vi "minimal_test_startup.vi"   [LabVIEW 2013, in "main.lvlib"]
uses:
  main.lvlib
  Controls/Enum Variables.ctl
  Controls/Enum Save Action Events.ctl
  Controls/Enum Paper Action Events.ctl
  Controls/Enum Process Data.ctl
  Controls/Enum DICOM.ctl
  Controls/Enum User Events.ctl
  New Design/Controls/Reference AE Control.ctl
  Controls/SaveDataCluster.ctl
  Controls/Combobox Filename.ctl
  <vilib>/Utility/error.llb/DialogTypeEnum.ctl
  Components/TypeDef - SHIFTER.ctl
  New Design/Menu/Top Menu.vi
  New Design/Profile/Profile.vi
  New Design/Configuration/Configuration.vi
  New Design/Acquisition/Acquisition.vi
  New Design/Data/Data.vi
  New Design/Journal/Journal.vi
  <userlib>/_MGI/Error Handling/MGI Suppress Error Code/MGI Suppress Error Code (Scalar).vi
  Acquisition/RefData(SubVI).vi
  Globals/DataPathGlobalVariable.vi
  <userlib>/_OpenG.lib/file/file.llb/File Exists - Scalar__ogtk.vi
  Globals/DataAcqRecordPathGlobal.vi
  <vilib>/Utility/file.llb/Write To Spreadsheet File (string).vi
  <userlib>/_OpenG.lib/error/error.llb/Filter Error Codes (Array)__ogtk.vi
  <vilib>/Utility/file.llb/Read From Spreadsheet File (DBL).vi
  <vilib>/Utility/file.llb/Write To Spreadsheet File (DBL).vi
  <vilib>/Utility/file.llb/Read From Spreadsheet File (string).vi
  <userlib>/_OpenG.lib/file/file.llb/Valid Path - Traditional__ogtk.vi
  <vilib>/regexp/Match Regular Expression.xnode
  Components/Dependencies.llb/TLB_Dependencies.lvlib
  Settings/Options/Options.vi
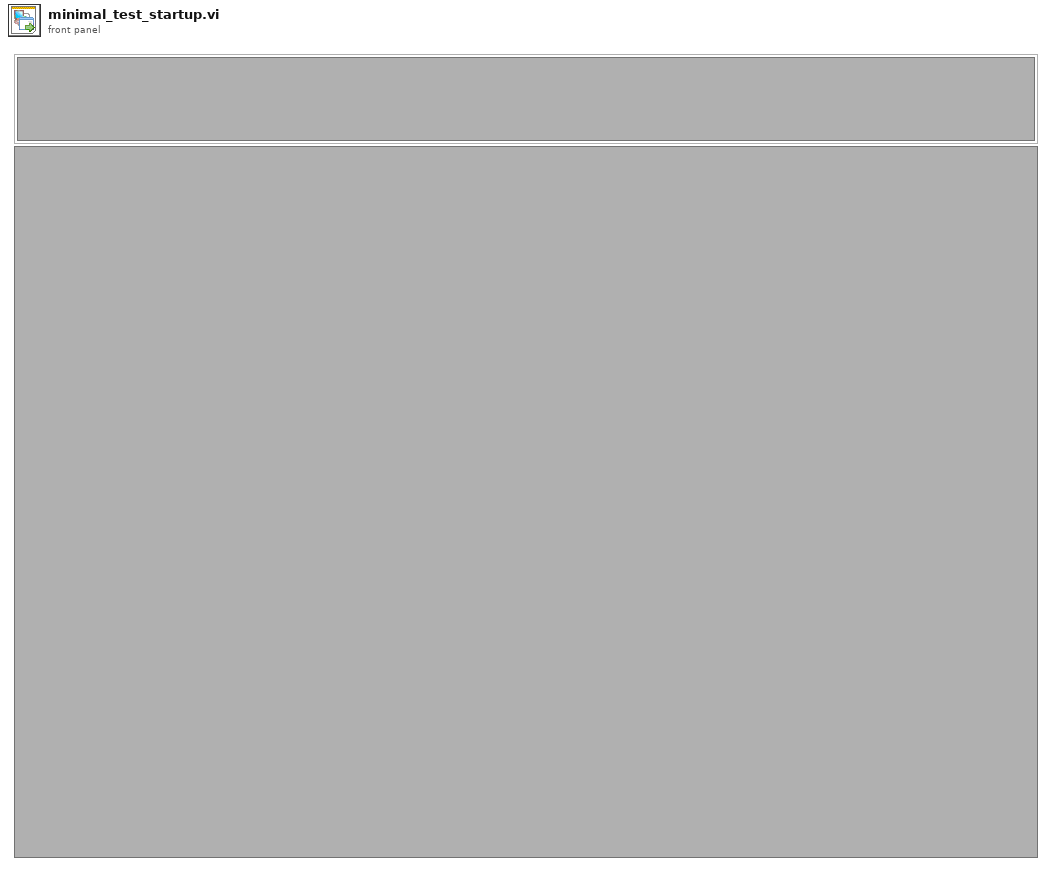
[diagram p1: front panel]
types:
  T1 = enum16{"Clear SR", "Set Display", "Set Shifter", "Initialize Events", "Init Q"}
  T2 = enum32{"Invalid", "Standard", "Closed", "Hidden", "Minimized", "Maximized"}
  T3 = typedef "main.lvlib/TypeDef - SHIFTER.ctl" = cluster{"Exit Event":T4, "Terminate Error":errorcluster, "User Parameter Controls":refnum<vi>[], "User Parameters":cluster{"Name":string, "CPR Number":string, "Measuring Type ":string, "Measuring Technique":string, "Measuring Limb":string, "Operator":string, "Doctor":string, "Comment":string, "AdditionalInfo":string, "RightArm":string[][], "LeftArm":string[][], "PalpationRight":string, "PalpationLeft":string, "Puls":dbl, "Temp One":dbl, "Temp Two":dbl, "ActivityBox":bool}, "System Parameters":cluster{"Paper Running?":bool, "GraphSelection":bool, "Date":string, "Active Page":string}, "Data Acquisition":cluster{"Acquisition":bool, "DAQmx Task":refnum<k21>, "DAQmx Error":errorcluster, "Record number":dbl, "RecordPath":path, "AcqDataRef":refnum<vi>, "Duration":timestamp, "Queue":refnum<queue>, "Control?":bool, "RelativeRecordPath":path}, "Reference signal":cluster{"DAQmx  Task ":refnum<k21>, "Monitor":bool, "Events":dbl, "Time":timestamp, "NullEvents":dbl, "RefDataRef":refnum<vi>, "Queue":refnum<queue>}, "Data Process":cluster{"SubpanelRef":refnum<vi>, "ActiveItemTag":string, "Queue":refnum<queue>}, "System Parameter Controls":refnum<vi>[], "Database":cluster{"PatientdataRef":refnum<file>, "PatientdataPath":path, "Blue Pressure":dbl, "Red Pressure":dbl, "ActiveItemTag":string, "Height Adjustment":dbl, "BluePositionArray":dbl[][], "RedPositionArray":dbl[][], "JournalPath":path}, "MWL":cluster{"PatientID":string, "Name":string, "DICOM Info":path, "DICOM Variables":string[], "Worklist":string[][]}, "Control":cluster{"Queue":refnum<queue>, "SignalCluster":cluster{"Pump":bool, "Finger":bool, "Ankle":bool, "Fast Def":bool, "Slow Def":bool, "Init Cal":bool, "Table Pres":bool, "Table":bool}}, "PageMenu":cluster{"VI Reference":refnum<vi>, "Queue":refnum<queue>}, "Profile":cluster{"VI Reference":refnum<vi>, "Queue":refnum<queue>}, "Configuration":cluster{"VI Reference":refnum<vi>, "Queue":refnum<queue>}, "Acquisition":cluster{"VI Reference":refnum<vi>, "Queue":refnum<queue>}, "Data":cluster{"VI Reference":refnum<vi>, "Queue":refnum<queue>}, "Journal":cluster{"VI Reference":refnum<vi>, "Queue":refnum<queue>}, "cRef":T5, "Bluetooth":cluster{"Queue":refnum<queue>, "VI Reference":refnum<vi>}}
  T4 = typedef "main.lvlib/TLB_Dependencies.lvlib/Exit Event Ref.ctl" = refnum<user-event>
  T5 = typedef "main.lvlib/Reference Cluster.ctl" = cluster{"Menu":cluster{"References":cluster{"Stop Acq":refnum<vi>, "MenuExit":refnum<vi>, "MenuStartADC":refnum<vi>, "PersonalInfoString":refnum<vi>, "Profile":refnum<vi>, "Configuration":refnum<vi>, "Acquisition":refnum<vi>, "Data":refnum<vi>, "Journal":refnum<vi>}}, "Profile":cluster{"References":cluster{"Search Patient ID":refnum<vi>, "Name":refnum<vi>, "CommentStr":refnum<vi>, "Listbox Patient ID":refnum<vi>, "ListboxDoctor":refnum<vi>, "ListboxOperator":refnum<vi>, "HospitalName":refnum<vi>, "HospitalDepartment":refnum<vi>, "HospitalAddress":refnum<vi>, "EditHospInfo":refnum<vi>, "Add Patient ID Btn":refnum<vi>, "Query Worklist":refnum<vi>}}, "Configuration":cluster{"References":cluster{"ListboxMeasurementArea":refnum<vi>, "ListboxMeasurementTechnique":refnum<vi>, "ListboxMeasurementMeth":refnum<vi>, "ListboxRightSegmentNr":refnum<vi>, "ListboxLeftSegmentNr":refnum<vi>, "HeightAdjustmentInt":refnum<vi>, "PalpationRight":refnum<vi>, "PalpationLeft":refnum<vi>, "ActivityBox":refnum<vi>}, "New method":cluster{"AddNewMeasurementBtn":refnum<vi>, "Left Time Table":refnum<vi>, "Right Time Table":refnum<vi>}, "Old method":cluster{"LeftArmPressureTable":refnum<vi>, "RightArmPressureTable":refnum<vi>, "SaveArmPressureBtn":refnum<vi>, "Puls":refnum<vi>, "TempTwo":refnum<vi>, "TempOne":refnum<vi>}, "Method":string}, "Acquisition":cluster{"References":cluster{"SegmentAcqString":refnum<vi>, "RingActGraph":refnum<vi>}}, "Data":cluster{"References":cluster{"cmString":refnum<vi>, "AdjustedHeight":refnum<vi>, "Menu":refnum<vi>, "Tangent On/Off":refnum<vi>, "FilterControl":refnum<vi>}}, "Journal":cluster{"References":cluster{"ReportSelection":refnum<vi>, "Data":refnum<vi>, "GenerateReport":refnum<vi>, "Menu":refnum<vi>, "Send To PACS":refnum<vi>}}}
  T6 = typedef "main.lvlib/TLB_Dependencies.lvlib/amc_Message Queue.ctl" = refnum<queue>
  T7 = typedef "main.lvlib/Enum Variables.ctl" = enum16{"SetAcqFilter", "GetAcqFilter", "Set Filter", "Get Filter", "Set Height", "Get Height", "Set Blue Pressure", "Get Blue Pressure", "Set Red Pressure", "Get Red Pressure", "Init", "Reset Pressure", "Set Red Cursors", "Get Red Cursors", "Set Blue Cursors", "Get Blue Cursors", "Set Language", "Get Language", "Set Active Graphs", "Get ActiveGraphs", "Set Method", "Get Method", "Set Encryption", "Get Encryption", "Set ExcelVersion", "Get ExcelVersion", "Set DICOM Avail", "Get DICOM Avail", "Set DICOM Encode", "Get DICOM Encode", "Set JournalExport", "Get JournalExport", "Set Sequence", "Get Sequence", "Set DAQ Connected", "Get DAQ Connected", "Set Current Graph", "Get Current Graph", "Set General Settings", "Get Hyphenation", "Set Arm Calc Method", "Get Arm Calc Method", "Set Dicom Tags", "Get Dicom Tags", "Set BT Serial", "Get BT Serial", "Set BT Accepted Serials", "Get BT Accepted Serials", "Get BT License", "Set BT License"}
  T8 = typedef "main.lvlib/Enum Save Action Events.ctl" = enum16{"LoadReportPath", "SaveReportPath", "Load Graph Path", "Save Graph Path", "LoadDataPath", "SaveDataPath", "Load Template Path", "Save Template Path", "Load PressureFactor", "Save PressureFactor", "Init", "Load Listbox", "Save Listbox", "LoadHospInfo", "SaveHospInfo", "Load DICOM Activation", "Save DICOM Activation", "LoadDICOMInfoWL", "SaveDICOMInfoWL", "LoadDICOMInfoPACS", "SaveDICOMInfoPACS", "Load ArmCalcMethod", "Save ArmCalcMethod", "LoadItemTags", "SaveItemTags", "LoadDICOMEncoding", "SaveDICOMEncoding", "LoadJournalType", "SaveJournalType", "LoadAcqFilterType", "SaveAcqFilterType", "Load Sequence", "Save Sequence", "Load Acquisition Mode", "Save Acquisition Mode", "Load General Settings", "Save General Settings", "Load Language", "Save Language", "Load Dicom Tags", "Save Dicom Tags", "Load BT Serial", "Save BT Serial", "Load BT License", "Save BT License"}
  T9 = typedef "LVPoint32TypeDef.ctl" = cluster{"Horizontal":i32, "Vertical":i32}
  T10 = typedef "LVRowAndColumnTypeDef.ctl" = cluster{"Row":i32, "Column":i32}
  T11 = typedef "eventvkey.ctl" = enum16{"ASCII", "Enter", "Return", "Shift", "Ctrl", "Alt", "Cmd", "Opt", "Caps", "NumLock", "Clear", "Break", "Up", "Down", "Left", "Right", "Insert", "Delete", "Home", "End", "PageUp", "PageDown", "Escape", "Help", "Pause", "ScrollLock", "F1", "F2", "F3", "F4", "F5", "F6", "F7", "F8", "F9", "F10", "F11", "F12", "F13", "F14", "F15", "F16", "F17", "F18", "F19", "F20", "F21", "F22", "F23", "F24", "Play", "VolumeUp", "VolumeDown", "Mute", "Two Byte Char"}
  T12 = typedef "main.lvlib/Enum Paper Action Events.ctl" = enum16{"Paper State", "Init"}
  T13 = typedef "main.lvlib/Enum Process Data.ctl" = enum16{"Init", "Set Cursor Mode", "Set Data Path", "Get All"}
  T14 = typedef "main.lvlib/Enum DICOM.ctl" = enum16{"Set DICOM itemTags", "Set Dicom Encoding", "Set DICOM Attributes"}
  T15 = typedef "main.lvlib/Reference AE Control.ctl" = enum16{"Initialize", "Set Menu", "Set Profile", "Set Configuration", "Set Configuration_old", "Set Configuration_new", "Set Configuration Method", "Set Acquisition", "Set Data", "Set Journal", "Get"}
  T16 = typedef "main.lvlib/Enum User Events.ctl" = enum16{"User Event", "Init"}
  T17 = typedef "main.lvlib/SaveDataCluster.ctl" = cluster{"HospInfo":cluster{"Name":string, "Address":string, "Department":string}, "Pressure":cluster{"Pressure":dbl}, "DataPath":cluster{"DataPath":path}, "ReportPath":cluster{"Path":path, "Name":string}, "DICOM Info WL":cluster{"port":i32, "AEtitle":string, "host":string, "remoteAE":string}, "DICOM Info PACS":cluster{"port":i32, "AEtitle":string, "host":string, "remoteAE":string}, "ArmCalcMethod":dbl, "itemTags":string[], "DicomEncoding":u16, "JournalType":u16, "General Settings":cluster{"Hyphenation":bool, "Language":u16, "CellStr1":string, "CellStr2":string}, "Dicom Tags":string[][], "BT Serial":cluster{"Serial Number":string, "Side":string, "Ignore?":bool}[], "BT License":cluster{"License":string, "Accepted Serials":string[]}}
  T18 = typedef "main.lvlib/Combobox Filename.ctl" = string
  T19 = enum16{"leave excel open after last close", "close only if opened by LabVIEW", "close excel after last close"}
  T20 = cluster{"sys":dbl, "dia":dbl, "puls":dbl, "date":string, "time":string, "code":string, "serial":string, "temp":dbl, "activity":string}
  T21 = cluster{"name":string, "department":string, "address":string}
  T22 = cluster{"id":string, "name":string, "operator":string, "doctor":string, "comment":string}
  T23 = typedef "DialogTypeEnum.ctl" = enum16{"no dialog", "OK message", "continue or stop message", "auto error handling dialog", "OK message + warnings", "continue/stop + warnings"}
  T24 = cluster{"port":i32, "AEtitle":string, "host":string, "remoteAE":string}
  T25 = cluster{"Search Patient ID":refnum<vi>, "Name":refnum<vi>, "CommentStr":refnum<vi>, "Listbox Patient ID":refnum<vi>, "ListboxDoctor":refnum<vi>, "ListboxOperator":refnum<vi>, "HospitalName":refnum<vi>, "HospitalDepartment":refnum<vi>, "HospitalAddress":refnum<vi>, "EditHospInfo":refnum<vi>, "Add Patient ID Btn":refnum<vi>, "Query Worklist":refnum<vi>}
  T26 = cluster{"Name":refnum<vi>, "ListboxOperator":refnum<vi>, "ListboxDoctor":refnum<vi>, "CommentStr":refnum<vi>, "Name":string, "Operator":string, "Doctor":string, "Comment":string}
  T27 = cluster{"Hospital Name 2":string, "Hospital Address 2":string, "Department 2":string}
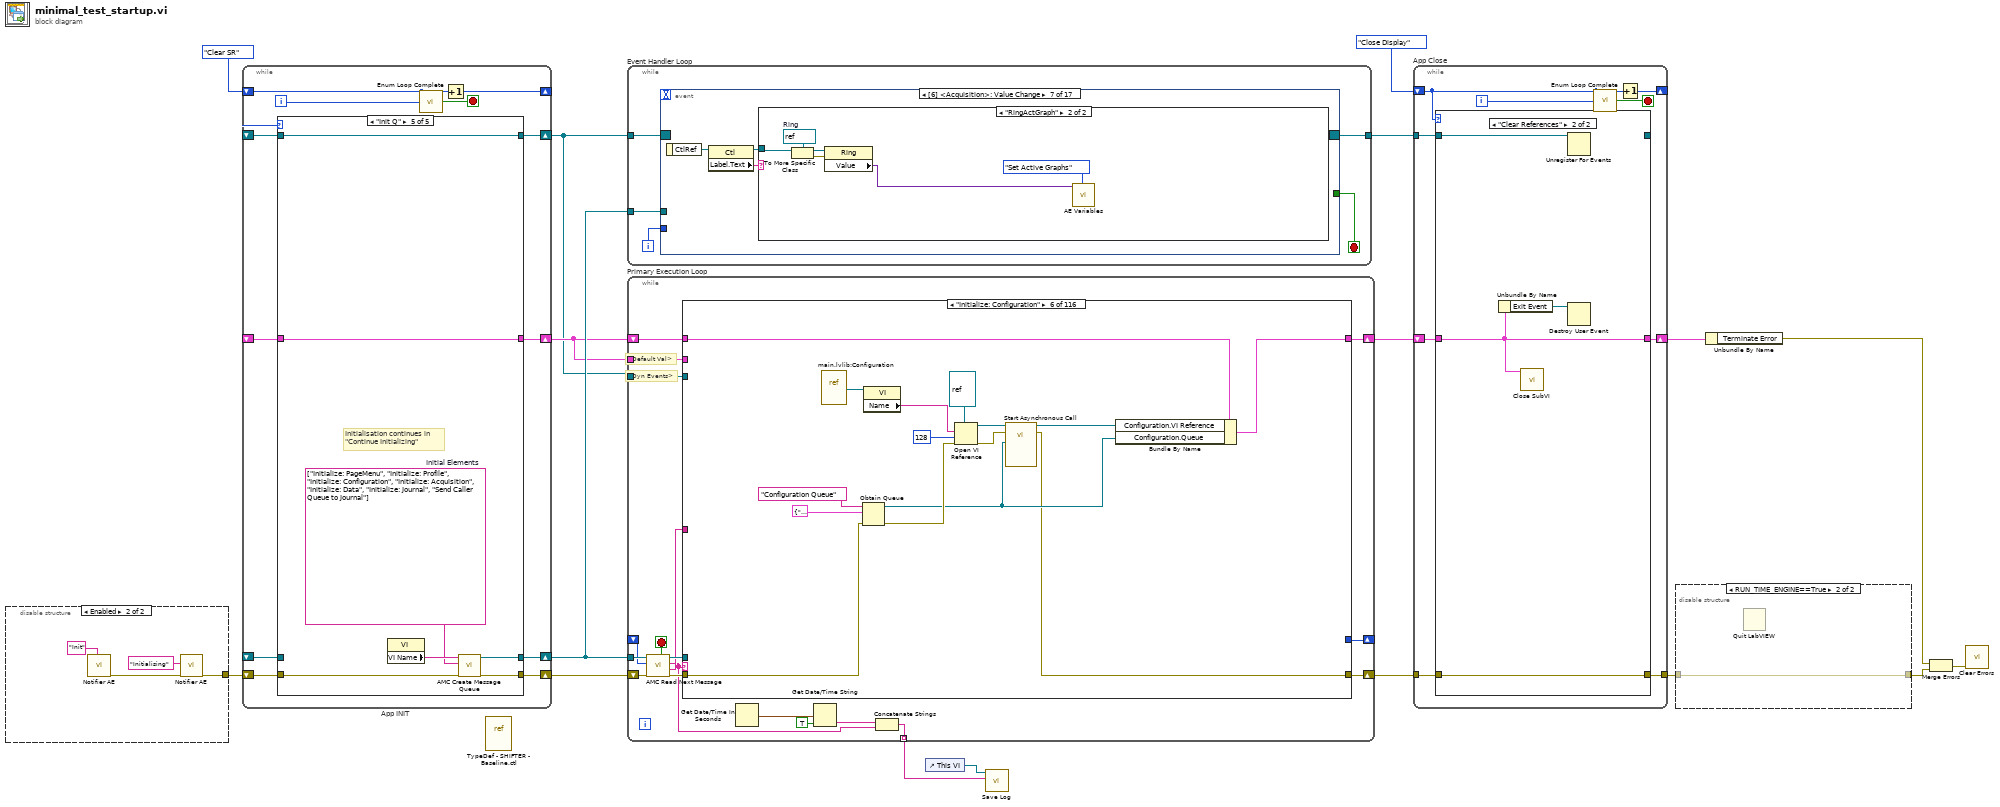
[diagram p0: block diagram]
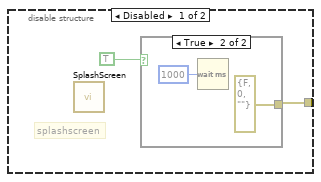
[diagram p2: hidden frame]
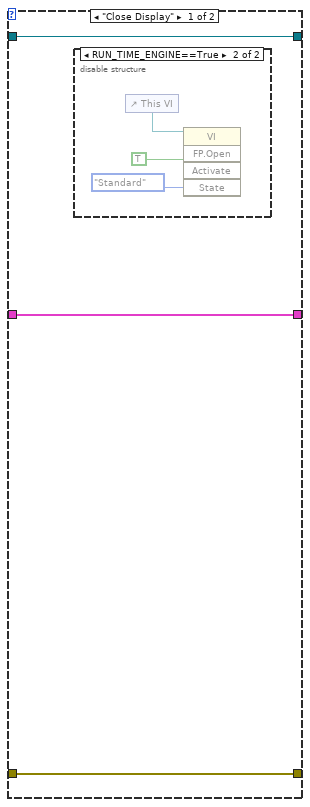
[diagram p5: hidden frame]
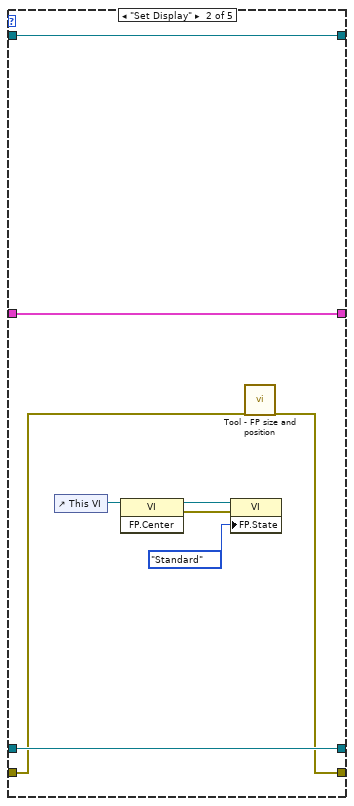
[diagram p8: hidden frame]
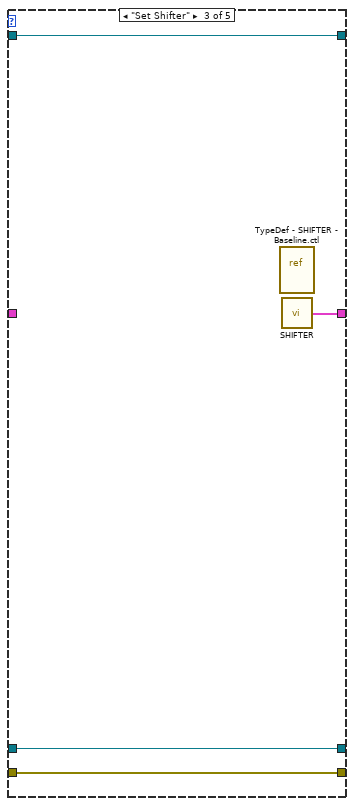
[diagram p9: hidden frame]
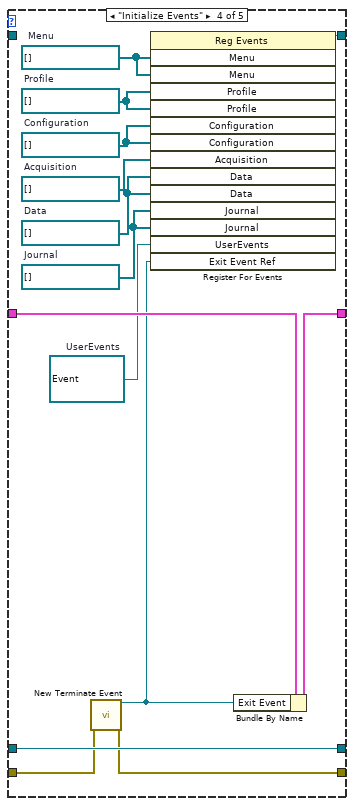
[diagram p10: hidden frame]
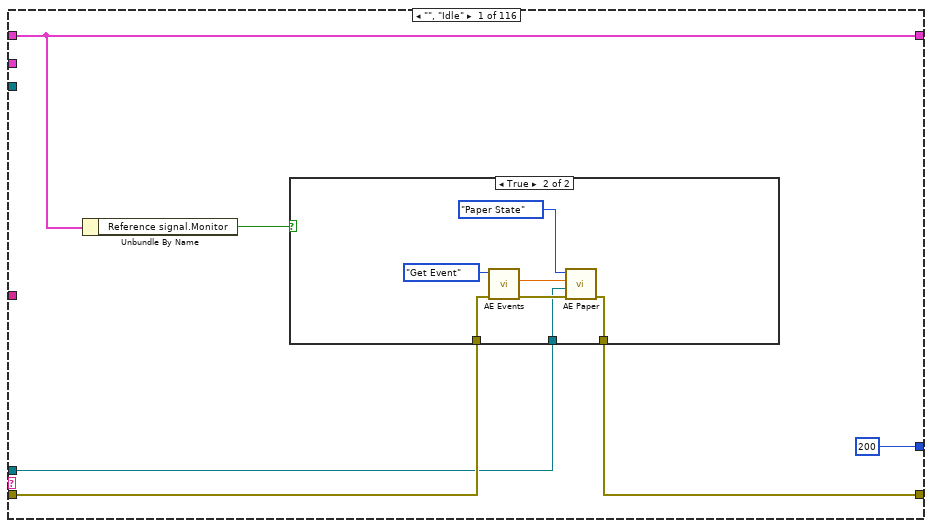
[diagram p11: hidden frame]
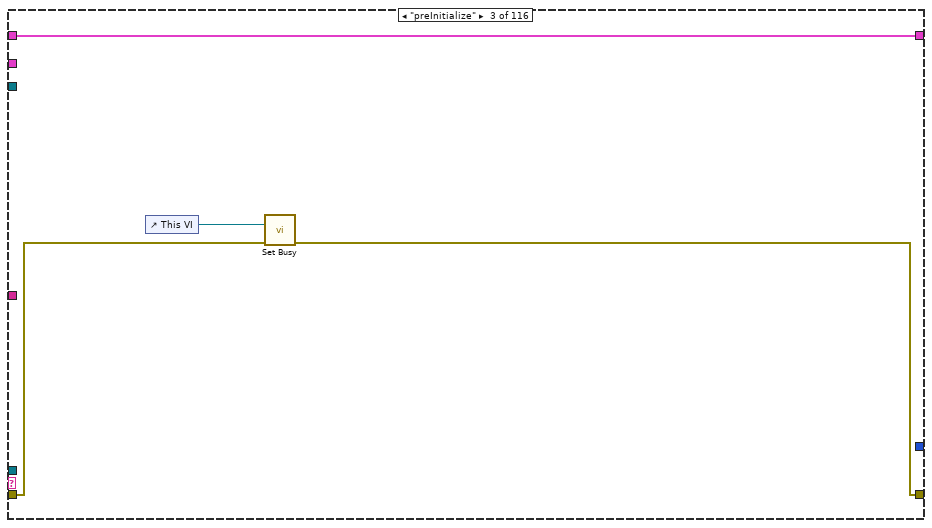
[diagram p14: hidden frame]
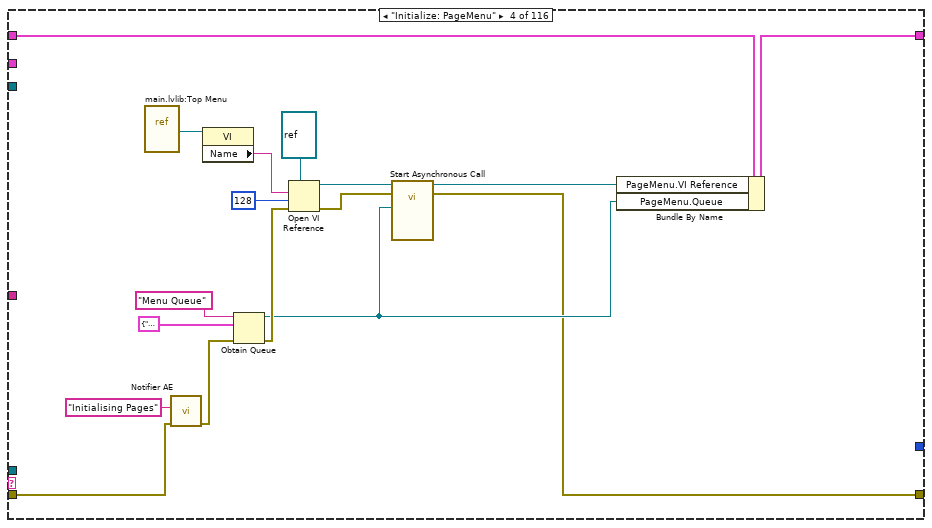
[diagram p15: hidden frame]
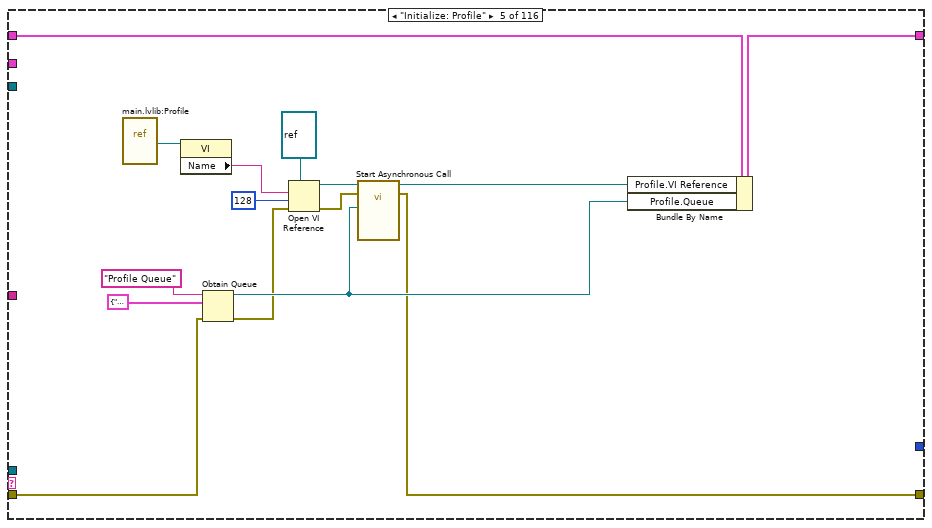
[diagram p16: hidden frame]
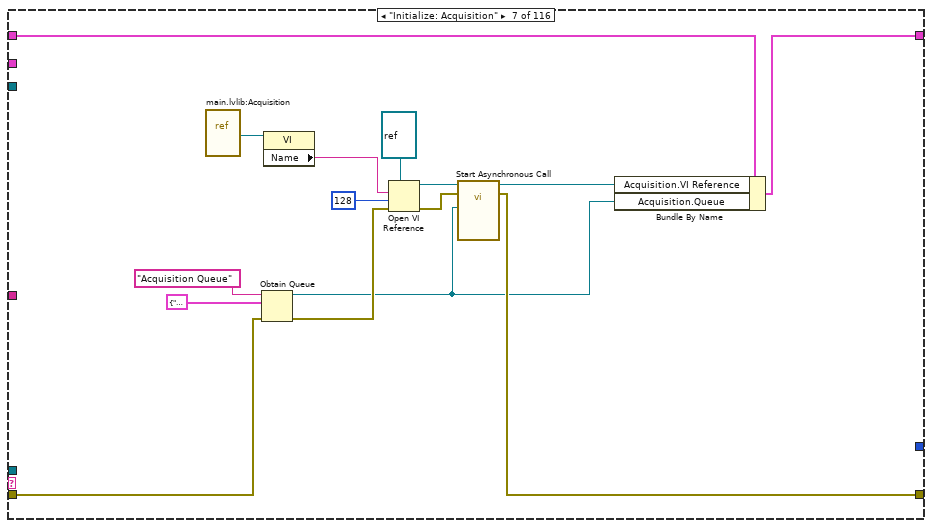
[diagram p17: hidden frame]
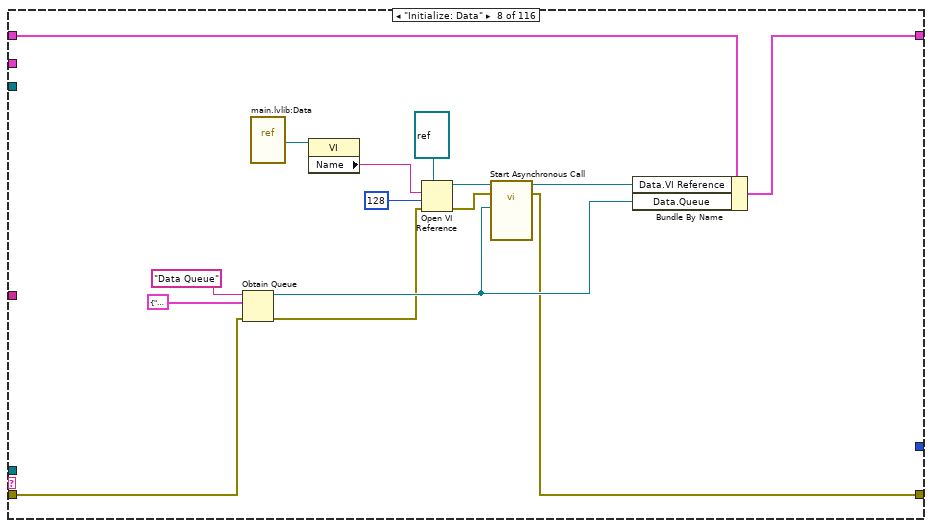
[diagram p18: hidden frame]
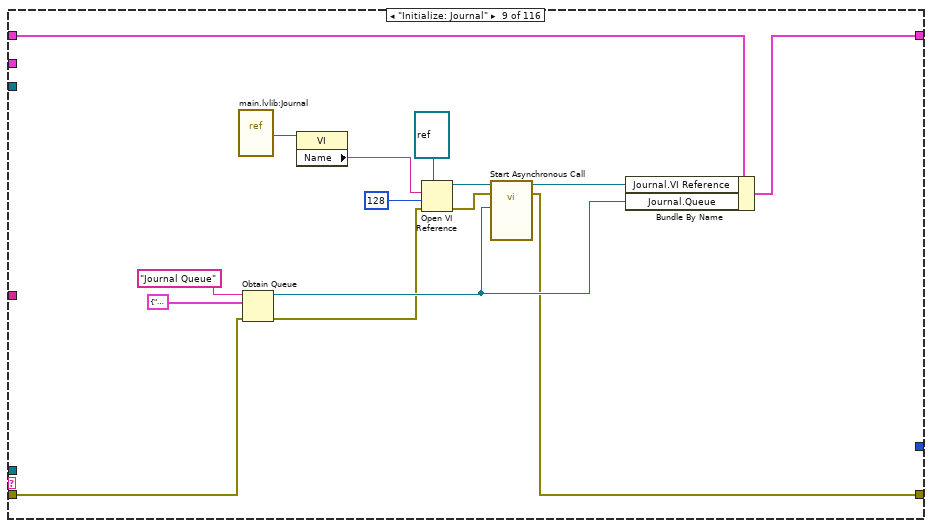
[diagram p19: hidden frame]
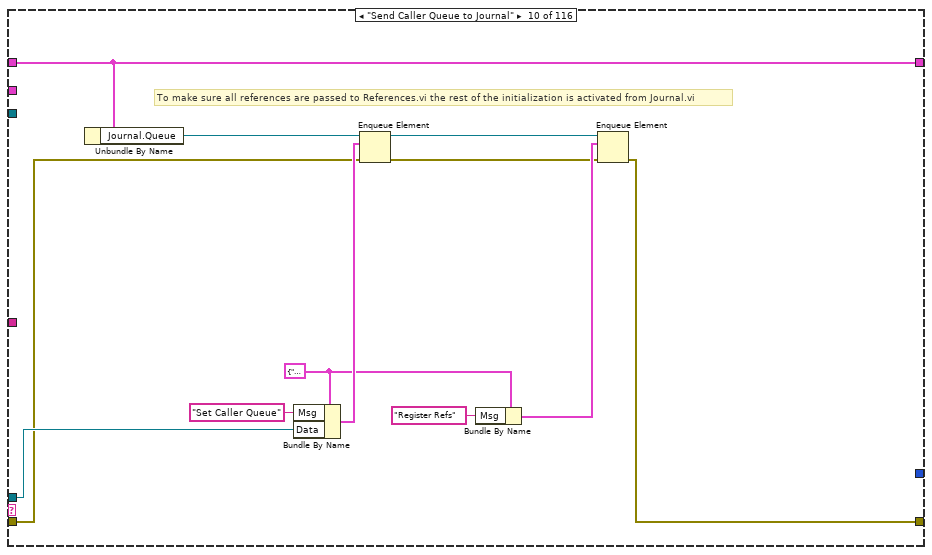
[diagram p20: hidden frame]
diagram:
  n1 = disable-structure shown="Enabled" {
    disable-tunnel: [w18 w23] -> w3
    frame Disabled {
      # "splashscreen"
      n2 = call "SplashScreen.vi"() -> ()  [unwired: 11 in, 1 out]
      n3 = case shown="True" TRUE {
        tunnel: [_ errorcluster {"status"=FALSE, "code"=0, "source"=""} ("error out")] -> w18
        frame False {
        }
        frame True {
          n4 = Wait (ms)(milliseconds to wait=u32 1000) -> ()  [unwired: 1 out]
        }
      }
    }
    frame Enabled {
      n5 = call "Notifier AE.vi"("Cmd"="Init") -> ("error out"=w24:errorcluster)  [unwired: 10 in]
      n6 = call "Notifier AE.vi"("error in (no error)"=w24, "String"="Initialising") -> ("error out"=w23:errorcluster)  [unwired: 9 in]
    }
  }
  n7 = while "App INIT" {
    shift-right: [w31] -> _
    shift-left: T1."Clear SR" -> [w26]
    shift-right: [w37] -> w7
    shift-left: _ -> [w30]
    shift-right: [w34] -> w12
    shift-left: w3 -> [w29]
    shift-right: [w36] -> w5
    shift-left: _ -> [w28]
    shift-right: [w35] -> w6
    shift-left: _ -> [w27]
    i -> [w32]
    stop <- w33 stop-if-true
    n8 = case shown="\"Init Q\"" w26 {
      tunnel: [_ w44 w49 w64 w68] -> w37
      tunnel: [_ w43 w48 w59 w66] -> w34
      tunnel: [_ w46 w50 w62 w70] -> w35
      tunnel: [_ w45 w47 w61 w71] -> w36
      tunnel: w30 -> [_ w44 w49 w64 _]
      tunnel: w29 -> [_ w42 w48 w60 w67]
      tunnel: w28 -> [_ w45 w47 _ w71]
      tunnel: w27 -> [_ w46 _ w63 w70]
      frame "Clear SR" {
      }
      frame "Set Display" {
        n9 = control-ref of="This VI"() -> (w40:refnum<vi>)
        n10 = invoke class="VI" method="FP.Center"(reference=w40) -> (reference out=w39:refnum<vi>, error out=w38:errorcluster)  [unwired: 2 in, 1 out]
        n11 = property class="VI"(reference=w39, error in=w38, "FP.State"=T2."Standard" ("Front Panel Window:State")) -> ()  [unwired: 2 out]
        n12 = call "Tool - FP size and position.vi"("error in (no error)"=w42) -> ("error out"=w43:errorcluster)  [unwired: 7 in, 11 out]
      }
      frame "Set Shifter" {
        n13 = vi-ref "TypeDef - SHIFTER - Baseline.ctl"() -> ()  [unwired: 1 out]
        n14 = call "SHIFTER.vi"() -> ("SHIFTER DATA"=w50:T3)  [unwired: 15 out]
      }
      frame "Initialize Events" {
        w53 = refnum<vi>[] []  # Journal
        w54 = refnum<vi>[] []  # Data
        w55 = refnum<vi>[] []  # Acquisition
        w56 = refnum<vi>[] []  # Configuration
        w52 = refnum<user-event> refnum  # UserEvents
        w57 = refnum<vi>[] []  # Profile
        w58 = refnum<vi>[] []  # Menu
        n15 = call "New Terminate Event.vi"("error in (no error)"=w60) -> ("Exit Event Ref"=w51:T4, "error out"=w59:errorcluster)  [unwired: 13 in]
        n16 = register-events(w58, w58, w57, w57, w56, w56, w55, w54, w54, w53, w53, w52, w51) -> (reference out=w61:refnum<event-registration>)  [unwired: 2 in, 1 out]
        n17 = Bundle By Name(cluster=w63, "Exit Event"=w51) -> (w62:T3)
      }
      frame "Init Q" {
        w65 = string[] ["Initialize: PageMenu", "Initialize: Profile", "Initialize: Configuration", "Initialize: Acquisition", "Initialize: Data", "Initialize: Journal", "Send Caller Queue to Journal"]  # Initial Elements
        # "Initialisation continues in \n\"Continue Initializing\""
        n18 = property class="VI"() -> ("VI Name"=w69:string)  [unwired: 2 in, 2 out]
        n19 = call "AMC Create Message Queue.vi"("error in (no error)"=w67, "Initial Message Names"=w65, "Message Queue Name"=w69) -> ("error out"=w66:errorcluster, "Message Queue out"=w68:T6)  [unwired: 7 in]
      }
    }
    n20 = call "Enum Loop Complete.vi"("Current State Enum"=w26, "Itteration"=w32) -> ("Loop Complete?"=w33:bool)  [unwired: 13 out]
    n21 = Increment(x=w26) -> (x+1=w31:T1)
  }
  n22 = vi-ref "TypeDef - SHIFTER - Baseline.ctl"() -> ()  [unwired: 1 out]
  n23 = while "Event Handler Loop" {
    tunnel: w5 -> [w75]
    tunnel: w7 -> [w74]
    tunnel: [w73] -> w15
    i -> [w72]
    stop <- w76 stop-if-true
    n24 = event shown="[6] <Acquisition>: Value Change" {
      selector: w75 -> [_ _ _ _ _ _ _ _ _ _ _ _ _ _ _ _ _]
      dyn-events: [_ _ _ _ _ _ _ _ _ _ _ _ _ _ _ _ _] -> w73
      timeout: _ -> [_ _ _ _ _ _ _ _ _ _ _ _ _ _ _ _ _]
      tunnel: [_ _ _ _ _ _ _ _ _ _ _ _ TRUE ("NewVal") TRUE ("NewVal") _ w290 _] -> w76
      tunnel: w74 -> [w80 _ w106 w124 w155 _ _ w179 w191 w207 w219 w236 w267 w268 w272 w291 _]
      tunnel: w72 -> [_ _ _ _ _ _ _ _ _ _ _ _ _ _ _ _ _]
      event Value Change {
        n25 = event-data() -> ("CtlRef"=w82:refnum<vi>)  [unwired: 1 out]
        n26 = property class="Ctl"(reference=w82) -> (reference out=w77:refnum<vi>, "Label.Text"=w81:string)  [unwired: 1 in, 1 out]
        n27 = call "AMC Send Local Message.vi"("Message Name"="Cache User Parameters", "Message Queue in"=w80) -> ("Message Queue out"=w79:T6)  [unwired: 8 in, 1 out]
        n28 = case shown="\"Acquisition\"" w81 {
          tunnel: w79 -> [_ w84 w85 w87 w89 w91 w97 w102 w105]
          tunnel: w77 -> [_ _ _ _ _ _ w96 _ _]
          frame "", Default {
          }
          frame "Profile" {
            n29 = call "AMC Send Local Messages.vi"("Message Names"=string[] ["Subpanel: Load Profile"], "Message Queue in"=w84) -> ()  [unwired: 8 in, 2 out]
          }
          frame "Configuration" {
            n30 = call "AMC Send Local Messages.vi"("Message Names"=string[] ["Subpanel: Load Configuration"], "Message Queue in"=w85) -> ()  [unwired: 8 in, 2 out]
          }
          frame "Acquisition" {
            n31 = call "AMC Send Local Messages.vi"("Message Names"=string[] ["Update Display", "Subpanel: Load Acquisition", "Send Segment to Acquisition"], "Message Queue in"=w87) -> ()  [unwired: 8 in, 2 out]
          }
          frame "Data" {
            n32 = call "AMC Send Local Messages.vi"("Message Names"=string[] ["Subpanel: Load Data"], "Message Queue in"=w89) -> ()  [unwired: 8 in, 2 out]
          }
          frame "Journal" {
            n33 = call "AMC Send Local Messages.vi"("Message Names"=string[] ["Subpanel: Load Journal"], "Message Queue in"=w91) -> ()  [unwired: 8 in, 2 out]
          }
          frame "MenuStartADC" {
            n34 = property class="Ctl"(reference=w96) -> ("Value"=w95:variant)  [unwired: 1 in, 2 out]
            n35 = Variant To Data(type=TRUE, Variant=w95) -> (data=w93:bool)  [unwired: 1 in, 1 out]
            n36 = case shown="True" w93 {
              tunnel: w97 -> [w98 w100]
              frame False {
                n37 = call "AMC Send Local Messages.vi"("Message Names"=string[] ["Stop Reference", "Update Display", "", "", ""], "Message Queue in"=w98) -> ()  [unwired: 8 in, 2 out]
              }
              frame True {
                n38 = call "AMC Send Local Messages.vi"("Message Names"=string[] ["Query DAQ Availability", "SavePatientDataOnDate"], "Message Queue in"=w100) -> ()  [unwired: 8 in, 2 out]
              }
            }
          }
          frame "Stop Acq" {
            n39 = call "AMC Send Local Messages.vi"("Message Names"=string[] ["Stop Reference", "Update Display", "", "", ""], "Message Queue in"=w102) -> ()  [unwired: 8 in, 2 out]
          }
          frame "MenuExit" {
            n40 = call "AMC Send Local Message.vi"("Message Name"="Exit", "Message Queue in"=w105) -> ()  [unwired: 8 in, 2 out]
          }
        }
      }
      event Shortcut Menu Selection (User) {
        n41 = event-data() -> ()  [unwired: 6 out]
      }
      event Value Change {
        n42 = event-data() -> ("CtlRef"=w108:refnum<vi>)  [unwired: 1 out]
        n43 = property class="Ctl"(reference=w108) -> ("Label.Text"=w107:string)  [unwired: 1 in, 2 out]
        n44 = case shown="\"Listbox Patient ID\"" w107 {
          tunnel: w106 -> [_ w109 w111 w114 w115 w117 w119]
          frame "", Default {
          }
          frame "Search Patient ID" {
            n45 = call "AMC Send Local Message.vi"("Message Name"="FindCprNumber", "Message Queue in"=w109) -> ()  [unwired: 8 in, 2 out]
          }
          frame "CommentStr", "ListboxDoctor", "ListboxOperator", "Name" {
            n46 = call "AMC Send Local Messages.vi"("Message Names"=string[] ["Cache User Parameters", "SavePatientData", "Update Display", "DCM: Update Variables"], "Message Queue in"=w111) -> ()  [unwired: 8 in, 2 out]
          }
          frame "Listbox Patient ID" {
            n47 = call "AMC Send Local Messages.vi"("Message Names"=string[] ["ResetToDefault", "LoadNameCpr", "Cache User Parameters", "SelectCpr", "DCM: Load DICOM Info", "DCM: Update Variables", "Load Armpressure"], "Message Queue in"=w114) -> ()  [unwired: 8 in, 2 out]
          }
          frame "EditHospInfo" {
            n48 = call "AMC Send Local Message.vi"("Message Name"="EditHospInfo", "Message Queue in"=w115) -> ()  [unwired: 8 in, 2 out]
          }
          frame "Add Patient ID Btn" {
            n49 = call "AMC Send Local Messages.vi"("Message Names"=string[] ["AddCpr", ""], "Message Queue in"=w117) -> ()  [unwired: 8 in, 2 out]
          }
          frame "Query Worklist" {
            n50 = call "AMC Send Local Messages.vi"("Message Names"=string[] ["MWL: QueryWorklist", "MWL: PatientID", "ResetToDefault", "LoadNameCpr", "Cache User Parameters", "MWL: Update Data", "SelectCpr"], "Message Queue in"=w119) -> ()  [unwired: 8 in, 2 out]
          }
        }
      }
      event Shortcut Menu Selection (User) {
        n51 = event-data() -> ("CtlRef"=w123:refnum<vi>, "ItemTag"=w122:string, "Coords"=w121:T9)  [unwired: 3 out]
        n52 = case shown="\"Add New\"" w122 {
          tunnel: w124 -> [_ w129 w145 w152]
          tunnel: w123 -> [_ w128 w144 w151]
          tunnel: w121 -> [_ w125 w141 _]
          frame "False", Default {
          }
          frame "DeleteID" {
            w127 = refnum<vi> refnum  # ListBox
            n53 = To More Specific Class(target class=w127, reference=w128) -> (specific class reference=w126:refnum<vi>)  [unwired: 1 in, 1 out]
            n54 = invoke class="LstBox" method="Point To Row"(reference=w126, "Point"=w125) -> (reference out=w133:refnum<vi>, "Row"=w131:i32)  [unwired: 5 in, 5 out]
            n55 = property class="LstBox"(reference=w133) -> ("Item Names"=w132:string[])  [unwired: 1 in, 2 out]
            n56 = Index Array(array=w132, index=w131) -> (element=w130:string)
            n57 = call "AMC Send Local Message.vi"("Message Value"=w130, "Message Name"="RemoveCpr", "Message Queue in"=w129) -> ()  [unwired: 7 in, 2 out]
          }
          frame "Delete" {
            w143 = refnum<vi> refnum  # ListBox
            n58 = To More Specific Class(target class=w143, reference=w144) -> (specific class reference=w142:refnum<vi>)  [unwired: 1 in, 1 out]
            n59 = invoke class="LstBox" method="Point To Row"(reference=w142, "Point"=w141) -> (reference out=w140:refnum<vi>, "Row"=w139:i32)  [unwired: 5 in, 5 out]
            n60 = property class="LstBox"(reference=w140) -> ("Label.Text"=w137:string)  [unwired: 1 in, 2 out]
            n61 = Number To Decimal String(number=w139) -> (decimal integer string=w135:string)  [unwired: 1 in]
            n62 = Concatenate Strings("Delete: ", w137) -> (w136:string)
            n63 = call "AMC Send Local Message.vi"("Message Value"=w135, "Message Name"=w136, "Message Queue in"=w145) -> ()  [unwired: 7 in, 2 out]
          }
          frame "Add New" {
            w150 = refnum<vi> refnum  # ListBox
            n64 = To More Specific Class(target class=w150, reference=w151) -> (specific class reference=w146:refnum<vi>)  [unwired: 1 in, 1 out]
            n65 = property class="LstBox"(reference=w146) -> ("Label.Text"=w148:string)  [unwired: 1 in, 2 out]
            n66 = Concatenate Strings("Add New: ", w148) -> (w147:string)
            n67 = call "AMC Send Local Message.vi"("Message Name"=w147, "Message Queue in"=w152) -> ()  [unwired: 8 in, 2 out]
          }
        }
      }
      event Value Change {
        n68 = event-data() -> ("CtlRef"=w158:refnum<vi>)  [unwired: 1 out]
        n69 = call "AMC Send Local Message.vi"("Message Name"="Cache User Parameters", "Message Queue in"=w155) -> ("Message Queue out"=w154:T6)  [unwired: 8 in, 1 out]
        n70 = property class="Ctl"(reference=w158) -> (reference out=w156:refnum<vi>, "Label.Text"=w157:string)  [unwired: 1 in, 1 out]
        n71 = case shown="\"SaveArmPressureBtn\"" w157 {
          tunnel: w154 -> [_ _ _ _ _ _ w165 _ _ _ _ _ w166 _ _]
          tunnel: w156 -> [_ _ _ w162 _ _ _ _ _ _ _ _ _ _ _]
          frame "False", Default {
          }
          frame "ListboxMeasurementArea" {
          }
          frame "ListboxMeasurementTechnique" {
          }
          frame "ListboxMeasurementMeth" {
            w161 = refnum<vi> refnum  # ListBox
            n72 = To More Specific Class(target class=w161, reference=w162) -> (specific class reference=w160:refnum<vi>)  [unwired: 1 in, 1 out]
            n73 = property class="LstBox"(reference=w160) -> ("Value"=w159:variant)  [unwired: 1 in, 2 out]
            n74 = call "AE Variables.vi"("VariantIn"=w159, "Action"=Enum_Variables."Set Method") -> ()  [unwired: 10 in, 8 out]
          }
          frame "ListboxRightSegmentNr" {
          }
          frame "ListboxLeftSegmentNr" {
          }
          frame "HeightAdjustmentInt" {
            n75 = call "AMC Send Local Message.vi"("Message Name"="Set Height", "Message Queue in"=w165) -> ()  [unwired: 8 in, 2 out]
          }
          frame "TempOne" {
          }
          frame "TempTwo" {
          }
          frame "Puls" {
          }
          frame "RightArmPressureTable" {
          }
          frame "LeftArmPressureTable" {
          }
          frame "SaveArmPressureBtn" {
            n76 = call "AMC Send Local Messages.vi"("Message Names"=string[] ["SaveArmPressure", "SavePalpationData"], "Message Queue in"=w166) -> ()  [unwired: 8 in, 2 out]
          }
          frame "PalpationRight" {
          }
          frame "PalpationLeft" {
          }
        }
      }
      event Shortcut Menu Selection (User) {
        n77 = event-data() -> ("ItemTag"=w168:string)  [unwired: 5 out]
        n78 = case shown="\"True\"" w168 {
          frame "False", Default {
          }
          frame "True" {
          }
        }
      }
      event Value Change {
        n79 = event-data() -> ("CtlRef"=w171:refnum<vi>)  [unwired: 1 out]
        n80 = property class="Ctl"(reference=w171) -> (reference out=w169:refnum<vi>, "Label.Text"=w170:string)  [unwired: 1 in, 1 out]
        n81 = case shown="\"RingActGraph\"" w170 {
          tunnel: w169 -> [_ w176]
          frame "", Default {
          }
          frame "RingActGraph" {
            w175 = refnum<vi> refnum  # Ring
            n82 = To More Specific Class(target class=w175, reference=w176) -> (specific class reference=w174:refnum<vi>, error out=w173:errorcluster)  [unwired: 1 in]
            n83 = property class="Ring"(reference=w174, error in=w173) -> ("Value"=w172:variant)  [unwired: 2 out]
            n84 = call "AE Variables.vi"("VariantIn"=w172, "Action"=Enum_Variables."Set Active Graphs") -> ()  [unwired: 10 in, 8 out]
          }
        }
      }
      event Value Change {
        n85 = event-data() -> ("CtlRef"=w181:refnum<vi>)  [unwired: 1 out]
        n86 = property class="Ctl"(reference=w181) -> (reference out=w178:refnum<vi>, "Label.Text"=w180:string)  [unwired: 1 in, 1 out]
        n87 = case shown="\"FilterControl\"" w180 {
          tunnel: w179 -> [_ w182 w187 w189]
          tunnel: w178 -> [_ w184 _ _]
          frame "", Default {
          }
          frame "ProcessDataTreeMenu" {
            n88 = call "Tree Menu to String.vi"("Control in"=w184) -> ("delimited string"=w183:string)  [unwired: 10 in]
            n89 = Build Array(w183) -> (w185:string[])
            n90 = call "AMC Send Local Messages.vi"("Message Values"=w185, "Message Names"=string[] ["GetActiveItemTag", "Display Data", "Update Display"], "Message Queue in"=w182) -> ()  [unwired: 7 in, 2 out]
          }
          frame "Tangent On/Off" {
            n91 = call "AMC Send Local Message.vi"("Message Name"="Set Tangent Mode", "Message Queue in"=w187) -> ()  [unwired: 8 in, 2 out]
          }
          frame "FilterControl" {
            n92 = call "AMC Send Local Messages.vi"("Message Names"=string[] ["FilterControl", "Display Data", ""], "Message Queue in"=w189) -> ()  [unwired: 8 in, 2 out]
          }
        }
      }
      event Shortcut Menu Selection (User) {
        n93 = event-data() -> ("CtlRef"=w192:refnum<vi>, "ItemTag"=w193:string)  [unwired: 4 out]
        n94 = case shown="\"ChangeSegment\"" w193 {
          tunnel: w192 -> [_ w196 w200 w204]
          tunnel: w191 -> [_ w194 w198 w202]
          frame "", Default {
          }
          frame "DeleteTreeItem" {
            n95 = call "Tree Menu to String.vi"("Control in"=w196) -> ("delimited string"=w195:string)  [unwired: 10 in]
            n96 = call "AMC Send Local Message.vi"("Message Value"=w195, "Message Name"="DeleteTreeItem", "Message Queue in"=w194) -> ()  [unwired: 7 in, 2 out]
          }
          frame "ChangeSegment" {
            n97 = call "Tree Menu to String.vi"("Control in"=w200) -> ("delimited string"=w199:string)  [unwired: 10 in]
            n98 = call "AMC Send Local Message.vi"("Message Value"=w199, "Message Name"="ChangeSegment", "Message Queue in"=w198) -> ()  [unwired: 7 in, 2 out]
          }
          frame "ExportGraphs" {
            n99 = call "Tree Menu to String.vi"("Control in"=w204) -> ("delimited string"=w203:string)  [unwired: 10 in]
            n100 = call "AMC Send Local Message.vi"("Message Value"=w203, "Message Name"="ExportGraphs", "Message Queue in"=w202) -> ()  [unwired: 7 in, 2 out]
          }
        }
      }
      event Value Change {
        n101 = event-data() -> ("CtlRef"=w209:refnum<vi>)  [unwired: 1 out]
        n102 = property class="Ctl"(reference=w209) -> (reference out=w206:refnum<vi>, "Label.Text"=w208:string)  [unwired: 1 in, 1 out]
        n103 = case shown="\"Data Menu\"" w208 {
          tunnel: w207 -> [_ _ _ w210 w215 w217]
          tunnel: w206 -> [_ _ _ _ w214 _]
          frame "", Default {
          }
          frame "ReportSelection" {
          }
          frame "Data Listbox" {
          }
          frame "GenerateReport" {
            n104 = call "AMC Send Local Message.vi"("Message Name"="GenerateReport", "Message Queue in"=w210) -> ()  [unwired: 8 in, 2 out]
          }
          frame "Data Menu" {
            # "Need to convert to array because\nmultiple messages"
            n105 = call "Tree Menu to String.vi"("Control in"=w214) -> ("delimited string"=w213:string)  [unwired: 10 in]
            n106 = Build Array(w213) -> (w212:string[])
            n107 = call "AMC Send Local Messages.vi"("Message Values"=w212, "Message Names"=string[] ["FillDataTable", "DCM: Create Export Path", "DCM: Load DICOM Info", "DCM: Update Variables"], "Message Queue in"=w215) -> ()  [unwired: 7 in, 2 out]
          }
          frame "Send To PACS" {
            n108 = call "AMC Send Local Messages.vi"("Message Names"=string[] ["DCM: Create Export Path", "DCM: Export Journal"], "Message Queue in"=w217) -> ()  [unwired: 8 in, 2 out]
          }
        }
      }
      event Shortcut Menu Selection (User) {
        n109 = event-data() -> ("CtlRef"=w221:refnum<vi>, "ItemTag"=w222:string, "Coords"=w220:T9)  [unwired: 3 out]
        n110 = case shown="\"DeleteSingleMeasurement\"" w222 {
          tunnel: w221 -> [_ w224 w233]
          tunnel: w220 -> [_ _ w230]
          tunnel: w219 -> [_ w223 w228]
          frame "", Default {
          }
          frame "DeleteTreeItem" {
            n111 = call "Tree Menu to String.vi"("Control in"=w224) -> ("delimited string"=w225:string)  [unwired: 10 in]
            n112 = call "AMC Send Local Message.vi"("Message Value"=w225, "Message Name"="DeleteTreeItem", "Message Queue in"=w223) -> ()  [unwired: 7 in, 2 out]
          }
          frame "DeleteSingleMeasurement" {
            w232 = refnum<vi> refnum  # MulticolumnListbox
            n113 = To More Specific Class(target class=w232, reference=w233) -> (specific class reference=w231:refnum<vi>)  [unwired: 1 in, 1 out]
            n114 = invoke class="MCListbox" method="Point To Row Column"(reference=w231, "Point"=w230) -> ("CellPosition"=w234:T10)  [unwired: 5 in, 6 out]
            n115 = Flatten To String(anything=w234) -> (data string=w227:string)  [unwired: 3 in, 2 out]
            n116 = call "AMC Send Local Message.vi"("Message Value"=w227, "Message Name"="DeleteSingleMeasurement", "Message Queue in"=w228) -> ()  [unwired: 7 in, 2 out]
          }
        }
      }
      event User Event {
        n117 = event-data() -> ("Event"=w235:string)  [unwired: 1 out]
        n118 = case shown="\"BTelement\"" w235 {
          selector: w235 -> [_ _ _ _ _ _ _ _ _ w257 _ _ _]
          tunnel: w236 -> [_ w237 w243 w246 w247 w249 w251 w254 w256 w258 w260 w262 w264]
          frame "", Default {
          }
          frame "DaqError" {
            n119 = One Button Dialog(message="Programmet kan ikke få kontakt til dit USB6008\ndataopsamlingskort. Undersøg venligst om dette er\ntilsluttet korrekt.", button name ("OK")="Luk") -> ()  [unwired: 1 out]
            n120 = call "AMC Send Local Messages.vi"("Message Names"=string[] ["Stop Reference", "Update Display"], "Message Queue in"=w237) -> ()  [unwired: 8 in, 2 out]
          }
          frame "tdmsError" {
            n121 = One Button Dialog(message="Data fejl", button name ("OK")="Luk") -> ()  [unwired: 1 out]
            n122 = call "AMC Send Local Messages.vi"("Message Names"=string[] ["Stop Reference", "Update Display"], "Message Queue in"=w243) -> ()  [unwired: 8 in, 2 out]
          }
          frame "SavePressure" {
            n123 = call "AMC Send Local Messages.vi"("Message Names"=string[] ["GetProcessData", "SaveProcessData"], "Message Queue in"=w246) -> ()  [unwired: 8 in, 2 out]
          }
          frame "TangentMode" {
            n124 = call "AMC Send Local Message.vi"("Message Name"="Set Tangent Mode: True", "Message Queue in"=w247) -> ()  [unwired: 8 in, 2 out]
          }
          frame "StopCalibration" {
            n125 = call "AMC Send Local Messages.vi"("Message Names"=string[] ["Calibrate Pressure: Step 3", "Monitor Reference"], "Message Queue in"=w249) -> ()  [unwired: 8 in, 2 out]
          }
          frame "Set Acquisition Mode" {
            n126 = call "AMC Send Local Messages.vi"("Message Names"=string[] ["Set Acquisition Mode"], "Message Queue in"=w251) -> ()  [unwired: 8 in, 2 out]
          }
          frame "Set DICOM Availability" {
            n127 = call "AMC Send Local Messages.vi"("Message Names"=string[] ["Load Menu", "Initialize: Dicom"], "Message Queue in"=w254) -> ()  [unwired: 8 in, 2 out]
          }
          frame "New Data Path" {
            n128 = call "AMC Send Local Messages.vi"("Message Names"=string[] ["ResetToDefault", "Load Patient Register"], "Message Queue in"=w256) -> ()  [unwired: 8 in, 2 out]
          }
          frame "Regulation Stopped" {
            n129 = call "AMC Send Local Message.vi"("Message Name"=w257, "Message Queue in"=w258) -> ()  [unwired: 8 in, 2 out]
          }
          frame "Set New Hospital Info" {
            n130 = call "AMC Send Local Message.vi"("Message Name"="Load Hospital Info", "Message Queue in"=w260) -> ()  [unwired: 8 in, 2 out]
          }
          frame "Change Language" {
            n131 = call "AMC Send Local Messages.vi"("Message Names"=string[] ["Change Language", "Load Patient Register", "Initialize: Dicom"], "Message Queue in"=w262) -> ()  [unwired: 8 in, 2 out]
          }
          frame "BTelement" {
            n132 = call "AMC Send Local Message.vi"("Message Name"="BT: Dequeue Element", "Message Queue in"=w264) -> ()  [unwired: 8 in, 2 out]
          }
        }
      }
      event User Event {
        n133 = event-data() -> ()  [unwired: 2 out]
        n134 = call "AMC Send Local Messages.vi"("Message Names"=string[] ["BT: Stop", "Exit"], "Message Queue in"=w267) -> ()  [unwired: 8 in, 2 out]
      }
      event Panel Close? {
        w270 = TRUE  # Discard?
        n135 = event-data() -> ()  [unwired: 2 out]
        n136 = call "AMC Send Local Message.vi"("Message Name"="Exit", "Message Queue in"=w268) -> ()  [unwired: 8 in, 2 out]
        n137 = event-data("Discard?"=w270) -> ()  [unwired: 1 in, 1 out]
      }
      event Key Down {
        n138 = event-data() -> ("VKey"=w273:T11, "ScanCode"=w274:i16)  [unwired: 3 out]
        n139 = case shown="57" w274 {
          tunnel: w273 -> [_ _ w279 w284]
          tunnel: w272 -> [_ w276 w278 w283]
          frame 0, Default {
          }
          frame 57 {
            # "Space"
            n140 = call "AMC Send Local Message.vi"("Message Value"="Space", "Message Name"="KeyDown", "Message Queue in"=w276) -> ()  [unwired: 7 in, 2 out]
          }
          frame 77 {
            n141 = case shown="\"Right\"" w279 {
              tunnel: w278 -> [_ w281]
              frame "ASCII", Default {
              }
              frame "Right" {
                # "Rightarrow"
                n142 = call "AMC Send Local Message.vi"("Message Value"="Right", "Message Name"="KeyDown", "Message Queue in"=w281) -> ()  [unwired: 7 in, 2 out]
              }
            }
          }
          frame 75 {
            n143 = case shown="\"Left\"" w284 {
              tunnel: w283 -> [_ w286]
              frame "ASCII", Default {
              }
              frame "Left" {
                # "Leftarrow"
                n144 = call "AMC Send Local Message.vi"("Message Value"="Left", "Message Name"="KeyDown", "Message Queue in"=w286) -> ()  [unwired: 7 in, 2 out]
              }
            }
          }
        }
      }
      event Menu Selection (User) {
        n145 = event-data() -> ("MenuRef"=w288:refnum<k9>, "ItemTag"=w292:string, "ItemPath"=w289:string)  [unwired: 2 out]
        n146 = case shown="\"StartCalibration\"" w292 {
          tunnel: w291 -> [_ w295 _ w297 _ w302 w308 _ _ w311 _ w314 w316 _ _ _ _ _ w326 _ _ _ _]
          tunnel: [_ TRUE _ _ _ _ _ _ _ _ _ _ _ _ _ _ _ _ _ _ _ _ _] -> w290
          tunnel: w289 -> [_ _ _ _ _ _ _ _ _ _ _ _ _ _ _ _ _ _ _ _ _ _ _]
          tunnel: w288 -> [_ _ _ _ _ _ _ _ _ _ _ _ _ _ _ _ _ _ _ _ _ _ _]
          frame Default {
          }
          frame "ExitProgram" {
            n147 = call "AMC Send Local Messages.vi"("Message Names"=string[] ["Close SubVI", "Exit"], "Message Queue in"=w295) -> ()  [unwired: 8 in, 2 out]
          }
          frame "ArmPressureCalculation" {
            n148 = call "ArmPressureCalcMethod.vi"() -> ()  [unwired: 12 in]
          }
          frame "EditDataFolder" {
            n149 = call "SaveDataPath.vi"() -> ("Changed"=w296:bool)  [unwired: 11 in]
            n150 = case shown="True" w296 {
              tunnel: w297 -> [_ w298]
              frame False {
              }
              frame True {
                n151 = call "AMC Send Local Message.vi"("Message Name"="ResetToDefault", "Message Queue in"=w298) -> ()  [unwired: 8 in, 2 out]
              }
            }
          }
          frame "EditJournalFolder" {
            n152 = call "SaveReportPath.vi"() -> ()  [unwired: 12 in]
          }
          frame "StartCalibration" {
            # "Calibration is stopped as userEvent"
            n153 = call "AE Variables.vi"("Action"=Enum_Variables."Get DAQ Connected") -> ("BooleanOut"=w300:bool)  [unwired: 11 in, 7 out]
            n154 = case shown="True" w300 {
              tunnel: w302 -> [_ w305]
              frame False {
                n155 = One Button Dialog(message="Acquisition module must be active") -> ()  [unwired: 1 in, 1 out]
              }
              frame True {
                n156 = call "AMC Send Local Messages.vi"("Message Names"=string[] ["Idle Monitor Reference", "Calibrate Pressure: Step 1", "Calibrate Pressure: Step 2"], "Message Queue in"=w305) -> ()  [unwired: 8 in, 2 out]
                n157 = call "stopCalibrationPopUp.vi"() -> ()  [unwired: 12 in]
              }
            }
          }
          frame "MeasurementTest" {
            n158 = call "AE Variables.vi"("Action"=Enum_Variables."Get DAQ Connected") -> ("BooleanOut"=w306:bool)  [unwired: 11 in, 7 out]
            n159 = case shown="True" w306 {
              tunnel: w308 -> [_ w309]
              frame False {
              }
              frame True {
                n160 = call "AMC Send Local Messages.vi"("Message Names"=string[] ["Stop Monitor Reference", "AcqTest", "Monitor Reference"], "Message Queue in"=w309) -> ()  [unwired: 8 in, 2 out]
              }
            }
          }
          frame "LowpassFilter" {
            n161 = call "acqFilterSelection.vi"() -> ()  [unwired: 12 in]
          }
          frame "Options" {
            n162 = call-by-ref "?"() -> ()  [unwired: 14 in, 2 out]
          }
          frame "FlowCalc" {
            n163 = call "AMC Send Local Message.vi"("Message Name"="Flow: View Signals", "Message Queue in"=w311) -> ()  [unwired: 8 in, 2 out]
          }
          frame "DICOM Server" {
            n164 = call "DICOMServerSettings.vi"() -> ()  [unwired: 12 in]
          }
          frame "EditDicomValues" {
            n165 = call "AMC Send Local Messages.vi"("Message Names"=string[] ["DCM: Edit Values"], "Message Queue in"=w314) -> ()  [unwired: 8 in, 2 out]
          }
          frame "ShowDicomValues" {
            n166 = call "AMC Send Local Messages.vi"("Message Names"=string[] ["DCM: Show Values"], "Message Queue in"=w316) -> ()  [unwired: 8 in, 2 out]
          }
          frame "Journal" {
            w317 = u16 0 items=["Journal", "Graph"]
            n167 = call "AE Variables.vi"("VariantIn"=w317, "Action"=Enum_Variables."Set JournalExport") -> ()  [unwired: 10 in, 8 out]
            n168 = call "AE Save.vi"("Variant In"=w317, "Action"=Enum_Save_Action_Events."SaveJournalType") -> ()  [unwired: 7 in, 2 out]
          }
          frame "Graph" {
            w320 = u16 1 items=["Journal", "Graph"]
            n169 = call "AE Variables.vi"("VariantIn"=w320, "Action"=Enum_Variables."Set JournalExport") -> ()  [unwired: 10 in, 8 out]
            n170 = call "AE Save.vi"("Variant In"=w320, "Action"=Enum_Save_Action_Events."SaveJournalType") -> ()  [unwired: 7 in, 2 out]
          }
          frame "Bitmap" {
            w323 = u16 0 items=["Bitmap", "JPEG"] ("Encoding")
            n171 = call "DICOMFileEncoding.vi"("Encoding"=w323) -> ()  [unwired: 11 in]
          }
          frame "JPEG" {
            w324 = u16 1 items=["Bitmap", "JPEG"] ("Encoding")
            n172 = call "DICOMFileEncoding.vi"("Encoding"=w324) -> ()  [unwired: 11 in]
          }
          frame "ChangePassword" {
            n173 = call "change_password.vi"() -> ()  [unwired: 12 in]
          }
          frame "UpdateProgram" {
            n174 = call "AMC Send Local Message.vi"("Message Name"="Update Program", "Message Queue in"=w326) -> ()  [unwired: 8 in, 2 out]
          }
          frame "ActivateDICOM" {
            n175 = call "Activation.vi"() -> ()  [unwired: 12 in]
          }
          frame "Danish" {
            (unwired) u16 0 ("Value (Signaling)")
          }
          frame "English" {
            (unwired) u16 1 ("Value (Signaling)")
          }
          frame "French" {
            (unwired) u16 2 ("Value (Signaling)")
          }
        }
      }
      event Menu Activation? {
        n176 = event-data() -> ("MenuRef"=w327:refnum<k9>)  [unwired: 1 out]
        n177 = call "AE Variables.vi"("Action"=Enum_Variables."Get DICOM Avail") -> ("BooleanOut"=w328:bool)  [unwired: 11 in, 7 out]
        n178 = case shown="True" w328 {
          tunnel: w327 -> [_ w330]
          frame False {
          }
          frame True {
            n179 = Get Menu Item Info(7:"FileEncoding" ("item tag"), 11:w330) -> (3:w338:refnum<k9>, 5:w339:string[])  [unwired: 1 in, 5 out]
            n180 = call "AE Variables.vi"("Action"=Enum_Variables."Get DICOM Encode") -> ("RingOut"=w337:u16)  [unwired: 11 in, 7 out]
            n181 = for {
              tunnel: w339 -> [w351] mode=indexing
              tunnel: w338 -> [w352]
              tunnel: w337 -> [w350]
              tunnel: [w347] -> w336
              i -> [w349]
              n182 = Equal?(x=w350, y=w349) -> (x = y?=w348:bool)
              n183 = Set Menu Item Info(6:w348, 7:w351, 11:w352) -> (3:w347:refnum<k9>)  [unwired: 4 in, 1 out]
            }
            n184 = Get Menu Item Info(7:"ExportType" ("item tag"), 11:w336) -> (3:w333:refnum<k9>, 5:w334:string[])  [unwired: 1 in, 5 out]
            n185 = call "AE Variables.vi"("Action"=Enum_Variables."Get JournalExport") -> ("RingOut"=w332:u16)  [unwired: 11 in, 7 out]
            n186 = for {
              tunnel: w334 -> [w345] mode=indexing
              tunnel: w333 -> [w346]
              tunnel: w332 -> [w344]
              i -> [w343]
              n187 = Equal?(x=w344, y=w343) -> (x = y?=w342:bool)
              n188 = Set Menu Item Info(6:w342, 7:w345, 11:w346) -> ()  [unwired: 4 in, 2 out]
            }
          }
        }
        n189 = event-data() -> ()  [unwired: 2 in, 1 out]
      }
    }
  }
  n190 = while "Primary Execution Loop" {
    shift-right: [w370] -> w17
    shift-left: w12 -> [w358]
    shift-right: [w367] -> _
    shift-left: _ -> [w361]
    shift-right: [w366] -> w16
    shift-left: w6 -> [w369]
    tunnel: w6 -> [w368]
    tunnel: w7 -> [w364]
    tunnel: w5 -> [w365]
    tunnel: [w354] -> w1 mode=indexing
    stop <- w362 stop-if-true
    # "<Dyn Events>"
    # "<Default Val>"
    n191 = call "AMC Read Next Message.vi"("error in (no error)"=w358, "timeout (1ms)"=w361, "Message Queue in"=w364) -> ("error out"=w360:errorcluster, "Message Value"=w359:string, "Message Name"=w356:string, "Message Queue out"=w363:T6, "Exit Process"=w362:bool)  [unwired: 2 in, 2 out]
    n192 = case shown="\"Initialize: Configuration\"" w356 {
      selector: w356 -> [_ _ _ _ _ _ _ _ _ _ _ _ _ _ _ _ _ _ w600 _ _ _ _ _ _ _ _ _ _ _ _ _ _ _ _ _ _ _ _ _ _ _ _ _ _ _ _ _ _ _ _ _ _ _ _ _ _ _ _ _ _ _ _ _ _ _ _ _ _ _ _ _ _ _ _ _ _ _ _ _ _ _ _ _ _ _ _ _ _ _ _ _ _ _ _ _ _ _ _ _ _ _ _ _ _ _ _ _ _ _ _ _ _ _ _ w2466]
      tunnel: [w373 w386 w387 w395 w410 w423 w440 w453 w468 w484 w495 w506 w512 w529 w553 w562 w571 w596 w612 w616 w620 w639 w659 w665 w676 w678 w679 w686 w692 w698 w704 w710 w713 w719 w721 w722 w743 w753 w764 w769 w799 w836 w866 w875 w1138 w1170 w1187 w1208 w1228 w1236 w1245 w1270 w1288 w1305 w1347 w1358 w1375 w1388 w1391 w1409 w1430 w1458 w1460 w1473 w1475 w1476 w1491 w1526 w1551 w1559 w1568 w1579 w1593 w1603 w1617 w1625 w1634 w1645 w1665 w1705 w1733 w1747 w1755 w1776 w1821 w1831 w1833 w1837 w1843 w1846 w1876 w1883 w1892 w1901 w1905 w2050 w2081 w2102 w2112 w2131 w2149 w2196 w2216 w2250 w2273 w2294 w2317 w2347 w2362 w2379 w2396 w2435 w2442 w2459 w2464 w2470] -> w370
      tunnel: w360 -> [w375 w386 w388 w392 w412 w424 w439 w454 w469 w483 w496 w506 w513 w537 w548 w564 w568 w597 w602 w616 w619 w651 w659 w663 w676 w678 w680 w687 w693 w699 w705 w711 w714 w719 w721 w724 w750 w756 w764 w769 w803 w837 w866 w876 w1139 w1171 w1188 w1208 w1229 w1237 w1247 w1269 w1289 w1304 w1348 w1360 w1363 w1376 w1392 w1410 w1429 w1458 w1461 w1473 w1475 w1484 w1492 w1527 w1552 w1560 w1569 w1581 w1595 w1605 w1618 w1626 w1633 w1645 w1663 w1706 w1732 w1747 w1754 w1777 w1822 w1831 w1833 w1837 w1839 w1848 w1876 w1885 w1894 w1903 w1923 w2053 w2078 w2102 w2104 w2136 w2152 w2196 w2217 w2251 w2272 w2296 w2318 w2347 w2354 w2379 w2398 w2435 w2443 w2457 w2464 w2471]
      tunnel: w363 -> [w371 _ _ _ _ _ _ _ _ w492 w500 w504 _ _ _ _ _ _ _ _ _ _ _ _ _ _ _ _ _ _ _ _ _ _ _ w725 _ _ _ w768 w796 _ _ _ _ _ _ _ _ _ _ _ _ _ _ _ _ _ _ _ _ _ _ _ _ _ w1494 w1529 _ _ _ _ _ _ _ _ w1631 _ _ _ _ _ _ _ w1823 _ _ _ _ _ _ _ _ _ _ _ _ _ _ _ _ _ _ _ _ _ _ w2345 _ _ _ _ w2441 _ _ _]
      tunnel: w369 -> [w372 w385 w390 w405 w418 w426 w448 w463 w478 w494 w502 w505 w521 w533 w552 w567 w570 w599 w608 w615 w618 w657 w658 w674 w675 w677 w682 w685 w690 w696 w702 w708 w717 w718 w720 w728 w752 w762 w763 w766 w797 w838 w863 w889 w1137 w1166 w1189 w1207 w1219 w1239 w1241 w1268 w1292 w1294 w1336 w1353 w1367 w1380 w1390 w1408 w1428 w1457 w1467 w1470 w1474 w1482 w1498 w1532 w1558 w1563 w1567 w1582 w1596 w1606 w1621 w1628 w1632 w1644 w1666 w1704 w1739 w1745 w1762 w1779 w1825 w1830 w1832 w1836 w1842 w1851 w1875 w1882 w1891 w1900 w1922 w2047 w2075 w2101 w2111 w2134 w2164 w2195 w2224 w2254 w2279 w2311 w2333 w2346 w2361 w2378 w2401 w2434 w2438 w2462 w2463 w2472]
      tunnel: w368 -> [_ _ _ _ _ _ _ _ _ _ _ _ _ _ _ _ _ _ _ _ _ _ _ _ _ _ _ _ _ _ _ _ _ _ _ _ _ _ _ _ _ _ _ _ _ _ _ _ _ _ _ _ _ _ _ _ _ _ _ _ _ _ _ _ _ _ _ _ _ _ _ _ _ _ _ _ _ _ _ _ _ _ _ _ _ _ _ _ _ _ _ _ _ _ _ _ _ _ _ _ _ _ _ _ _ _ _ _ _ _ _ _ _ _ _ _]
      tunnel: [w372 w385 w390 w404 w417 w425 w447 w462 w477 w494 w502 w505 w521 w545 w552 w567 w572 w599 w607 w615 w621 w657 w658 w674 w675 w677 w682 w684 w689 w695 w701 w707 w717 w718 w720 w728 w752 w762 w763 w766 w804 w838 w863 w888 w1137 w1172 w1189 w1206 w1219 w1239 w1241 w1268 w1292 w1303 w1335 w1353 w1367 w1380 w1390 w1408 w1428 w1457 w1467 w1469 w1474 w1481 w1498 w1532 w1558 w1563 w1567 w1582 w1596 w1606 w1620 w1630 w1636 w1644 w1666 w1703 w1738 w1752 w1762 w1798 w1825 w1830 w1832 w1835 w1842 w1855 w1875 w1882 w1891 w1900 w1922 w2047 w2075 w2101 w2113 w2133 w2164 w2195 w2224 w2254 w2279 w2311 w2333 w2346 w2360 w2378 w2401 w2434 w2437 w2462 w2463 w2472] -> w366
      tunnel: [200 _ _ _ _ _ _ _ _ _ _ _ _ _ _ _ _ _ _ _ _ _ _ _ _ _ _ _ _ _ _ _ _ _ _ _ _ _ _ _ _ _ _ _ _ _ _ _ _ _ _ _ _ _ _ _ _ _ _ _ _ _ _ _ _ _ _ _ _ _ _ _ _ _ _ _ _ _ _ _ _ _ _ _ _ _ _ _ _ _ _ _ _ _ _ _ _ _ _ _ _ _ _ _ _ _ _ _ _ _ _ _ _ _ _ _] -> w367
      tunnel: w365 -> [_ _ _ _ _ _ _ _ _ _ _ _ _ _ _ _ _ _ w606 _ _ _ _ _ _ _ _ _ _ _ _ _ _ _ _ _ _ _ _ _ _ _ _ _ _ _ _ _ _ _ _ _ _ _ _ _ _ _ _ _ _ _ _ _ _ _ _ _ _ _ _ _ _ _ _ _ _ _ _ _ _ _ _ _ _ _ _ _ _ _ _ _ _ _ _ _ _ _ _ _ _ _ _ _ _ _ _ _ _ _ _ _ _ _ _ _]
      tunnel: w359 -> [_ _ _ _ _ _ _ _ _ _ _ _ _ _ _ _ _ _ _ _ _ _ _ _ _ _ _ _ _ _ _ _ _ _ _ _ _ _ _ w767 _ _ _ _ _ _ _ _ _ _ _ _ _ w1299 _ _ w1365 w1378 _ _ _ _ w1463 _ _ _ _ _ _ _ _ _ _ _ _ _ _ _ _ _ _ _ _ _ _ _ _ w1834 _ _ _ _ _ _ w1917 w2048 w2080 _ w2108 _ w2167 _ _ _ _ _ _ _ _ _ _ _ _ _ _ _]
      frame "", "Idle" {
        n193 = Unbundle By Name(w372) -> ("Reference signal.Monitor"=w374:bool)
        n194 = case shown="True" w374 {
          tunnel: w375 -> [w377 w384]
          tunnel: [w377 w381] -> w373
          tunnel: w371 -> [_ w379]
          frame False {
          }
          frame True {
            n195 = call "AE Events.vi"("error in (no error)"=w384, "Action"=enum16{"Init", "Get Event", "Set Event"}."Get Event") -> ("error out"=w382:errorcluster, "Event Out"=w378:dbl)  [unwired: 8 in]
            n196 = call "AE Paper.vi"("error in (no error)"=w382, "Message Queue in"=w379, "Events"=w378, "Action Events"=Enum_Paper_Action_Events."Paper State") -> ("error out"=w381:errorcluster)  [unwired: 5 in, 1 out]
          }
        }
      }
      frame "/*********Initialize********/" {
      }
      frame "preInitialize" {
        n197 = control-ref of="This VI"() -> (w389:refnum<vi>)
        n198 = call <vilib>:"Set Busy.vi"("error in (no error)"=w388, "VI reference (current VI)"=w389) -> ("error out"=w387:errorcluster)  [unwired: 8 in, 1 out]
      }
      frame "Initialize: PageMenu" {
        n199 = vi-ref "main.lvlib:Top Menu.vi"() -> (w398:refnum<vi>)
        n200 = call "Notifier AE.vi"("error in (no error)"=w392, "String"="Initialising Pages") -> ("error out"=w391:errorcluster)  [unwired: 9 in]
        n201 = property class="VI"(reference=w398) -> ("Name"=w397:string)  [unwired: 1 in, 2 out]
        n202 = Obtain Queue(name (unnamed)="Menu Queue", element data type=cluster{"Msg":string, "Data":variant} {"Msg"="", "Data"=variant}, error in (no error)=w391) -> (queue out=w396:refnum<queue>, error out=w399:errorcluster)  [unwired: 2 in, 1 out]
        n203 = Open VI Reference(type specifier VI Refnum (for type only)=refnum<vi> refnum, vi path=w397, options=128, error in (no error)=w399) -> (vi reference=w403:refnum<vi>, error out=w402:errorcluster)  [unwired: 2 in]
        n204 = call-by-ref "Start Asynchronous Call"(reference=w403, error in=w402, "Menu Queue"=w396) -> (reference out=w394:refnum<vi>, error out=w395:errorcluster)  [unwired: 11 in]
        n205 = Bundle By Name(cluster=w405, "PageMenu.VI Reference"=w394, "PageMenu.Queue"=w396) -> (w404:T3)
      }
      frame "Initialize: Profile" {
        n206 = vi-ref "main.lvlib:Profile.vi"() -> (w409:refnum<vi>)
        n207 = property class="VI"(reference=w409) -> ("Name"=w408:string)  [unwired: 1 in, 2 out]
        n208 = Obtain Queue(name (unnamed)="Profile Queue", element data type=cluster{"Msg":string, "Data":variant} {"Msg"="", "Data"=variant}, error in (no error)=w412) -> (queue out=w413:refnum<queue>, error out=w411:errorcluster)  [unwired: 2 in, 1 out]
        n209 = Open VI Reference(type specifier VI Refnum (for type only)=refnum<vi> refnum, vi path=w408, options=128, error in (no error)=w411) -> (vi reference=w416:refnum<vi>, error out=w414:errorcluster)  [unwired: 2 in]
        n210 = call-by-ref "Start Asynchronous Call"(reference=w416, error in=w414, "Queue In"=w413) -> (reference out=w415:refnum<vi>, error out=w410:errorcluster)  [unwired: 11 in]
        n211 = Bundle By Name(cluster=w418, "Profile.VI Reference"=w415, "Profile.Queue"=w413) -> (w417:T3)
      }
      frame "Initialize: Configuration" {
        n212 = vi-ref "main.lvlib:Configuration.vi"() -> (w430:refnum<vi>)
        n213 = Obtain Queue(name (unnamed)="Configuration Queue", element data type=cluster{"Msg":string, "Data":variant} {"Msg"="", "Data"=variant}, error in (no error)=w424) -> (queue out=w427:refnum<queue>, error out=w428:errorcluster)  [unwired: 2 in, 1 out]
        n214 = property class="VI"(reference=w430) -> ("Name"=w429:string)  [unwired: 1 in, 2 out]
        n215 = Open VI Reference(type specifier VI Refnum (for type only)=refnum<vi> refnum, vi path=w429, options=128, error in (no error)=w428) -> (vi reference=w433:refnum<vi>, error out=w431:errorcluster)  [unwired: 2 in]
        n216 = call-by-ref "Start Asynchronous Call"(reference=w433, error in=w431, "Queue In"=w427) -> (reference out=w432:refnum<vi>, error out=w423:errorcluster)  [unwired: 11 in]
        n217 = Bundle By Name(cluster=w426, "Configuration.VI Reference"=w432, "Configuration.Queue"=w427) -> (w425:T3)
      }
      frame "Initialize: Acquisition" {
        n218 = vi-ref "main.lvlib:Acquisition.vi"() -> (w443:refnum<vi>)
        n219 = Obtain Queue(name (unnamed)="Acquisition Queue", element data type=cluster{"Msg":string, "Data":variant} {"Msg"="", "Data"=variant}, error in (no error)=w439) -> (queue out=w438:refnum<queue>, error out=w441:errorcluster)  [unwired: 2 in, 1 out]
        n220 = property class="VI"(reference=w443) -> ("Name"=w442:string)  [unwired: 1 in, 2 out]
        n221 = Open VI Reference(type specifier VI Refnum (for type only)=refnum<vi> refnum, vi path=w442, options=128, error in (no error)=w441) -> (vi reference=w446:refnum<vi>, error out=w444:errorcluster)  [unwired: 2 in]
        n222 = call-by-ref "Start Asynchronous Call"(reference=w446, error in=w444, "Queue In"=w438) -> (reference out=w445:refnum<vi>, error out=w440:errorcluster)  [unwired: 11 in]
        n223 = Bundle By Name(cluster=w448, "Acquisition.VI Reference"=w445, "Acquisition.Queue"=w438) -> (w447:T3)
      }
      frame "Initialize: Data" {
        n224 = Obtain Queue(name (unnamed)="Data Queue", element data type=cluster{"Msg":string, "Data":variant} {"Msg"="", "Data"=variant}, error in (no error)=w454) -> (queue out=w456:refnum<queue>, error out=w455:errorcluster)  [unwired: 2 in, 1 out]
        n225 = vi-ref "main.lvlib:Data.vi"() -> (w458:refnum<vi>)
        n226 = property class="VI"(reference=w458) -> ("Name"=w457:string)  [unwired: 1 in, 2 out]
        n227 = Open VI Reference(type specifier VI Refnum (for type only)=refnum<vi> refnum, vi path=w457, options=128, error in (no error)=w455) -> (vi reference=w461:refnum<vi>, error out=w459:errorcluster)  [unwired: 2 in]
        n228 = call-by-ref "Start Asynchronous Call"(reference=w461, error in=w459, "Queue In"=w456) -> (reference out=w460:refnum<vi>, error out=w453:errorcluster)  [unwired: 11 in]
        n229 = Bundle By Name(cluster=w463, "Data.VI Reference"=w460, "Data.Queue"=w456) -> (w462:T3)
      }
      frame "Initialize: Journal" {
        n230 = vi-ref "main.lvlib:Journal.vi"() -> (w473:refnum<vi>)
        n231 = Obtain Queue(name (unnamed)="Journal Queue", element data type=cluster{"Msg":string, "Data":variant} {"Msg"="", "Data"=variant}, error in (no error)=w469) -> (queue out=w471:refnum<queue>, error out=w470:errorcluster)  [unwired: 2 in, 1 out]
        n232 = property class="VI"(reference=w473) -> ("Name"=w472:string)  [unwired: 1 in, 2 out]
        n233 = Open VI Reference(type specifier VI Refnum (for type only)=refnum<vi> refnum, vi path=w472, options=128, error in (no error)=w470) -> (vi reference=w476:refnum<vi>, error out=w474:errorcluster)  [unwired: 2 in]
        n234 = call-by-ref "Start Asynchronous Call"(reference=w476, error in=w474, "Queue In"=w471) -> (reference out=w475:refnum<vi>, error out=w468:errorcluster)  [unwired: 11 in]
        n235 = Bundle By Name(cluster=w478, "Journal.VI Reference"=w475, "Journal.Queue"=w471) -> (w477:T3)
      }
      frame "Send Caller Queue to Journal" {
        w489 = cluster{"Msg":string, "Data":variant} {"Msg"="", "Data"=variant} ("element")
        # "To make sure all references are passed to References.vi the rest of the initialization is activated from Journal.vi"
        n236 = Unbundle By Name(w494) -> ("Journal.Queue"=w493:refnum<queue>)
        n237 = Bundle By Name(cluster=w489, "Msg"="Set Caller Queue", "Data"=w492) -> (w491:cluster{"Msg":string, "Data":variant})
        n238 = Enqueue Element(queue=w493, element=w491, error in (no error)=w483) -> (queue out=w487:refnum<queue>, error out=w485:errorcluster)  [unwired: 1 in, 1 out]
        n239 = Bundle By Name(cluster=w489, "Msg"="Register Refs") -> (w486:cluster{"Msg":string, "Data":variant})
        n240 = Enqueue Element(queue=w487, element=w486, error in (no error)=w485) -> (error out=w484:errorcluster)  [unwired: 1 in, 2 out]
      }
      frame "Send Caller Queue to Acquisition" {
        # "To control the acquisition"
        n241 = Unbundle By Name(w502) -> ("Acquisition.Queue"=w501:refnum<queue>)
        n242 = Bundle By Name(cluster=cluster{"Msg":string, "Data":variant} {"Msg"="", "Data"=variant} ("element"), "Msg"="Set Caller Queue", "Data"=w500) -> (w499:cluster{"Msg":string, "Data":variant})
        n243 = Enqueue Element(queue=w501, element=w499, error in (no error)=w496) -> (error out=w495:errorcluster)  [unwired: 1 in, 2 out]
      }
      frame "Continue Initializing" {
        w503 = string[] ["Send Caller Queue to Acquisition", "Register User Parameters", "Initialize", "Change Language", "", "Load Patient Register", "Cache User Parameters", "Load Hospital Info", "Subpanel: Load Menu", "Subpanel: Load Profile", "Reset Graphs", "Set SubVi Color", "Silent DAQ Initialization", "Update Display", "Set Acquisition Mode", "", "Set Height", "ResetToDefault", "End Initializing"]  # Initial Elements
        n244 = call "AMC Send Local Messages.vi"("Message Names"=w503, "Message Queue in"=w504) -> ()  [unwired: 8 in, 2 out]
      }
      frame "Set SubVi Color" {
        w507 = u32 16777226
        n245 = Unbundle By Name(w521) -> ("PageMenu.Queue"=w520:refnum<queue>, "Profile.Queue"=w519:refnum<queue>, "Configuration.Queue"=w518:refnum<queue>, "Acquisition.Queue"=w517:refnum<queue>, "Data.Queue"=w516:refnum<queue>, "Journal.Queue"=w515:refnum<queue>)
        n246 = Bundle By Name(cluster=cluster{"Msg":string, "Data":variant} {"Msg"="", "Data"=variant} ("element"), "Msg"="Set Color", "Data"=w507) -> (w509:cluster{"Msg":string, "Data":variant})
        n247 = control-ref of="This VI"() -> (w508:refnum<vi>)
        n248 = call "Set VI Color.vi"("Pane Color"=w507, "VI in"=w508) -> ()  [unwired: 10 in]
        n249 = Build Array(w520, w519, w518, w517, w516, w515) -> (w514:refnum<queue>[])
        n250 = for {
          tunnel: w514 -> [w525] mode=indexing
          shift-right: [w524] -> w512
          shift-left: w513 -> [w523]
          tunnel: w509 -> [w522]
          n251 = Enqueue Element(queue=w525, element=w522, error in (no error)=w523) -> (error out=w524:errorcluster)  [unwired: 1 in, 2 out]
        }
      }
      frame "Initialize" {
        n252 = Unbundle By Name(w533) -> ("cRef.Profile.References.ListboxDoctor"=w532:refnum<vi>, "cRef.Profile.References.ListboxOperator"=w531:refnum<vi>)
        n253 = call "UpdateGlobals.vi"("error in (no error)"=w537, "Operator Listbox Ref"=w531, "Doctor Listbox Ref"=w532) -> ("error out"=w530:errorcluster)  [unwired: 7 in]
        n254 = call "AE DataProcessControl.vi"("Action"=Enum_Process_Data."Init", "error in (no error)"=w530) -> ("error out"=w538:errorcluster)  [unwired: 7 in, 2 out]
        n255 = call "AE Variables.vi"("VariantIn"=TRUE, "error in (no error)"=w538, "Action"=Enum_Variables."Set Encryption") -> ("error out"=w536:errorcluster)  [unwired: 9 in, 7 out]
        n256 = call "AE Variables.vi"("error in (no error)"=w536, "Action"=Enum_Variables."Set ExcelVersion") -> ("error out"=w534:errorcluster)  [unwired: 10 in, 7 out]
        n257 = call "PassNill.vi"("Error In"=w534) -> ("Error Out"=w526:errorcluster)  [unwired: 10 in]
        n258 = Get Date/Time In Seconds() -> (seconds since 1Jan1904=w543:timestamp)
        n259 = Format Date/Time String(time format string (%c)="%Y-%m-%d", seconds (now)=w543) -> (date/time string=w544:string)  [unwired: 1 in]
        n260 = call-poly <userlib>:"MGI Suppress Error Code.vi"("Error Code"=666, "Error In"=w526) -> ("Error Supressed?"=w527:bool, "Error Out"=w529:errorcluster)  [unwired: 4 in]
        n261 = Bundle By Name(cluster=w533, "System Parameters.Date"=w544) -> (w545:T3)
        n262 = disable-structure shown="Default" {
          disable-tunnel: w527 -> [w546 _]
          frame condition #0 {
            n263 = Quit LabVIEW(quit? (T)=w546) -> ()
          }
          frame condition #1 (active) {
          }
        }
      }
      frame "Initialize: Dicom" {
        n264 = Unbundle By Name(w552) -> ("cRef.Profile.References.Query Worklist"=w551:refnum<vi>, "cRef.Journal.References.Send To PACS"=w550:refnum<vi>)
        n265 = call "CheckLicens.vi"("error in (no error)"=w548) -> ("error out"=w549:errorcluster, "Dicom Active"=w547:bool)  [unwired: 9 in]
        n266 = case shown="False" w547 {
          frame False {
            n267 = Current VI's Menubar() -> (w561:refnum<k9>)
            n268 = Delete Menu Items(7:"DICOM" ("item name"), 9:w561) -> ()  [unwired: 2 in, 2 out]
          }
          frame True {
          }
        }
        n269 = property class="Bool"(reference=w550, "Visible"=w547) -> ()  [unwired: 1 in, 2 out]
        n270 = property class="Bool"(reference=w551, "Visible"=w547) -> ()  [unwired: 1 in, 2 out]
        n271 = case shown="True" w547 {
          tunnel: w549 -> [w554 w557]
          tunnel: [w554 w558] -> w553
          frame False {
          }
          frame True {
            n272 = call "AE Save.vi"("error in (no error)"=w557, "Action"=Enum_Save_Action_Events."Load Dicom Tags") -> ("error out"=w556:errorcluster)  [unwired: 7 in, 1 out]
            n273 = call "AE DICOM.vi"("Action"=Enum_DICOM."Set Dicom Encoding", "Error In"=w556) -> ("Error Out"=w558:errorcluster)  [unwired: 9 in]
          }
        }
      }
      frame "postInitialize" {
        n274 = control-ref of="This VI"() -> (w566:refnum<vi>)
        n275 = call <vilib>:"Unset Busy.vi"("error in (no error)"=w564, "VI reference (current VI)"=w566) -> ("error out"=w563:errorcluster)  [unwired: 9 in]
        n276 = property class="VI"(reference=w566, error in=w563, "FP:Transparency"=u8 0 ("Front Panel Window:Transparency")) -> (error out=w562:errorcluster)  [unwired: 1 out]
      }
      frame "Initialize Reference" {
        n277 = Unbundle By Name(w570) -> ("Data Acquisition.Control?"=w569:bool)
        n278 = case shown="False" w569 {
          tunnel: [w593 w594] -> w572
          tunnel: [w575 w595] -> w571
          tunnel: w568 -> [w574 w595]
          tunnel: w570 -> [w573 w594]
          frame False {
            # "Initialize reference  signal acquisition"
            n279 = vi-ref "main.lvlib:RefData(SubVI).vi"() -> (w584:refnum<vi>)
            n280 = property class="VI"(reference=w584) -> ("Name"=w583:string)  [unwired: 1 in, 2 out]
            n281 = Open VI Reference(type specifier VI Refnum (for type only)=refnum<vi> refnum, vi path=w583, options=128, error in (no error)=w574) -> (vi reference=w580:refnum<vi>, error out=w581:errorcluster)  [unwired: 2 in]
            n282 = call-by-ref "Start Asynchronous Call"(reference=w580, error in=w581) -> (reference out=w577:refnum<vi>, error out=w578:errorcluster)  [unwired: 1 in, 1 out]
            n283 = Obtain Queue(name (unnamed)="RefControl", element data type="", error in (no error)=w578) -> (queue out=w587:refnum<queue>, error out=w586:errorcluster)  [unwired: 2 in, 1 out]
            n284 = Flush Queue(queue=w587, error in (no error)=w586) -> (queue out=w585:refnum<queue>, error out=w576:errorcluster)  [unwired: 1 out]
            n285 = Close Reference(reference=w577, error in (no error)=w576) -> (error out=w575:errorcluster)
            n286 = Bundle By Name(cluster=w573, "Reference signal.Queue"=w585, "Reference signal.Monitor"=TRUE, "System Parameters.Paper Running?"=FALSE ("Paper Running?"), "Reference signal.Events"=0.0) -> (w593:T3)
          }
          frame True {
          }
        }
      }
      frame "End Initializing" {
        n287 = call "Notifier AE.vi"("error in (no error)"=w597, "String"="Ready") -> ("error out"=w596:errorcluster)  [unwired: 9 in]
      }
      frame "Register User Parameters" {
        w613 = ""  # Event
        n288 = call "Notifier AE.vi"("error in (no error)"=w602, "String"=w600) -> ("error out"=w601:errorcluster)  [unwired: 9 in]
        n289 = Create User Event(user event datatype=w613, error in=w601) -> (user event=w605:refnum<user-event>, error out=w611:errorcluster)
        n290 = call "Register User Parameters.vi"("User Events"=w605, "error in (no error)"=w602, "SHIFTER DATA"=w608, "Event Registration Refnum in"=w606) -> ("error out"=w604:errorcluster)  [unwired: 7 in]
        n291 = call "References.vi"("error in"=w604, "Reference AE Control"=Reference_AE_Control."Get") -> ("error out"=w603:errorcluster, "Cluster out"=w609:T5)  [unwired: 8 in]
        n292 = call "AE User Events.vi"("Action"=Enum_User_Events."Init", "user event in"=w605) -> ()  [unwired: 8 in, 2 out]
        n293 = Bundle By Name(cluster=w608, "cRef"=w609) -> (w607:T3)
        n294 = Merge Errors(w603, w611) -> (w612:errorcluster)
      }
      frame "/*********Display Updates********/" {
      }
      frame "Cache User Parameters" {
        n295 = Unbundle By Name(w618) -> ("cRef.Configuration.Method"=w617:string)
        n296 = disable-structure shown="Enabled" {
          disable-tunnel: [w626 w636] -> w621
          disable-tunnel: [w625 w635] -> w620
          disable-tunnel: w619 -> [w624 w637]
          disable-tunnel: w618 -> [w623 w638]
          disable-tunnel: w617 -> [w622 _]
          frame Enabled {
            n297 = case shown="\"new\", Default" w622 {
              tunnel: [w628 w634] -> w626
              tunnel: [w627 w633] -> w625
              tunnel: w624 -> [w629 w632]
              tunnel: w623 -> [w630 w631]
              frame "new", Default {
                n298 = call "Cache User Parameters_new method.vi"("error in (no error)"=w629, "SHIFTER DATA in"=w630) -> ("error out"=w627:errorcluster, "SHIFTER DATA out"=w628:T3)  [unwired: 8 in]
              }
              frame "old" {
                n299 = call "Cache User Parameters.vi"("error in (no error)"=w632, "SHIFTER DATA in"=w631) -> ("error out"=w633:errorcluster, "SHIFTER DATA out"=w634:T3)  [unwired: 8 in]
              }
            }
          }
          frame Disabled {
            n300 = call "Cache User Parameters_minimal_test.vi"("error in (no error)"=w637, "SHIFTER DATA in"=w638) -> ("error out"=w635:errorcluster, "SHIFTER DATA out"=w636:T3)  [unwired: 8 in]
          }
        }
      }
      frame "Update Display" {
        n301 = Unbundle By Name(w657) -> ("cRef.Menu.References.PersonalInfoString"=w643:refnum<vi>, "User Parameters.Name"=w641:string, "User Parameters.CPR Number"=w642:string, "cRef.Data.References.AdjustedHeight"=w648:refnum<vi>, "Database.Height Adjustment"=w647:dbl, "cRef.Acquisition.References.SegmentAcqString"=w656:refnum<vi>, "User Parameters.Measuring Limb"=w655:string, "cRef.Menu.References.MenuStartADC"=w653:refnum<vi>)
        n302 = call "AE Variables.vi"("error in (no error)"=w651, "Action"=Enum_Variables."Get DAQ Connected") -> ("BooleanOut"=w650:bool, "error out"=w649:errorcluster)  [unwired: 10 in, 6 out]
        n303 = property class="Bool (strict)"(reference=w653, error in=w649, "Value"=w650) -> (error out=w654:errorcluster)  [unwired: 1 out]
        n304 = property class="Str"(reference=w656, error in=w654, "Value"=w655) -> (error out=w646:errorcluster)  [unwired: 1 out]
        n305 = property class="DigNum (strict)"(reference=w648, error in=w646, "Val(Sgnl)"=w647) -> (error out=w640:errorcluster)  [unwired: 1 out]
        n306 = Concatenate Strings(w641, "\r", w642) -> (w644:string)
        n307 = property class="Str"(reference=w643, error in=w640, "Value"=w644) -> (error out=w639:errorcluster)  [unwired: 1 out]
      }
      frame "/ ***Language***/" {
      }
      frame "Change Language" {
        n308 = call "AE Variables.vi"("Action"=Enum_Variables."Get Language") -> ("RingOut"=w660:u16)  [unwired: 11 in, 7 out]
        n309 = call "getAllRefs.vi"("error in (no error)"=w663, "Language"=w660, "Change Language"=TRUE) -> ("error out"=w662:errorcluster)  [unwired: 7 in, 1 out]
        n310 = Current VI's Path() -> (path=w670:path)
        n311 = Strip Path(path=w670) -> (stripped path=w669:path)  [unwired: 1 out]
        n312 = Index Array(array=string[] ["DM2000RuntimeMenu.rtm", "DM2000RuntimeMenuEng.rtm", "DM2000RuntimeMenuFrench.rtm"], index=w660) -> (element=w671:string)
        n313 = control-ref of="This VI"() -> (w673:refnum<vi>)
        n314 = Build Path(base path=w669, name or relative path=w671) -> (appended path=w668:path)
        n315 = property class="VI"(reference=w673, error in=w662, "RT Menu Path"=w668) -> (reference out=w666:refnum<vi>, error out=w667:errorcluster)
        n316 = Close Reference(reference=w666, error in (no error)=w667) -> (error out=w665:errorcluster)
      }
      frame "/*********Primary Execution********/" {
      }
      frame "/***Subpanel Control***/" {
      }
      frame "Subpanel: Load Menu" {
        n317 = Unbundle By Name(w682) -> ("PageMenu.VI Reference"=w681:refnum<vi>)
        n318 = invoke on="Top Subpanel" class="SubPanel" method="Insert VI"(error in=w680, "VI Ref"=w681) -> (error out=w679:errorcluster)  [unwired: 2 in, 3 out]
      }
      frame "Subpanel: Load Profile" {
        n319 = Unbundle By Name(w685) -> ("Profile.VI Reference"=w688:refnum<vi>)
        n320 = invoke on="Main Subpanel" class="SubPnl" method="Insert VI"(error in=w687, "VI Ref"=w688) -> (error out=w686:errorcluster)  [unwired: 2 in, 3 out]
        n321 = Bundle By Name(cluster=w685, "System Parameters.Active Page"="Profile") -> (w684:T3)
      }
      frame "Subpanel: Load Configuration" {
        n322 = Unbundle By Name(w690) -> ("Configuration.VI Reference"=w694:refnum<vi>)
        n323 = invoke on="Main Subpanel" class="SubPanel" method="Insert VI"(error in=w693, "VI Ref"=w694) -> (error out=w692:errorcluster)  [unwired: 2 in, 3 out]
        n324 = Bundle By Name(cluster=w690, "System Parameters.Active Page"="Configuration") -> (w689:T3)
      }
      frame "Subpanel: Load Acquisition" {
        n325 = Unbundle By Name(w696) -> ("Acquisition.VI Reference"=w700:refnum<vi>)
        n326 = invoke on="Main Subpanel" class="SubPanel" method="Insert VI"(error in=w699, "VI Ref"=w700) -> (error out=w698:errorcluster)  [unwired: 2 in, 3 out]
        n327 = Bundle By Name(cluster=w696, "System Parameters.Active Page"="Acquisition") -> (w695:T3)
      }
      frame "Subpanel: Load Data" {
        n328 = Unbundle By Name(w702) -> ("Data.VI Reference"=w706:refnum<vi>)
        n329 = invoke on="Main Subpanel" class="SubPanel" method="Insert VI"(error in=w705, "VI Ref"=w706) -> (error out=w704:errorcluster)  [unwired: 2 in, 3 out]
        n330 = Bundle By Name(cluster=w702, "System Parameters.Active Page"="Data") -> (w701:T3)
      }
      frame "Subpanel: Load Journal" {
        n331 = Unbundle By Name(w708) -> ("Journal.VI Reference"=w712:refnum<vi>)
        n332 = invoke on="Main Subpanel" class="SubPanel" method="Insert VI"(error in=w711, "VI Ref"=w712) -> (error out=w710:errorcluster)  [unwired: 2 in, 3 out]
        n333 = Bundle By Name(cluster=w708, "System Parameters.Active Page"="Journal") -> (w707:T3)
      }
      frame "Subpanel: Set Splitters" {
        n334 = Unbundle By Name(w717) -> ("Configuration.Queue"=w716:refnum<queue>)
        n335 = Enqueue Element(queue=w716, element=cluster{"Msg":string, "Data":variant} {"Msg"="Set Splitter", "Data"=variant}, error in (no error)=w714) -> (error out=w713:errorcluster)  [unwired: 1 in, 2 out]
      }
      frame "/*** Bluetooth ***/" {
      }
      frame "/*** Menu ***/" {
      }
      frame "Update Program" {
        n336 = call "Update.vi"("error in (no error)"=w724) -> ("error out"=w723:errorcluster, "Update"=w726:bool, "UpdatePath"=w727:string)  [unwired: 8 in]
        n337 = case shown="True" w726 {
          tunnel: w725 -> [_ w741]
          tunnel: w727 -> [_ w734]
          tunnel: w723 -> [w729 w731]
          tunnel: [w729 w730] -> w722
          frame False {
          }
          frame True {
            w733 = "\""
            n338 = Concatenate Strings("cmd /c", w733, w734, w733, "\r\n") -> (w739:string)
            n339 = Temporary Directory() -> (w736:path)
            n340 = call <vilib>:"System Exec.vi"("run minimized? (F)"=TRUE, "wait until completion? (T)"=FALSE, "error in (no error)"=w731, "working directory"=w736, "command line"=w739) -> ("error out"=w732:errorcluster)  [unwired: 3 in, 3 out]
            n341 = call "AMC Send Local Messages.vi"("error in (no error)"=w732, "Message Names"=string[] ["Close SubVI", "Exit"], "Message Queue in"=w741) -> ("error out"=w730:errorcluster)  [unwired: 7 in, 1 out]
          }
        }
      }
      frame "Load Patient Register" {
        n342 = Unbundle By Name(w752) -> ("cRef.Profile.References.ListboxOperator"=w748:refnum<vi>, "cRef.Profile.References.ListboxDoctor"=w747:refnum<vi>, "cRef.Profile.References.Listbox Patient ID"=w751:refnum<vi>)
        n343 = call "ListboxItemsCpr(SubVI).vi"("error in (no error)"=w750, "LstBox Refnum"=w751) -> ("error out"=w745:errorcluster)  [unwired: 8 in, 1 out]
        n344 = call "AE Save.vi"("error in (no error)"=w745, "LstBox Refnum"=w747, "Action"=Enum_Save_Action_Events."Load Listbox") -> ("error out"=w746:errorcluster)  [unwired: 6 in, 1 out]
        n345 = call "AE Save.vi"("error in (no error)"=w746, "LstBox Refnum"=w748, "Action"=Enum_Save_Action_Events."Load Listbox") -> ("error out"=w743:errorcluster)  [unwired: 6 in, 1 out]
      }
      frame "Load Menu" {
        n346 = control-ref of="This VI"() -> (w759:refnum<vi>)
        n347 = Current VI's Path() -> (path=w761:path)
        n348 = Strip Path(path=w761) -> (stripped path=w757:path)  [unwired: 1 out]
        n349 = Build Path(base path=w757, name or relative path="DM2000RuntimeMenu.rtm") -> (appended path=w758:path)
        n350 = property class="VI"(reference=w759, error in=w756, "RT Menu Path"=w758) -> (reference out=w755:refnum<vi>, error out=w754:errorcluster)
        n351 = Close Reference(reference=w755, error in (no error)=w754) -> (error out=w753:errorcluster)
      }
      frame "/****Profile Page***/" {
      }
      frame "KeyDown" {
        n352 = Unbundle By Name(w766) -> ("System Parameters.Active Page"=w765:string)
        n353 = case shown="\"Left\"" w767 {
          tunnel: w768 -> [_ w771 w780 w789]
          tunnel: w765 -> [_ w770 w781 w788]
          frame "0", Default {
          }
          frame "Right" {
            # "Rightarrow"
            n354 = case shown="\"Configuration\"" w770 {
              tunnel: w771 -> [_ w772 w774 w776 w778]
              frame "Profile", Default {
              }
              frame "Configuration" {
                n355 = call "AMC Send Local Messages.vi"("Message Names"=string[] ["Subpanel: Load Acquisition"], "Message Queue in"=w772) -> ()  [unwired: 8 in, 2 out]
              }
              frame "Acquisition" {
                n356 = call "AMC Send Local Messages.vi"("Message Names"=string[] ["Subpanel: Load Data"], "Message Queue in"=w774) -> ()  [unwired: 8 in, 2 out]
              }
              frame "Data" {
                n357 = call "AMC Send Local Messages.vi"("Message Names"=string[] ["Subpanel: Load Journal"], "Message Queue in"=w776) -> ()  [unwired: 8 in, 2 out]
              }
              frame "Journal" {
                n358 = call "AMC Send Local Messages.vi"("Message Names"=string[] ["Subpanel: Load Profile"], "Message Queue in"=w778) -> ()  [unwired: 8 in, 2 out]
              }
            }
          }
          frame "Left" {
            # "Leftarrow"
            n359 = case shown="\"Journal\"" w781 {
              tunnel: w780 -> [_ _ w782 w784 w786]
              frame "Profile", Default {
              }
              frame "Configuration" {
              }
              frame "Acquisition" {
                n360 = call "AMC Send Local Messages.vi"("Message Names"=string[] ["Subpanel: Load Configuration"], "Message Queue in"=w782) -> ()  [unwired: 8 in, 2 out]
              }
              frame "Data" {
                n361 = call "AMC Send Local Messages.vi"("Message Names"=string[] ["Subpanel: Load Acquisition"], "Message Queue in"=w784) -> ()  [unwired: 8 in, 2 out]
              }
              frame "Journal" {
                n362 = call "AMC Send Local Messages.vi"("Message Names"=string[] ["Subpanel: Load Data"], "Message Queue in"=w786) -> ()  [unwired: 8 in, 2 out]
              }
            }
          }
          frame "Space" {
            # "Space"
            n363 = case shown="\"Configuration\"" w788 {
              tunnel: w789 -> [_ w791 w793 w794 _]
              frame "Profile", Default {
              }
              frame "Configuration" {
                n364 = call "AMC Send Local Messages.vi"("Message Names"=string[] ["Subpanel: Load Acquisition"], "Message Queue in"=w791) -> ()  [unwired: 8 in, 2 out]
              }
              frame "Acquisition" {
                n365 = call "AMC Send Local Message.vi"("Message Name"="Subpanel: Load Data", "Message Queue in"=w793) -> ()  [unwired: 8 in, 2 out]
              }
              frame "Data" {
                n366 = call "AMC Send Local Message.vi"("Message Name"="Subpanel: Load Configuration", "Message Queue in"=w794) -> ()  [unwired: 8 in, 2 out]
              }
              frame "Journal" {
              }
            }
          }
        }
      }
      frame "MWL: QueryWorklist" {
        n367 = call "fo_MWLQuery.vi"("error in (no error)"=w803) -> ("error out"=w800:errorcluster, "Cancel?"=w798:bool, "Worklist"=w802:string[][], "SelectedRow"=w801:string[])  [unwired: 7 in]
        n368 = case shown="False" w798 {
          tunnel: [w823 w832] -> w804
          tunnel: w797 -> [w818 w832]
          tunnel: w802 -> [w814 _]
          tunnel: w801 -> [w805 _]
          tunnel: w800 -> [w810 w831]
          tunnel: [w809 w831] -> w799
          tunnel: w797 -> [w806 _]
          tunnel: w796 -> [_ w830]
          frame False {
            n369 = Unbundle By Name(w806) -> ("System Parameters.Date"=w817:string)
            n370 = call "fo_LocatePatientInfo.vi"("subarray"=w805) -> ("PatientId"=w813:string, "PatientName"=w822:string)  [unwired: 9 in]
            n371 = global read "DataPathGlobalVariable.vi" "DataPath"() -> (w820:path)
            n372 = call "Encrypt.vi"("Input"=w813) -> ("Output"=w819:string)  [unwired: 10 in]
            n373 = Build Path(base path=w820, name or relative path=w819) -> (appended path=w808:path)
            n374 = Empty String/Path?(string/path=w813) -> (empty?=w812:bool)
            n375 = Build Path(base path=w808, name or relative path=w817) -> (appended path=w811:path)
            n376 = case shown="False" w812 {
              tunnel: w811 -> [w827 w828]
              tunnel: w810 -> [w826 w829]
              tunnel: [w825 w829] -> w809
              tunnel: [w824 w828] -> w807
              frame False {
                n377 = call <userlib>:"Create Dir if Non-Existant__ogtk.vi"("error in (no error)"=w826, "Directory Path"=w827) -> ("error out"=w825:errorcluster, "dup Directory Path"=w824:path)  [unwired: 7 in, 1 out]
              }
              frame True {
              }
            }
            n378 = call "DICOMFormatToName.vi"("DICOM Format Name"=w822) -> ("Name"=w821:string)  [unwired: 10 in]
            n379 = Build Path(base path=w807, name or relative path="info.dcm") -> (appended path=w815:path)
            n380 = Bundle By Name(cluster=w818, "MWL.Name"=w821, "MWL.PatientID"=w813, "MWL.DICOM Variables"=w805, "MWL.Worklist"=w814, "MWL.DICOM Info"=w815) -> (w823:T3)
          }
          frame True {
            n381 = call "AMC Flush Message Queue.vi"("Message Queue in"=w830) -> ()  [unwired: 8 in, 2 out]
          }
        }
      }
      frame "MWL: PatientID" {
        # "This will put patientID into the listbox and\nthen select that patientID"
        n382 = Unbundle By Name(w838) -> ("cRef.Profile.References.Listbox Patient ID"=w833:refnum<vi>, "MWL.PatientID"=w835:string)
        n383 = Empty String/Path?(string/path=w835) -> (empty?=w834:bool)
        n384 = case shown="False" w834 {
          tunnel: w837 -> [w849 w859]
          tunnel: [w847 w859] -> w836
          tunnel: w835 -> [w843 _]
          tunnel: w833 -> [w839 _]
          frame False {
            # "Already exist?"
            n385 = property class="LstBox (strict)"(reference=w839) -> (reference out=w840:refnum<vi>, "Item Names"=w844:string[])  [unwired: 1 in, 1 out]
            n386 = Search 1D Array(1D array=w844, element=w843) -> (index of element=w842:i32)  [unwired: 1 in]
            n387 = Greater Or Equal To 0?(x=w842) -> (x >= 0?=w841:bool)
            n388 = case shown="False" w841 {
              tunnel: w843 -> [w855 w857]
              tunnel: w849 -> [w850 w858]
              tunnel: [w854 w858] -> w848
              tunnel: [w853 w856] -> w846
              tunnel: [w852 w857] -> w845
              tunnel: w840 -> [w851 w856]
              frame False {
                n389 = call "InsertPatientIDIntoList.vi"("error in (no error)"=w850, "CPR Number"=w855, "ListBox in"=w851) -> ("error out"=w854:errorcluster, "CPR Number Out"=w852:string, "ListBox out"=w853:refnum<vi>)  [unwired: 6 in]
              }
              frame True {
              }
            }
            n390 = call "FocusItemInListbox.vi"("error in (no error)"=w848, "patientID"=w845, "ListBox in"=w846) -> ("error out"=w847:errorcluster)  [unwired: 8 in]
          }
          frame True {
          }
        }
      }
      frame "MWL: Update Data" {
        n391 = Unbundle By Name(w863) -> ("MWL.PatientID"=w860:string, "cRef.Profile.References.Name"=w861:refnum<vi>, "MWL.Name"=w864:string, "User Parameters.Name"=w865:string)  [unwired: 1 out]
        n392 = Empty String/Path?(string/path=w860) -> (empty?=w862:bool)
        n393 = case shown="False" w862 {
          tunnel: w865 -> [w870 _]
          tunnel: w864 -> [w869 _]
          tunnel: w861 -> [w867 _]
          frame False {
            n394 = Empty String/Path?(string/path=w870) -> (empty?=w868:bool)
            n395 = case shown="True" w868 {
              tunnel: w869 -> [_ w871]
              tunnel: w867 -> [_ w872]
              frame False {
              }
              frame True {
                n396 = property class="Str"(reference=w872, "Val(Sgnl)"=w871) -> ()  [unwired: 1 in, 2 out]
              }
            }
          }
          frame True {
          }
        }
      }
      frame "DCM: Create Export Path" {
        # "patient id and date"
        # "Search existing journal"
        n397 = Unbundle By Name(w889) -> ("User Parameters.CPR Number"=w885:string, "Database.ActiveItemTag"=w893:string)
        n398 = global read "DataPathGlobalVariable.vi" "DataPath"() -> (w896:path)
        n399 = global read "DataPathGlobalVariable.vi" "ReportPath"() -> (w883:path)
        n400 = call "Encrypt.vi"("Input"=w885) -> ("Output"=w890:string)  [unwired: 10 in]
        n401 = xnode "Match Regular Expression"("input string"=w893, "regular expression"="[0-9]+[-][0-9]+[-][0-9]+", "error in"=w876) -> ("whole match"=w884:string, "error out"=w874:errorcluster)  [unwired: 3 in, 3 out]
        n402 = Build Path(base path=w896, name or relative path=w890) -> (appended path=w892:path)
        n403 = call <vilib>:"Space Constant.vi"() -> ("String"=w886:string)
        n404 = List Folder(path=w883, error in=w876) -> (filenames=w880:string[], error out=w873:errorcluster)  [unwired: 2 in, 2 out]
        n405 = Build Path(base path=w892, name or relative path=w884) -> (appended path=w895:path)
        n406 = Concatenate Strings(w885, w886, w884) -> (w882:string)
        n407 = Build Path(base path=w895, name or relative path="info.dcm") -> (appended path=w887:path)
        n408 = while {
          tunnel: w880 -> [w905] mode=indexing
          tunnel: w882 -> [w908]
          tunnel: [w905] -> w881
          tunnel: w880 -> [w904]
          tunnel: [w899] -> w877
          i -> [w903]
          stop <- w901 stop-if-true
          n409 = Array Size(array=w904) -> (size(s)=w902:i32)
          n410 = xnode "Match Regular Expression"("input string"=w905, "regular expression"=w908) -> ("offset past match"=w907:i32)  [unwired: 4 in, 4 out]
          n411 = Less?(x=w902, y=w903) -> (x < y?=w899:bool)
          n412 = Greater?(x=w907, y=0) -> (0:w900:bool)
          n413 = Or(x=w900, y=w899) -> (x .or. y?=w901:bool)
        }
        n414 = Build Path(base path=w883, name or relative path=w881) -> (appended path=w879:path)
        n415 = Merge Errors(w873, w874) -> (w875:errorcluster)
        n416 = case shown="False" w877 {
          tunnel: [w897 path "" ("appended path")] -> w878
          tunnel: w879 -> [w897 _]
          frame False {
          }
          frame True {
          }
        }
        n417 = Bundle By Name(cluster=w889, "Database.JournalPath"=w878, "MWL.DICOM Info"=w887) -> (w888:T3)
      }
      frame "DCM: Export Journal" {
        n418 = Unbundle By Name(w1137) -> ("Database.JournalPath"=w1135:path, "MWL.DICOM Info"=w1136:path)
        n419 = Empty String/Path?(string/path=w1135) -> (empty?=w1134:bool)
        n420 = call-poly <userlib>:"File Exists__ogtk.vi"("file path"=w1136) -> ("exists"=w1131:bool)  [unwired: 6 in, 1 out]
        n421 = Not(x=w1134) -> (.not. x?=w1133:bool)
        n422 = And(x=w1133, y=w1131) -> (x .and. y?=w1132:bool)
        n423 = case shown="True" w1132 {
          tunnel: w1139 -> [w1141 w1155]
          tunnel: [w1141 w1154] -> w1138
          tunnel: w1135 -> [_ w1145]
          tunnel: w1136 -> [_ w1144]
          frame False {
            n424 = One Button Dialog(message="To generate a DICOM file it is neccessary to acquire study information from the Worklist beforehand or generate DICOM values manually. It is also neccessary to generate a journal beforehand by using the button to the left.") -> ()  [unwired: 1 in, 1 out]
          }
          frame True {
            n425 = Unbundle By Name(T17 {"HospInfo"={"Name"="", "Address"="", "Department"=""}, "Pressure"={"Pressure"=0.0}, "DataPath"={"DataPath"=path ""}, "ReportPath"={"Path"=path "", "Name"=""}, "DICOM Info WL"={"port"=0, "AEtitle"="", "host"="", "remoteAE"=""}, "DICOM Info PACS"={"port"=0, "AEtitle"="", "host"="", "remoteAE"=""}, "ArmCalcMethod"=0.0, "itemTags"=[], "DicomEncoding"=0, "JournalType"=0, "General Settings"={"Hyphenation"=FALSE, "Language"=0, "CellStr1"="", "CellStr2"=""}, "Dicom Tags"=[], "BT Serial"=[], "BT License"={"License"="", "Accepted Serials"=[]}} ("Data")) -> ("DICOM Info PACS"=w1156:T24)
            n426 = call "AE Save.vi"("error in (no error)"=w1155, "Action"=Enum_Save_Action_Events."LoadDICOMInfoPACS") -> ("error out"=w1159:errorcluster, "Anything"=w1158:variant)  [unwired: 7 in]
            n427 = Variant To Data(error in=w1159, type=w1156, Variant=w1158) -> (data=w1153:T24, error out=w1152:errorcluster)
            n428 = call <vilib>:"Set Busy.vi"("error in (no error)"=w1152) -> ("error out"=w1151:errorcluster)  [unwired: 9 in, 1 out]
            n429 = call "fo_ExcelToDcm.vi"("DICOM Info"=w1144, "error in (no error)"=w1151, "JournalPath"=w1145, "ServerInfo"=w1153) -> ("error out"=w1148:errorcluster, "No active excel error"=w1143:bool)  [unwired: 6 in]
            n430 = call-poly <userlib>:"MGI Suppress Error Code.vi"("Error Code"=51000, "Error In"=w1148) -> ("Error Supressed?"=w1146:bool, "Error Out"=w1149:errorcluster)  [unwired: 4 in]
            n431 = call <vilib>:"Unset Busy.vi"("error in (no error)"=w1149) -> ("error out"=w1150:errorcluster)  [unwired: 10 in]
            n432 = case shown="True" w1143 {
              tunnel: w1150 -> [w1162 w1163]
              tunnel: [w1162 w1163] -> w1154
              frame False {
              }
              frame True {
                n433 = One Button Dialog(message="Cannot connect to Excel. Please make sure that Excel is running. ") -> ()  [unwired: 1 in, 1 out]
              }
            }
            n434 = case shown="True" w1146 {
              tunnel: "Some error: 51000" ("VerificationFailure") -> [_ w1161]
              frame False {
              }
              frame True {
                n435 = One Button Dialog(message=w1161) -> ()  [unwired: 1 in, 1 out]
              }
            }
          }
        }
      }
      frame "DCM: Load DICOM Info" {
        n436 = Unbundle By Name(w1166) -> ("MWL.DICOM Info"=w1165:path)
        n437 = call-poly <userlib>:"File Exists__ogtk.vi"("file path"=w1165) -> ("exists"=w1169:bool)  [unwired: 6 in, 1 out]
        n438 = Empty String/Path?(string/path=w1165) -> (empty?=w1168:bool)
        n439 = Implies(1:w1168, 2:w1169) -> (0:w1167:bool)
        n440 = case shown="False" w1167 {
          tunnel: w1166 -> [w1179 w1183]
          tunnel: [w1178 w1182] -> w1172
          tunnel: w1165 -> [w1177 w1180]
          tunnel: w1171 -> [w1175 w1184]
          tunnel: [w1174 w1184] -> w1170
          frame False {
            n441 = Path To String(path=w1177) -> (string=w1176:string)
            n442 = call "fo_DumpDataset.vi"("error in (no error)"=w1175, "file"=w1176) -> ("error out"=w1174:errorcluster, "items"=w1173:string[])  [unwired: 6 in, 2 out]
            n443 = Bundle By Name(cluster=w1179, "MWL.DICOM Info"=w1177, "MWL.DICOM Variables"=w1173) -> (w1178:T3)
          }
          frame True {
            n444 = Bundle By Name(cluster=w1183, "MWL.DICOM Info"=w1180, "MWL.DICOM Variables"=string[] []) -> (w1182:T3)
          }
        }
      }
      frame "DCM: Show Values" {
        n445 = Unbundle By Name(w1189) -> ("MWL.DICOM Info"=w1186:path)
        n446 = call-poly <userlib>:"File Exists__ogtk.vi"("file path"=w1186) -> ("exists"=w1185:bool)  [unwired: 6 in, 1 out]
        n447 = case shown="True" w1185 {
          tunnel: w1188 -> [w1191 w1198]
          tunnel: [w1191 w1200] -> w1187
          tunnel: w1186 -> [_ w1199]
          frame False {
            n448 = One Button Dialog(message="No DICOM files found") -> ()  [unwired: 1 in, 1 out]
          }
          frame True {
            n449 = Path To String(path=w1199) -> (string=w1196:string)
            n450 = call "fo_DumpDataset.vi"("error in (no error)"=w1198, "file"=w1196) -> ("error out"=w1197:errorcluster, "items"=w1193:string[], "keywords"=w1194:string[], "tags"=w1195:string[])  [unwired: 6 in]
            n451 = Build Array(w1195, w1194, w1193) -> (w1192:string[][])
            n452 = call "ShowDicomValues.vi"("error in (no error)"=w1197, "Array"=w1192) -> ("error out"=w1200:errorcluster)  [unwired: 9 in]
          }
        }
      }
      frame "DCM: Update Variables" {
        n453 = Unbundle By Name(w1207) -> ("MWL.DICOM Variables"=w1201:string[], "User Parameters.Name"=w1205:string, "User Parameters.CPR Number"=w1204:string, "User Parameters.Operator"=w1202:string)
        n454 = call "InputDICOMVariables.vi"("values"=w1201, "Operator"=w1202, "CPR Number"=w1204, "Name"=w1205) -> ("Array"=w1203:string[])  [unwired: 7 in]
        n455 = Bundle By Name(cluster=w1207, "MWL.DICOM Variables"=w1203) -> (w1206:T3)
      }
      frame "LoadNameCpr" {
        n456 = Unbundle By Name(w1219) -> ("cRef.Profile.References"=w1217:T25, "cRef.Profile.References.Listbox Patient ID"=w1218:refnum<vi>, "System Parameters.Date"=w1210:string)
        n457 = property class="LstBox (strict)"(reference=w1218, error in=w1229) -> (error out=w1221:errorcluster, "Item Names"=w1232:string[], "Value"=w1231:i32)  [unwired: 1 out]
        n458 = Index Array(array=w1232, index=w1231) -> (element=w1222:string)
        n459 = global read "DataPathGlobalVariable.vi" "DataPath"() -> (w1230:path)
        n460 = call "Encrypt.vi"("Input"=w1222) -> ("Output"=w1223:string)  [unwired: 10 in]
        n461 = Build Path(base path=w1230, name or relative path=w1223) -> (appended path=w1211:path)
        n462 = Build Path(base path=w1211, name or relative path=w1210) -> (appended path=w1209:path)
        n463 = global write "DataPathGlobalVariable.vi" "DataPatientDatePath"(w1209) -> ()
        n464 = global write "DataPathGlobalVariable.vi" "DataPatientPath"(w1211) -> ()
        n465 = Unbundle By Name(w1217) -> ("Name"=w1216:refnum<vi>, "ListboxOperator"=w1215:refnum<vi>, "ListboxDoctor"=w1214:refnum<vi>, "CommentStr"=w1213:refnum<vi>)
        n466 = call "LoadProfileInfo.vi"("error in (no error)"=w1221, "DataPatientPath"=w1211) -> ("error out"=w1220:errorcluster, "Doctor"=w1225:string, "Operator"=w1226:string, "Name"=w1227:string, "Comment"=w1224:string)  [unwired: 5 in]
        n467 = Bundle("Name"=w1216, "ListboxOperator"=w1215, "ListboxDoctor"=w1214, "CommentStr"=w1213, "Name"=w1227, "Operator"=w1226, "Doctor"=w1225, "Comment"=w1224) -> (w1212:T26)  [unwired: 1 in]
        n468 = call "UpdateProfile.vi"("error in"=w1220, "cluster"=w1212) -> ("error out"=w1228:errorcluster)  [unwired: 5 in]
      }
      frame "Load Armpressure" {
        n469 = Unbundle By Name(w1239) -> ("Configuration.Queue"=w1238:refnum<queue>)
        n470 = Bundle By Name(cluster=cluster{"Msg":string, "Data":variant} {"Msg"="", "Data"=variant} ("element"), "Msg"="Load Arm Pressure") -> (w1235:cluster{"Msg":string, "Data":variant})
        n471 = Enqueue Element(queue=w1238, element=w1235, error in (no error)=w1237) -> (error out=w1236:errorcluster)  [unwired: 1 in, 2 out]
      }
      frame "AddCpr" {
        n472 = Unbundle By Name(w1241) -> ("cRef.Profile.References.Listbox Patient ID"=w1240:refnum<vi>)
        n473 = call "TypeCPRNum(SubVI).vi"() -> ("CprOut"=w1243:string, "Boolean"=w1244:bool)  [unwired: 2 in]
        n474 = property class="LstBox (strict)"(reference=w1240, error in=w1247) -> (reference out=w1242:refnum<vi>, error out=w1246:errorcluster, "Item Names"=w1248:string[])
        n475 = case shown="False" w1244 {
          tunnel: w1248 -> [w1263 _]
          tunnel: w1242 -> [w1262 _]
          tunnel: w1246 -> [w1257 w1266]
          tunnel: w1243 -> [w1250 _]
          tunnel: [w1260 w1266] -> w1245
          frame False {
            w1255 = 10 items=["No error", "Argument error", "Memory is full", "Out of zone", "End of file", "File already open", "Generic file I/O error", "File not found", "File permission error", "Disk is full", "Duplicate path", "Too many files open", "System feature not enabled", "Resource file not found", "Cannot add resource", "Resource not found", "Image not found", "Image memory error", "Pen does not exist", "Config type invalid", "Config token not found", "Config parse error", "Config memory error", "Bad external code format", "Bad external code offset", "External code not present", "Null window", "Destroy window error", "Null menu", "Print aborted", "Bad print record", "Print driver error", "Windows error during printing", "Memory error during printing", "Print dialog error", "Generic print error", "Invalid device refnum", "Device not found", "Device parameter error", "Device unit error", "Cannot open device", "Device call aborted", "Generic error", "Cancelled by user", "Object ID too low", "Object ID too high", "Object not in heap", "Unknown heap", "Unknown object (invalid DefProc)", "Unknown object (DefProc not in table)", "Message out of range", "Invalid (null) method", "Unknown message", "Manager call not supported", "Bad address", "Network operation in progress", "Network operation timed out", "Connection is busy", "Network attribute not supported", "Network error", "Address in use", "System out of memory", "Connection aborted", "Connection refused", "Not connected", "Already connected", "Connection closed", "Initialization error (interapplication manager)", "Bad occurrence", "Wait on unbound occurrence handler", "Occurrence queue overflow", "Datalog type conflict", "Unused", "Unrecognized type (interapplication manager)", "Memory corrupt", "Failed to make temporary DLL", "Old CIN version", "Drag socket not found", "Failed to load drop-object", "Failed to register OLE object", "Failed to release OLE object", "Format specifier type mismatch", "Unknown format specifier", "Too few format specifiers", "Too many format specifiers", "Scan failed", "Newer CIN version", "OLE Convert", "Runtime menu error", "Password tampered", "Unknown error code"] ("Error Code")
            # "If CPR number exists, suppress error\nand display message"
            # "Create new folder"
            n476 = global read "DataPathGlobalVariable.vi" "DataPath"() -> (w1261:path)
            n477 = Insert Into Array(array=w1263, index=0, new element=w1250) -> (w1253:string[])
            n478 = call "Encrypt.vi"("Input"=w1250) -> ("Output"=w1249:string)  [unwired: 10 in]
            n479 = Build Path(base path=w1261, name or relative path=w1249) -> (appended path=w1256:path)
            n480 = Create Folder(path (use dialog)=w1256, error in=w1257) -> (error out=w1258:errorcluster)  [unwired: 1 in, 2 out]
            n481 = property class="LstBox (strict)"(reference=w1262, error in=w1258, "Item Names"=w1253, "Val(Sgnl)"=0 ("Value (Signaling)")) -> (error out=w1259:errorcluster)  [unwired: 1 out]
            n482 = call-poly <userlib>:"MGI Suppress Error Code.vi"("Error Code"=w1255, "Error In"=w1259) -> ("Error Supressed?"=w1254:bool, "Error Out"=w1260:errorcluster)  [unwired: 4 in]
            n483 = case shown="True" w1254 {
              frame False {
              }
              frame True {
                n484 = One Button Dialog(message="The CPR number already exists", button name ("OK")="Close") -> ()  [unwired: 1 out]
              }
            }
          }
          frame True {
            # "Cancel true?"
          }
        }
      }
      frame "EditHospInfo" {
        n485 = Unbundle By Name(w1268) -> ("Profile.Queue"=w1267:refnum<queue>)
        n486 = call "SaveHospInfo.vi"() -> ("Cancel?"=w1271:bool, "Department 2"=w1272:string, "Hospital Address 2"=w1273:string, "Hospital Name 2"=w1274:string)  [unwired: 8 in]
        n487 = case shown="False" w1271 {
          tunnel: w1274 -> [w1285 _]
          tunnel: w1273 -> [w1284 _]
          tunnel: w1272 -> [w1283 _]
          tunnel: [w1279 w1287] -> w1270
          tunnel: w1269 -> [w1281 w1287]
          tunnel: w1267 -> [w1278 _]
          frame False {
            n488 = Bundle("Hospital Name 2"=w1285, "Hospital Address 2"=w1284, "Department 2"=w1283) -> (w1282:T27)  [unwired: 1 in]
            n489 = To Variant(anything=w1282) -> (Variant=w1276:variant)
            n490 = call "AE Save.vi"("error in (no error)"=w1281, "Variant In"=w1276, "Action"=Enum_Save_Action_Events."SaveHospInfo") -> ("error out"=w1280:errorcluster)  [unwired: 6 in, 1 out]
            n491 = Bundle By Name(cluster=cluster{"Msg":string, "Data":variant} {"Msg"="Load Hospital Info", "Data"=variant} ("element"), "Data"=w1276) -> (w1275:cluster{"Msg":string, "Data":variant})
            n492 = Enqueue Element(queue=w1278, element=w1275, error in (no error)=w1280) -> (error out=w1279:errorcluster)  [unwired: 1 in, 2 out]
          }
          frame True {
          }
        }
      }
      frame "Load Hospital Info" {
        n493 = Unbundle By Name(w1292) -> ("Profile.Queue"=w1291:refnum<queue>)
        n494 = Enqueue Element(queue=w1291, element=cluster{"Msg":string, "Data":variant} {"Msg"="Load Hospital Info", "Data"=variant}, error in (no error)=w1289) -> (error out=w1288:errorcluster)  [unwired: 1 in, 2 out]
      }
      frame "RemoveCpr" {
        n495 = global read "DataPathGlobalVariable.vi" "DataPath"() -> (w1300:path)
        n496 = Unbundle By Name(w1294) -> ("cRef.Profile.References.Listbox Patient ID"=w1293:refnum<vi>)
        n497 = call "Encrypt.vi"("Input"=w1299) -> ("Output"=w1301:string)  [unwired: 10 in]
        n498 = Build Path(base path=w1300, name or relative path=w1301) -> (appended path=w1295:path)
        n499 = call-poly <userlib>:"File Exists__ogtk.vi"("file path"=w1295) -> ("is directory"=w1297:bool, "exists"=w1296:bool)  [unwired: 6 in]
        n500 = And(x=w1297, y=w1296) -> (x .and. y?=w1298:bool)
        n501 = case shown="True" w1298 {
          tunnel: [w1306 w1313] -> w1305
          tunnel: w1304 -> [w1306 w1312]
          tunnel: [w1307 w1311] -> w1302
          tunnel: w1299 -> [w1307 w1309]
          tunnel: w1295 -> [_ w1310]
          tunnel: w1293 -> [_ w1308]
          frame False {
          }
          frame True {
            n502 = Concatenate Strings("Do you want to delete patient ID: " ("message"), w1309, " and all the data in the folder?" ("string")) -> (w1316:string)
            n503 = Two Button Dialog(message=w1316, 1:"Cancel" ("F button name (\"Cancel\")"), 2:"Yes" ("T button name (\"OK\")")) -> (T button?=w1319:bool)
            n504 = case shown="True" w1319 {
              tunnel: [w1321 w1326] -> w1313
              tunnel: w1312 -> [w1321 w1325]
              tunnel: [w1320 w1324] -> w1311
              tunnel: w1310 -> [_ w1323]
              tunnel: w1309 -> [w1320 _]
              tunnel: w1308 -> [_ w1322]
              frame False {
              }
              frame True {
                n505 = while {
                  tunnel: [w1332] -> w1327
                  tunnel: w1325 -> [w1331]
                  tunnel: w1323 -> [w1330]
                  stop <- w1328 continue-if-true
                  n506 = Delete(path (use dialog)=w1330, entire hierarchy (F)=TRUE, error in=w1331) -> (deleted path=w1329:path, error out=w1332:errorcluster)  [unwired: 2 in, 1 out]
                  n507 = call-poly <userlib>:"File Exists__ogtk.vi"("file path"=w1329) -> ("exists"=w1328:bool)  [unwired: 6 in, 1 out]
                }
                n508 = call "ListboxItemsCpr(SubVI).vi"("error in (no error)"=w1327, "LstBox Refnum"=w1322) -> ("error out"=w1326:errorcluster, "FirstCpr"=w1324:string)  [unwired: 8 in]
              }
            }
          }
        }
        n509 = Bundle By Name(cluster=w1294, "User Parameters.CPR Number"=w1302) -> (w1303:T3)
      }
      frame "SelectCpr" {
        n510 = Unbundle By Name(w1336) -> ("User Parameters.Name"=w1352:string, "User Parameters.CPR Number"=w1338:string, "cRef.Menu.References.PersonalInfoString"=w1350:refnum<vi>, "System Parameters.Date"=w1337:string, "cRef.Data.References.Menu"=w1346:refnum<vi>, "cRef.Journal.References.Data"=w1345:refnum<vi>, "cRef.Journal.References.Menu"=w1344:refnum<vi>)
        n511 = call "SelectCprRutine.vi"("CPR Number"=w1338, "error in"=w1348, "Journal Menu"=w1344, "Data Listbox"=w1345, "ProcessDataTreeMenu"=w1346) -> ("error out"=w1347:errorcluster)  [unwired: 5 in]
        n512 = global read "DataPathGlobalVariable.vi" "DataPath"() -> (w1343:path)
        n513 = Concatenate Strings(w1352, "\r", w1338) -> (w1349:string)
        n514 = call "Encrypt.vi"("Input"=w1338) -> ("Output"=w1342:string)  [unwired: 10 in]
        n515 = property class="Str"(reference=w1350, "Value"=w1349) -> ()  [unwired: 1 in, 2 out]
        n516 = Build Path(base path=w1343, name or relative path=w1342) -> (appended path=w1341:path)
        n517 = Build Path(base path=w1341, name or relative path=w1337) -> (appended path=w1340:path)
        n518 = Build Path(base path=w1340, name or relative path="info.dcm") -> (appended path=w1334:path)
        n519 = Bundle By Name(cluster=w1336, "MWL.DICOM Info"=w1334) -> (w1335:T3)
      }
      frame "ResetToDefault" {
        n520 = Unbundle By Name(w1353) -> ("Configuration.Queue"=w1357:refnum<queue>, "Journal.Queue"=w1356:refnum<queue>, "Data.Queue"=w1355:refnum<queue>)
        n521 = Enqueue Element(queue=w1355, element=cluster{"Msg":string, "Data":variant} {"Msg"="ResetGraphs", "Data"=variant}, error in (no error)=w1360) -> (error out=w1358:errorcluster)  [unwired: 1 in, 2 out]
        n522 = Build Array(w1357, w1356, w1355) -> (w1354:refnum<queue>[])
        n523 = for {
          tunnel: w1354 -> [w1362] mode=indexing
          n524 = Enqueue Element(queue=w1362, element=cluster{"Msg":string, "Data":variant} {"Msg"="Clear", "Data"=variant}) -> ()  [unwired: 2 in, 3 out]
        }
      }
      frame "Delete: ListboxDoctor" {
        n525 = Unbundle By Name(w1367) -> ("cRef.Profile.References.ListboxDoctor"=w1366:refnum<vi>)
        n526 = Decimal String To Number(string=w1365) -> (number=w1364:i32)  [unwired: 2 in, 1 out]
        n527 = property class="LstBox (strict)"(reference=w1366, error in=w1363) -> (reference out=w1372:refnum<vi>, error out=w1371:errorcluster, "Item Names"=w1374:string[])
        n528 = Delete From Array(array=w1374, index=w1364) -> (array with subset deleted=w1373:string[])  [unwired: 1 in, 1 out]
        n529 = property class="LstBox (strict)"(reference=w1372, error in=w1371, "Item Names"=w1373) -> (reference out=w1368:refnum<vi>, error out=w1370:errorcluster)
        n530 = call "AE Save.vi"("error in (no error)"=w1370, "LstBox Refnum"=w1368, "Action"=Enum_Save_Action_Events."Save Listbox") -> ("error out"=w1375:errorcluster)  [unwired: 6 in, 1 out]
      }
      frame "Delete: ListboxOperator" {
        n531 = Unbundle By Name(w1380) -> ("cRef.Profile.References.ListboxOperator"=w1379:refnum<vi>)
        n532 = Decimal String To Number(string=w1378) -> (number=w1377:i32)  [unwired: 2 in, 1 out]
        n533 = property class="LstBox (strict)"(reference=w1379, error in=w1376) -> (reference out=w1385:refnum<vi>, error out=w1384:errorcluster, "Item Names"=w1387:string[])
        n534 = Delete From Array(array=w1387, index=w1377) -> (array with subset deleted=w1386:string[])  [unwired: 1 in, 1 out]
        n535 = property class="LstBox (strict)"(reference=w1385, error in=w1384, "Item Names"=w1386) -> (reference out=w1381:refnum<vi>, error out=w1383:errorcluster)
        n536 = call "AE Save.vi"("error in (no error)"=w1383, "LstBox Refnum"=w1381, "Action"=Enum_Save_Action_Events."Save Listbox") -> ("error out"=w1388:errorcluster)  [unwired: 6 in, 1 out]
      }
      frame "Add New: ListboxDoctor" {
        n537 = Unbundle By Name(w1390) -> ("cRef.Profile.References.ListboxDoctor"=w1389:refnum<vi>)
        n538 = call "AddName.vi"() -> ("Cancel Indicator"=w1393:bool, "NameString"=w1394:string)  [unwired: 9 in]
        n539 = case shown="False" w1393 {
          tunnel: w1394 -> [w1403 _]
          tunnel: w1392 -> [w1397 w1406]
          tunnel: [w1396 w1406] -> w1391
          tunnel: w1389 -> [w1395 _]
          frame False {
            n540 = property class="LstBox (strict)"(reference=w1395, error in=w1397) -> (reference out=w1405:refnum<vi>, error out=w1399:errorcluster, "Item Names"=w1402:string[])
            n541 = Insert Into Array(array=w1402, new element=w1403) -> (w1404:string[])  [unwired: 1 in]
            n542 = property class="LstBox (strict)"(reference=w1405, error in=w1399, "Item Names"=w1404) -> (reference out=w1400:refnum<vi>, error out=w1398:errorcluster)
            n543 = call "AE Save.vi"("error in (no error)"=w1398, "LstBox Refnum"=w1400, "Action"=Enum_Save_Action_Events."Save Listbox") -> ("error out"=w1396:errorcluster)  [unwired: 6 in, 1 out]
          }
          frame True {
          }
        }
      }
      frame "Add New: ListboxOperator" {
        n544 = Unbundle By Name(w1408) -> ("cRef.Profile.References.ListboxOperator"=w1407:refnum<vi>)
        n545 = call "AddName.vi"() -> ("Cancel Indicator"=w1411:bool, "NameString"=w1412:string)  [unwired: 9 in]
        n546 = case shown="False" w1411 {
          tunnel: w1412 -> [w1421 _]
          tunnel: w1410 -> [w1415 w1424]
          tunnel: [w1414 w1424] -> w1409
          tunnel: w1407 -> [w1413 _]
          frame False {
            n547 = property class="LstBox (strict)"(reference=w1413, error in=w1415) -> (reference out=w1423:refnum<vi>, error out=w1417:errorcluster, "Item Names"=w1420:string[])
            n548 = Insert Into Array(array=w1420, new element=w1421) -> (w1422:string[])  [unwired: 1 in]
            n549 = property class="LstBox (strict)"(reference=w1423, error in=w1417, "Item Names"=w1422) -> (reference out=w1418:refnum<vi>, error out=w1416:errorcluster)
            n550 = call "AE Save.vi"("error in (no error)"=w1416, "LstBox Refnum"=w1418, "Action"=Enum_Save_Action_Events."Save Listbox") -> ("error out"=w1414:errorcluster)  [unwired: 6 in, 1 out]
          }
          frame True {
          }
        }
      }
      frame "FindCprNumber" {
        # "Exclude non-match"
        # "Search for CPR number"
        n551 = Unbundle By Name(w1428) -> ("cRef.Profile.References.Listbox Patient ID"=w1427:refnum<vi>, "cRef.Profile.References.Search Patient ID"=w1426:refnum<vi>)
        n552 = global read "DataPathGlobalVariable.vi" "DataPath"() -> (w1441:path)
        n553 = property class="Str"(reference=w1426) -> ("Value"=w1425:string)  [unwired: 1 in, 2 out]
        n554 = call <userlib>:"List Directory__ogtk.vi"("directory path"=w1441) -> ("directory names"=w1440:string[])  [unwired: 3 in, 3 out]
        n555 = for {
          tunnel: w1440 -> [w1453] mode=indexing
          tunnel: [w1455] -> w1439 mode=indexing
          tunnel: [w1454] -> w1438 mode=indexing
          tunnel: w1425 -> [w1451]
          n556 = call "Decrypt.vi"("Input"=w1453) -> ("Output"=w1452:string)  [unwired: 10 in]
          n557 = String Subset(string=w1452) -> (substring=w1456:string)  [unwired: 2 in]
          n558 = Search/Split String(string=w1456, search string/char (-)=w1451) -> (match + rest of string=w1454:string, offset of match=w1455:i32)  [unwired: 1 in, 1 out]
        }
        n559 = for {
          tunnel: w1439 -> [w1445] mode=indexing
          tunnel: w1438 -> [w1443] mode=indexing
          shift-right: [w1442] -> w1434
          shift-left: string[] [] -> [w1446]
          n560 = Equal To 0?(x=w1445) -> (x = 0?=w1444:bool)
          n561 = case shown="True" w1444 {
            tunnel: [w1447 w1450] -> w1442
            tunnel: w1446 -> [w1447 w1449]
            tunnel: w1443 -> [_ w1448]
            frame False {
            }
            frame True {
              n562 = Build Array (concatenate)(w1449, w1448) -> (w1450:string[])
            }
          }
        }
        n563 = property class="LstBox (strict)"(reference=w1427, error in=w1429, "Item Names"=w1434) -> (reference out=w1435:refnum<vi>, error out=w1436:errorcluster)
        n564 = property class="LstBox (strict)"(reference=w1435, error in=w1436, "Value"=-1 ("Value (Signaling)")) -> (reference out=w1432:refnum<vi>, error out=w1431:errorcluster)
        n565 = Close Reference(reference=w1432, error in (no error)=w1431) -> (error out=w1430:errorcluster)
      }
      frame "/*** Configuration ***/" {
      }
      frame "Change Segment" {
        n566 = Unbundle By Name(w1467) -> ("cRef.Configuration.References.ListboxMeasurementArea"=w1466:refnum<vi>)
        n567 = property class="LstBox (strict)"(reference=w1466, error in=w1461) -> (reference out=w1465:refnum<vi>, error out=w1459:errorcluster, "Item Names"=w1464:string[])
        n568 = Match First String(2:w1464, 3:w1463) -> (0:w1462:i32)  [unwired: 1 out]
        n569 = property class="LstBox (strict)"(reference=w1465, error in=w1459, "Value"=w1462) -> (error out=w1460:errorcluster)  [unwired: 1 out]
      }
      frame "Set Height" {
        n570 = Unbundle By Name(w1470) -> ("cRef.Configuration.References.HeightAdjustmentInt"=w1471:refnum<vi>)
        n571 = property class="DigNum (strict)"(reference=w1471) -> ("Value"=w1468:dbl)  [unwired: 1 in, 2 out]
        n572 = Bundle By Name(cluster=w1470, "Database.Height Adjustment"=w1468) -> (w1469:T3)
        n573 = call "AE Variables.vi"("VariantIn"=w1468, "Action"=Enum_Variables."Set Height") -> ()  [unwired: 10 in, 8 out]
      }
      frame "/******Acquisition******/" {
      }
      frame "Set Acquisition Mode" {
        n574 = call "AE Save.vi"("error in (no error)"=w1484, "Action"=Enum_Save_Action_Events."Load Acquisition Mode") -> ("error out"=w1483:errorcluster, "Anything"=w1480:variant)  [unwired: 7 in]
        n575 = Unbundle By Name(w1482) -> ("Acquisition.Queue"=w1489:refnum<queue>)
        n576 = Bundle By Name(cluster=cluster{"Msg":string, "Data":variant} {"Msg"="", "Data"=variant} ("element"), "Msg"="Set Mode", "Data"=w1480) -> (w1486:cluster{"Msg":string, "Data":variant})
        n577 = Enqueue Element(queue=w1489, element=w1486, error in (no error)=w1483) -> (error out=w1477:errorcluster)  [unwired: 1 in, 2 out]
        n578 = Variant To Data(error in=w1477, type=FALSE, Variant=w1480) -> (data=w1478:bool, error out=w1476:errorcluster)
        n579 = Bundle By Name(cluster=w1482, "Data Acquisition.Control?"=w1478) -> (w1481:T3)
      }
      frame "Query DAQ Availability" {
        n580 = Unbundle By Name(w1498) -> ("Acquisition.Queue"=w1490:refnum<queue>, "cRef.Menu.References.MenuStartADC"=w1495:refnum<vi>)
        n581 = call "availableDAQ.vi"("error in (no error)"=w1492) -> ("error out"=w1493:errorcluster, "DAQmx Device Name"=w1497:tag)  [unwired: 9 in]
        n582 = Empty String/Path?(string/path=w1497) -> (empty?=w1496:bool)
        n583 = case shown="True" w1496 {
          tunnel: w1495 -> [_ w1522]
          tunnel: w1494 -> [w1502 w1520]
          tunnel: w1493 -> [w1501 w1519]
          tunnel: [w1500 w1518] -> w1491
          tunnel: w1490 -> [w1499 _]
          frame False {
            n584 = call "AE Variables.vi"("error in (no error)"=w1501, "Action"=Enum_Variables."Get DAQ Connected") -> ("BooleanOut"=w1503:bool, "error out"=w1505:errorcluster)  [unwired: 10 in, 6 out]
            n585 = case shown="False" w1503 {
              tunnel: [w1506 w1515] -> w1500
              tunnel: w1505 -> [w1507 w1516]
              tunnel: w1502 -> [w1508 w1517]
              tunnel: w1499 -> [w1513 _]
              frame False {
                n586 = Enqueue Element(queue=w1513, element=cluster{"Msg":string, "Data":variant} {"Msg"="Initialize DAQ", "Data"=variant}, error in (no error)=w1507) -> (error out=w1511:errorcluster)  [unwired: 1 in, 2 out]
                n587 = call "AE Variables.vi"("VariantIn"=TRUE, "error in (no error)"=w1511, "Action"=Enum_Variables."Set DAQ Connected") -> ("error out"=w1506:errorcluster)  [unwired: 9 in, 7 out]
                n588 = call "AMC Send Local Messages.vi"("Message Names"=string[] ["Initialize Reference", "Monitor Reference", "Update Display"], "Message Queue in"=w1508) -> ()  [unwired: 8 in, 2 out]
              }
              frame True {
                # "If DAQ is already active\nignore commands"
                n589 = call "AMC Flush Message Queue.vi"("error in (no error)"=w1516, "Message Queue in"=w1517) -> ("error out"=w1515:errorcluster)  [unwired: 7 in, 1 out]
              }
            }
          }
          frame True {
            n590 = call "AMC Flush Message Queue.vi"("Message Queue in"=w1520) -> ()  [unwired: 8 in, 2 out]
            n591 = property class="Bool (strict)"(reference=w1522, error in=w1519, "Value"=FALSE) -> (error out=w1518:errorcluster)  [unwired: 1 out]
            n592 = One Button Dialog(message="The USB interface cannot be registered. Please connect") -> ()  [unwired: 1 in, 1 out]
          }
        }
      }
      frame "Silent DAQ Initialization" {
        n593 = Unbundle By Name(w1532) -> ("Acquisition.Queue"=w1525:refnum<queue>, "cRef.Menu.References.MenuStartADC"=w1524:refnum<vi>)
        n594 = call "availableDAQ.vi"("error in (no error)"=w1527) -> ("error out"=w1528:errorcluster, "DAQmx Device Name"=w1531:tag)  [unwired: 9 in]
        n595 = Empty String/Path?(string/path=w1531) -> (empty?=w1530:bool)
        n596 = case shown="True" w1530 {
          tunnel: w1524 -> [w1542 w1550]
          tunnel: w1529 -> [w1537 _]
          tunnel: w1528 -> [w1543 w1549]
          tunnel: w1525 -> [w1544 _]
          tunnel: [w1533 w1546] -> w1526
          frame False {
            n597 = property class="Bool (strict)"(reference=w1542, "Value"=TRUE) -> ()  [unwired: 1 in, 2 out]
            n598 = call "AMC Send Local Messages.vi"("Message Names"=string[] ["Initialize Reference", "Monitor Reference"], "Message Queue in"=w1537) -> ()  [unwired: 8 in, 2 out]
            n599 = Enqueue Element(queue=w1544, element=cluster{"Msg":string, "Data":variant} {"Msg"="Initialize DAQ", "Data"=variant}, error in (no error)=w1543) -> (error out=w1538:errorcluster)  [unwired: 1 in, 2 out]
            n600 = call "AE Variables.vi"("VariantIn"=TRUE, "error in (no error)"=w1538, "Action"=Enum_Variables."Set DAQ Connected") -> ("error out"=w1534:errorcluster)  [unwired: 9 in, 7 out]
            n601 = call "Notifier AE.vi"("error in (no error)"=w1534, "String"="Starting DAQ") -> ("error out"=w1533:errorcluster)  [unwired: 9 in]
          }
          frame True {
            w1548 = FALSE ("Value")
            n602 = property class="Bool (strict)"(reference=w1550, error in=w1549, "Value"=w1548) -> (error out=w1546:errorcluster)  [unwired: 1 out]
            n603 = call "AE Variables.vi"("VariantIn"=w1548, "Action"=Enum_Variables."Set DAQ Connected") -> ()  [unwired: 10 in, 8 out]
          }
        }
      }
      frame "Send Segment to Acquisition" {
        n604 = Unbundle By Name(w1558) -> ("Acquisition.Queue"=w1557:refnum<queue>, "User Parameters.Measuring Limb"=w1554:string)
        n605 = Bundle By Name(cluster=cluster{"Msg":string, "Data":variant} {"Msg"="", "Data"=variant} ("element"), "Msg"="Set Segment", "Data"=w1554) -> (w1556:cluster{"Msg":string, "Data":variant})
        n606 = Enqueue Element(queue=w1557, element=w1556, error in (no error)=w1552) -> (error out=w1551:errorcluster)  [unwired: 1 in, 2 out]
      }
      frame "Regulation Stopped" {
        n607 = Unbundle By Name(w1563) -> ("Acquisition.Queue"=w1562:refnum<queue>)
        n608 = Enqueue Element(queue=w1562, element=cluster{"Msg":string, "Data":variant} {"Msg"="Control: Regulation Stopped", "Data"=variant}, error in (no error)=w1560) -> (error out=w1559:errorcluster)  [unwired: 1 in, 2 out]
      }
      frame "AcqTest" {
        n609 = Unbundle By Name(w1567) -> ("Acquisition.Queue"=w1566:refnum<queue>)
        n610 = flat-sequence {
          tunnel: w1566 -> [w1572]
          tunnel: [w1571] -> w1564
          tunnel: w1569 -> [w1575]
          tunnel: [w1575] -> w1568
          tunnel: [w1573] -> w1565
          tunnel: w1564 -> [w1573]
          tunnel: w1565 -> [w1577]
          frame #0 {
            n611 = Enqueue Element(queue=w1572, element=cluster{"Msg":string, "Data":variant} {"Msg"="Test", "Data"=variant}) -> (queue out=w1571:refnum<queue>)  [unwired: 2 in, 2 out]
          }
          frame #1 {
            n612 = Wait (ms)(milliseconds to wait=u32 10000) -> ()  [unwired: 1 out]
          }
          frame #2 {
            n613 = Enqueue Element(queue=w1577, element=cluster{"Msg":string, "Data":variant} {"Msg"="Idle", "Data"=variant}) -> ()  [unwired: 2 in, 3 out]
          }
        }
      }
      frame "Monitor Reference" {
        n614 = Unbundle By Name(w1582) -> ("Reference signal.Queue"=w1580:refnum<queue>, "Data Acquisition.Control?"=w1578:bool)
        n615 = case shown="False" w1578 {
          tunnel: w1581 -> [w1590 w1591]
          tunnel: w1580 -> [w1586 _]
          tunnel: [w1583 w1591] -> w1579
          frame False {
            n616 = call "AE Paper.vi"("error in (no error)"=w1590, "Action Events"=Enum_Paper_Action_Events."Init") -> ("error out"=w1588:errorcluster)  [unwired: 7 in, 1 out]
            n617 = call "AE Events.vi"("error in (no error)"=w1588, "Action"=enum16{"Init", "Get Event", "Set Event"}."Init") -> ("error out"=w1585:errorcluster)  [unwired: 8 in, 1 out]
            n618 = Enqueue Element(queue=w1586, element="Start", error in (no error)=w1585) -> (error out=w1583:errorcluster)  [unwired: 1 in, 2 out]
          }
          frame True {
          }
        }
      }
      frame "Idle Monitor Reference" {
        n619 = Unbundle By Name(w1596) -> ("Reference signal.Queue"=w1594:refnum<queue>, "Data Acquisition.Control?"=w1592:bool)
        n620 = case shown="False" w1592 {
          tunnel: w1595 -> [w1599 w1601]
          tunnel: w1594 -> [w1598 _]
          tunnel: [w1597 w1601] -> w1593
          frame False {
            n621 = Enqueue Element(queue=w1598, element="Idle", error in (no error)=w1599) -> (error out=w1597:errorcluster)  [unwired: 1 in, 2 out]
          }
          frame True {
          }
        }
      }
      frame "Stop Monitor Reference" {
        n622 = Unbundle By Name(w1606) -> ("Reference signal.Queue"=w1604:refnum<queue>, "Data Acquisition.Control?"=w1602:bool)
        n623 = case shown="True" w1602 {
          tunnel: w1605 -> [w1607 w1610]
          tunnel: w1604 -> [_ w1609]
          tunnel: [w1607 w1608] -> w1603
          frame False {
          }
          frame True {
            n624 = Enqueue Element(queue=w1609, element="Stop", error in (no error)=w1610) -> (error out=w1608:errorcluster)  [unwired: 1 in, 2 out]
          }
        }
      }
      frame "CreateLogPath" {
        # "Store data to local temporary directory"
        n625 = Unbundle By Name(w1621) -> ("User Parameters.CPR Number"=w1622:string, "User Parameters.Measuring Limb"=w1619:string)
        n626 = call "DataFileName(SubVI).vi"("error in (no error)"=w1618, "Segment"=w1619, "CPR"=w1622) -> ("error out"=w1617:errorcluster, "Relative path"=w1612:path, "Path"=w1613:path)  [unwired: 2 in]
        n627 = Temporary Directory() -> (w1616:path)
        n628 = Build Path(base path=w1616, name or relative path="data.tdms") -> (appended path=w1614:path)
        n629 = Bundle By Name(cluster=w1621, "Data Acquisition.RecordPath"=w1613, "Data Acquisition.RelativeRecordPath"=w1612) -> (w1620:T3)
        n630 = global write "DataAcqRecordPathGlobal.vi" "DataAcqRecordPath"(w1614) -> ()
      }
      frame "Acquisition" {
        # "Set the start of acquisition"
        n631 = Unbundle By Name(w1628) -> ("Acquisition.Queue"=w1627:refnum<queue>)
        n632 = Enqueue Element(queue=w1627, element=cluster{"Msg":string, "Data":variant} {"Msg"="Acquire", "Data"=variant}, error in (no error)=w1626) -> (error out=w1625:errorcluster)  [unwired: 1 in, 2 out]
        n633 = Get Date/Time In Seconds() -> (seconds since 1Jan1904=w1629:timestamp)
        n634 = Bundle By Name(cluster=w1628, "Data Acquisition.Duration"=w1629, "Data Acquisition.Acquisition"=TRUE) -> (w1630:T3)
      }
      frame "Stop Acquisition" {
        n635 = call "removeShortMeasurement.vi"("error in (no error)"=w1633, "Queue in"=w1631, "SHIFTER DATA"=w1632) -> ("error out"=w1634:errorcluster)  [unwired: 8 in]
        n636 = Bundle By Name(cluster=w1632, "Data Acquisition.Acquisition"=FALSE) -> (w1636:T3)
      }
      frame "LogData" {
        n637 = Unbundle By Name(w1644) -> ("Data Acquisition.RecordPath"=w1641:path, "User Parameters.Measuring Type"=w1640:string, "User Parameters.Measuring Technique"=w1643:string, "User Parameters.Measuring Limb"=w1639:string, "Database.Height Adjustment"=w1638:dbl)
        n638 = Empty String/Path?(string/path=w1641) -> (empty?=w1642:bool)
        n639 = Number To Decimal String(number=w1638) -> (decimal integer string=w1637:string)  [unwired: 1 in]
        n640 = case shown="False" w1642 {
          tunnel: w1643 -> [w1657 _]
          tunnel: w1641 -> [w1649 _]
          tunnel: w1640 -> [w1648 _]
          tunnel: w1639 -> [w1647 _]
          tunnel: w1637 -> [w1646 _]
          frame False {
            n641 = Build Array(w1648, w1657, w1647, w1646) -> (w1651:string[])
            n642 = Strip Path(path=w1649) -> (stripped path=w1650:path)  [unwired: 1 out]
            n643 = Build Path(base path=w1650, name or relative path=T18 "patientdata.dm2000") -> (appended path=w1652:path)
            n644 = call-poly <vilib>:"Write To Spreadsheet File.vi"("delimiter (\\t)"="," ("delimiter (\\t)"), "format (%s)"="%s", "append to file? (new file:F)"=FALSE, "1D data"=w1651, "file path (dialog if empty)"=w1652) -> ()  [unwired: 3 in, 1 out]
          }
          frame True {
          }
        }
      }
      frame "AddTreeItems" {
        n645 = Unbundle By Name(w1666) -> ("cRef.Journal.References.Menu"=w1658:refnum<vi>, "cRef.Data.References.Menu"=w1660:refnum<vi>, "Data Acquisition.RecordPath"=w1659:path)
        n646 = call <vilib>:"Check if File or Folder Exists.vi"("error in (no error)"=w1663, "path"=w1659) -> ("error out"=w1664:errorcluster, "file or folder exists?"=w1662:bool, "dup path"=w1661:path)  [unwired: 7 in]
        n647 = case shown="True" w1662 {
          tunnel: w1664 -> [w1670 w1680]
          tunnel: [w1669 w1682] -> w1665
          tunnel: w1661 -> [w1668 w1681]
          tunnel: w1660 -> [_ w1678]
          tunnel: w1658 -> [_ w1677]
          frame False {
            n648 = Empty String/Path?(string/path=w1668) -> (empty?=w1667:bool)
            n649 = case shown="False" w1667 {
              tunnel: w1670 -> [w1673 w1676]
              tunnel: [w1672 w1676] -> w1669
              tunnel: w1668 -> [w1671 _]
              frame False {
                n650 = Strip Path(path=w1671) -> (stripped path=w1675:path)  [unwired: 1 out]
                n651 = Delete(path (use dialog)=w1675, entire hierarchy (F)=TRUE, error in=w1673) -> (error out=w1672:errorcluster)  [unwired: 2 in, 2 out]
              }
              frame True {
              }
            }
          }
          frame True {
            n652 = case shown="False" FALSE {
              tunnel: w1681 -> [w1691 w1696]
              tunnel: w1680 -> [w1692 w1695]
              tunnel: [w1688 w1694] -> w1682
              tunnel: w1678 -> [w1684 _]
              tunnel: w1677 -> [w1683 _]
              frame False {
                n653 = Strip Path(path=w1691) -> (stripped path=w1690:path)  [unwired: 1 out]
                n654 = call "TreeMenuUpdatePath.vi"("error in"=w1692, "Level"=2, "ProcessDataTreeMenu"=w1684, "stripped path"=w1690) -> ("error out"=w1689:errorcluster, "stripped path out"=w1687:path)  [unwired: 1 in]
                n655 = call "TreeMenuUpdatePath.vi"("error in"=w1689, "Level"=1, "ProcessDataTreeMenu"=w1683, "stripped path"=w1687) -> ("error out"=w1688:errorcluster)  [unwired: 1 in, 1 out]
              }
              frame True {
                n656 = disable-structure shown="Disabled" {
                  disable-tunnel: w1696 -> [w1701 _]
                  disable-tunnel: w1695 -> [w1700 _]
                  disable-tunnel: [w1699 _] -> w1694
                  frame Disabled {
                    n657 = Strip Path(path=w1701) -> (stripped path=w1698:path)  [unwired: 1 out]
                    n658 = Delete(path (use dialog)=w1698, entire hierarchy (F)=TRUE, error in=w1700) -> (error out=w1699:errorcluster)  [unwired: 2 in, 2 out]
                  }
                  frame Enabled {
                  }
                }
                n659 = One Button Dialog(message="Yes") -> ()  [unwired: 1 in, 1 out]
              }
            }
          }
        }
      }
      frame "ProcessRecent" {
        n660 = Unbundle By Name(w1704) -> ("Data Acquisition.RecordPath"=w1707:path, "cRef.Data.References.Menu"=w1702:refnum<vi>)
        n661 = Empty String/Path?(string/path=w1707) -> (empty?=w1708:bool)
        n662 = case shown="False" w1708 {
          tunnel: w1707 -> [w1722 _]
          tunnel: w1706 -> [w1711 w1723]
          tunnel: [w1709 w1723] -> w1705
          tunnel: w1704 -> [w1719 w1724]
          tunnel: [w1717 w1724] -> w1703
          tunnel: w1702 -> [w1710 _]
          frame False {
            n663 = Strip Path(path=w1722) -> (stripped path=w1713:path)  [unwired: 1 out]
            n664 = Strip Path(path=w1713) -> (stripped path=w1721:path)  [unwired: 1 out]
            n665 = Path To String(path=w1721) -> (string=w1714:string)
            n666 = invoke class="Tree (strict)" method="Open/Close.Item"(reference=w1710, error in=w1711, "tag"=w1714, "Open"=TRUE ("Open?")) -> (reference out=w1716:refnum<vi>, error out=w1715:errorcluster)  [unwired: 1 in, 3 out]
            n667 = Path To String(path=w1713) -> (string=w1718:string)
            n668 = Path To String(path=w1713) -> (string=w1712:string)
            n669 = property class="Tree (strict)"(reference=w1716, error in=w1715, "Value"=w1712) -> (error out=w1709:errorcluster)  [unwired: 1 out]
            n670 = Bundle By Name(cluster=w1719, "Data Process.ActiveItemTag"=w1718) -> (w1717:T3)
          }
          frame True {
          }
        }
      }
      frame "Stop Reference" {
        n671 = Unbundle By Name(w1739) -> ("Reference signal.Queue"=w1735:refnum<queue>, "Data Acquisition.Control?"=w1726:bool, "Acquisition.Queue"=w1727:refnum<queue>)
        n672 = Enqueue Element(queue=w1727, element=cluster{"Msg":string, "Data":variant} {"Msg"="Halt DAQ", "Data"=variant}, error in (no error)=w1732) -> (error out=w1736:errorcluster)  [unwired: 1 in, 2 out]
        n673 = case shown="False" w1726 {
          tunnel: w1736 -> [w1743 w1744]
          tunnel: w1735 -> [w1742 _]
          tunnel: [w1740 w1744] -> w1731
          frame False {
            n674 = Enqueue Element(queue=w1742, element="Stop" ("DataAcqState"), error in (no error)=w1743) -> (error out=w1740:errorcluster)  [unwired: 1 in, 2 out]
          }
          frame True {
          }
        }
        n675 = call "AE Variables.vi"("VariantIn"=FALSE, "error in (no error)"=w1731, "Action"=Enum_Variables."Set DAQ Connected") -> ("error out"=w1730:errorcluster)  [unwired: 9 in, 7 out]
        n676 = call-poly <userlib>:"Filter Error Codes__ogtk.vi"("Error In"=w1730, "Error Codes to Filter"=i32[] [1, 1000]) -> ("Error Out"=w1733:errorcluster)  [unwired: 7 in, 2 out]
        n677 = Bundle By Name(cluster=w1739, "Reference signal.Monitor"=FALSE) -> (w1738:T3)
      }
      frame "Calibrate Pressure: Step 1" {
        # "Dont detect paper movement"
        # "Temporary file location"
        n678 = global read "DataPathGlobalVariable.vi" "DataPath"() -> (w1750:path)
        n679 = global write "DataAcqRecordPathGlobal.vi" "PressureCalibrationFactor"(1.0 ("PressureCalibrationFactor")) -> ()
        n680 = Build Path(base path=w1750, name or relative path="calibration.tdms") -> (appended path=w1748:path)
        n681 = global write "DataAcqRecordPathGlobal.vi" "DataAcqRecordPath"(w1748) -> ()
        n682 = Bundle By Name(cluster=w1745, "Reference signal.Monitor"=FALSE) -> (w1752:T3)
      }
      frame "Calibrate Pressure: Step 2" {
        w1757 = cluster{"Msg":string, "Data":variant} {"Msg"="", "Data"=variant} ("element")
        # "Start acquisition"
        n683 = Unbundle By Name(w1762) -> ("Acquisition.Queue"=w1761:refnum<queue>, "Data Acquisition.Control?"=w1753:bool)
        n684 = Bundle By Name(cluster=w1757, "Msg"="Acquire") -> (w1758:cluster{"Msg":string, "Data":variant})
        n685 = Enqueue Element(queue=w1761, element=w1758, error in (no error)=w1754) -> (queue out=w1760:refnum<queue>, error out=w1756:errorcluster)  [unwired: 1 in, 1 out]
        n686 = case shown="True" w1753 {
          tunnel: w1760 -> [_ w1769]
          tunnel: w1757 -> [_ w1768]
          tunnel: w1756 -> [w1763 w1765]
          tunnel: [w1763 w1764] -> w1755
          frame False {
          }
          frame True {
            n687 = Bundle By Name(cluster=w1768, "Msg"="Control: Deflate") -> (w1767:cluster{"Msg":string, "Data":variant})
            n688 = Enqueue Element(queue=w1769, element=w1767, error in (no error)=w1765) -> (error out=w1764:errorcluster)  [unwired: 1 in, 2 out]
          }
        }
      }
      frame "Calibrate Pressure: Step 3" {
        w1792 = 5 items=["No error", "Argument error", "Memory is full", "Out of zone", "End of file", "File already open", "Generic file I/O error", "File not found", "File permission error", "Disk is full", "Duplicate path", "Too many files open", "System feature not enabled", "Resource file not found", "Cannot add resource", "Resource not found", "Image not found", "Image memory error", "Pen does not exist", "Config type invalid", "Config token not found", "Config parse error", "Config memory error", "Bad external code format", "Bad external code offset", "External code not present", "Null window", "Destroy window error", "Null menu", "Print aborted", "Bad print record", "Print driver error", "Windows error during printing", "Memory error during printing", "Print dialog error", "Generic print error", "Invalid device refnum", "Device not found", "Device parameter error", "Device unit error", "Cannot open device", "Device call aborted", "Generic error", "Cancelled by user", "Object ID too low", "Object ID too high", "Object not in heap", "Unknown heap", "Unknown object (invalid DefProc)", "Unknown object (DefProc not in table)", "Message out of range", "Invalid (null) method", "Unknown message", "Manager call not supported", "Bad address", "Network operation in progress", "Network operation timed out", "Connection is busy", "Network attribute not supported", "Network error", "Address in use", "System out of memory", "Connection aborted", "Connection refused", "Not connected", "Already connected", "Connection closed", "Initialization error (interapplication manager)", "Bad occurrence", "Wait on unbound occurrence handler", "Occurrence queue overflow", "Datalog type conflict", "Unused", "Unrecognized type (interapplication manager)", "Memory corrupt", "Failed to make temporary DLL", "Old CIN version", "Drag socket not found", "Failed to load drop-object", "Failed to register OLE object", "Failed to release OLE object", "Format specifier type mismatch", "Unknown format specifier", "Too few format specifiers", "Too many format specifiers", "Scan failed", "Newer CIN version", "OLE Convert", "Runtime menu error", "Password tampered", "Unknown error code"] ("Error Code")
        # "Calculate calibration factor from measurement"
        n689 = global read "DataAcqRecordPathGlobal.vi" "DataAcqRecordPath"() -> (w1796:path)
        n690 = Unbundle By Name(w1779) -> ("Data Acquisition.Control?"=w1771:bool, "Acquisition.Queue"=w1778:refnum<queue>)
        n691 = call "AutomaticCalibration.vi"("error in (no error)"=w1777, "Path"=w1796) -> ("error out"=w1794:errorcluster, "Path Out"=w1795:path)  [unwired: 8 in]
        n692 = Delete(path (use dialog)=w1795, error in=w1794) -> (deleted path=w1785:path, error out=w1793:errorcluster)  [unwired: 3 in, 1 out]
        n693 = call-poly <userlib>:"MGI Suppress Error Code.vi"("Error Code"=w1792, "Error In"=w1793) -> ("Error Supressed?"=w1786:bool, "Error Out"=w1783:errorcluster)  [unwired: 4 in]
        n694 = case shown="True" w1786 {
          tunnel: w1785 -> [w1805 w1808]
          tunnel: [w1805 w1806] -> w1784
          tunnel: w1783 -> [w1804 w1811]
          tunnel: [w1804 w1809] -> w1782
          frame False {
          }
          frame True {
            n695 = flat-sequence {
              tunnel: w1811 -> [w1813]
              tunnel: [w1813] -> w1810
              tunnel: w1808 -> [w1812]
              tunnel: [w1812] -> w1807
              tunnel: w1810 -> [w1818]
              tunnel: [w1817] -> w1809
              tunnel: w1807 -> [w1816]
              tunnel: [w1815] -> w1806
              frame #0 {
                n696 = Wait (ms)(milliseconds to wait=u32 1000) -> ()  [unwired: 1 out]
              }
              frame #1 {
                n697 = Delete(path (use dialog)=w1816, error in=w1818) -> (deleted path=w1815:path, error out=w1817:errorcluster)  [unwired: 3 in, 1 out]
              }
            }
          }
        }
        n698 = Enqueue Element(queue=w1778, element=cluster{"Msg":string, "Data":variant} {"Msg"="Idle", "Data"=variant}, error in (no error)=w1777) -> (queue out=w1770:refnum<queue>, error out=w1773:errorcluster)  [unwired: 1 in, 1 out]
        n699 = case shown="True" w1771 {
          tunnel: w1773 -> [w1799 w1802]
          tunnel: [w1799 w1801] -> w1772
          tunnel: w1770 -> [_ w1800]
          frame False {
          }
          frame True {
            n700 = Enqueue Element(queue=w1800, element=cluster{"Msg":string, "Data":variant} {"Msg"="Control: Halt Deflate", "Data"=variant}, error in (no error)=w1802) -> (error out=w1801:errorcluster)  [unwired: 1 in, 2 out]
          }
        }
        n701 = Strip Path(path=w1784) -> (stripped path=w1787:path, name=w1790:string)
        n702 = Concatenate Strings(w1790, "_index" ("name or relative path")) -> (w1788:string)
        n703 = Bundle By Name(cluster=w1779, "Reference signal.Monitor"=TRUE) -> (w1798:T3)
        n704 = Build Path(base path=w1787, name or relative path=w1788) -> (appended path=w1791:path)
        n705 = Delete(path (use dialog)=w1791, error in=w1782) -> (error out=w1781:errorcluster)  [unwired: 3 in, 2 out]
        n706 = call-poly <userlib>:"MGI Suppress Error Code.vi"("Error Code"=1430, "Error In"=w1781) -> ("Error Out"=w1775:errorcluster)  [unwired: 4 in, 1 out]
        n707 = Merge Errors(w1775, w1772) -> (w1776:errorcluster)
      }
      frame "Check Data Folder" {
        n708 = global read "DataPathGlobalVariable.vi" "DataPath"() -> (w1820:path)
        n709 = call <vilib>:"Check if File or Folder Exists.vi"("error in (no error)"=w1822, "path"=w1820) -> ("error out"=w1819:errorcluster, "file or folder exists?"=w1824:bool)  [unwired: 7 in, 1 out]
        n710 = case shown="False" w1824 {
          tunnel: w1823 -> [_ _]
          tunnel: w1819 -> [w1826 w1829]
          tunnel: [w1826 w1829] -> w1821
          frame False {
            n711 = One Button Dialog(message="The Data folder has not been found. Please replace the Data folder in the application directory or start data acquisition to generate a new one. ", button name ("OK")="Close") -> ()  [unwired: 1 out]
          }
          frame True {
          }
        }
      }
      frame "ChangeTab" {
      }
      frame "/***Data Processing***/" {
      }
      frame "GetActiveItemTag" {
        n712 = Bundle By Name(cluster=w1836, "Data Process.ActiveItemTag"=w1834) -> (w1835:T3)
      }
      frame "FilterControl" {
        n713 = Unbundle By Name(w1842) -> ("cRef.Data.References.FilterControl"=w1841:refnum<vi>)
        n714 = property class="Bool (strict)"(reference=w1841, error in=w1839) -> (error out=w1838:errorcluster, "Value"=w1840:bool)  [unwired: 1 out]
        n715 = call "AE Variables.vi"("VariantIn"=w1840, "error in (no error)"=w1838, "Action"=Enum_Variables."Set Filter") -> ("error out"=w1843:errorcluster)  [unwired: 9 in, 7 out]
      }
      frame "Display Data" {
        # "Open measurement and display graph"
        n716 = Unbundle By Name(w1851) -> ("Data Process.ActiveItemTag"=w1852:string, "Data.Queue"=w1845:refnum<queue>)
        n717 = String To Path(string=w1852) -> (path=w1853:path)
        n718 = Build Path(base path=w1853, name or relative path="Data.tdms") -> (appended path=w1849:path)
        n719 = call-poly <userlib>:"File Exists__ogtk.vi"("file path"=w1849) -> ("exists"=w1850:bool)  [unwired: 6 in, 1 out]
        n720 = case shown="True" w1850 {
          tunnel: w1848 -> [w1857 w1868]
          tunnel: w1849 -> [_ w1865]
          tunnel: [w1857 w1866] -> w1846
          tunnel: w1851 -> [w1856 w1864]
          tunnel: [w1856 w1858] -> w1847
          tunnel: w1845 -> [_ w1860]
          frame False {
          }
          frame True {
            # "Send command to data processing vi"
            n721 = call "AE DataProcessControl.vi"("Action"=Enum_Process_Data."Set Data Path", "error in (no error)"=w1868, "Data Path In"=w1865) -> ("error out"=w1862:errorcluster)  [unwired: 6 in, 2 out]
            n722 = call "GetHeightAdj.vi"("appended path"=w1865) -> ("Numeric"=w1863:dbl)
            n723 = Enqueue Element(queue=w1860, element=cluster{"Msg":string, "Data":variant} {"Msg"="Update", "Data"=variant}, error in (no error)=w1862) -> (error out=w1861:errorcluster)  [unwired: 1 in, 2 out]
            n724 = Bundle By Name(cluster=w1864, "Database.Height Adjustment"=w1863) -> (w1858:T3)
            n725 = call "AE Variables.vi"("error in (no error)"=w1861, "Action"=Enum_Variables."Reset Pressure") -> ("error out"=w1866:errorcluster)  [unwired: 10 in, 7 out]
          }
        }
        n726 = Bundle By Name(cluster=w1847, "Database.PatientdataPath"=w1853) -> (w1855:T3)
      }
      frame "Flow: View Signals" {
        n727 = Unbundle By Name(w1875) -> ("Data Process.ActiveItemTag"=w1874:string)
        n728 = String To Path(string=w1874) -> (path=w1873:path)
        n729 = Build Path(base path=w1873, name or relative path="Data.tdms") -> (appended path=w1871:path)
        n730 = call-poly <userlib>:"File Exists__ogtk.vi"("file path"=w1871) -> ("exists"=w1870:bool)  [unwired: 6 in, 1 out]
        n731 = case shown="True" w1870 {
          tunnel: w1871 -> [_ w1877]
          frame False {
          }
          frame True {
            n732 = call "FlowPopup.vi"("Path"=w1877) -> ()  [unwired: 11 in]
          }
        }
      }
      frame "Set Tangent Mode" {
        n733 = Unbundle By Name(w1882) -> ("Data.Queue"=w1881:refnum<queue>, "cRef.Data.References.Tangent On/Off"=w1879:refnum<vi>)
        n734 = property class="Bool (strict)"(reference=w1879) -> ("Value"=w1878:bool)  [unwired: 1 in, 2 out]
        n735 = call "AE DataProcessControl.vi"("Action"=Enum_Process_Data."Set Cursor Mode", "error in (no error)"=w1885, "Cursor Mode In"=w1878) -> ("error out"=w1884:errorcluster)  [unwired: 6 in, 2 out]
        n736 = Enqueue Element(queue=w1881, element=cluster{"Msg":string, "Data":variant} {"Msg"="Set Tangent Mode", "Data"=variant}, error in (no error)=w1884) -> (error out=w1883:errorcluster)  [unwired: 1 in, 2 out]
      }
      frame "Set Tangent Mode: True" {
        w1887 = TRUE ("Value")
        n737 = Unbundle By Name(w1891) -> ("Data.Queue"=w1890:refnum<queue>, "cRef.Data.References.Tangent On/Off"=w1888:refnum<vi>)
        n738 = property class="Bool (strict)"(reference=w1888, "Value"=w1887) -> ()  [unwired: 1 in, 2 out]
        n739 = call "AE DataProcessControl.vi"("Action"=Enum_Process_Data."Set Cursor Mode", "error in (no error)"=w1894, "Cursor Mode In"=w1887) -> ("error out"=w1893:errorcluster)  [unwired: 6 in, 2 out]
        n740 = Enqueue Element(queue=w1890, element=cluster{"Msg":string, "Data":variant} {"Msg"="Set Tangent Mode", "Data"=variant}, error in (no error)=w1893) -> (error out=w1892:errorcluster)  [unwired: 1 in, 2 out]
      }
      frame "Reset Graphs" {
        n741 = Unbundle By Name(w1900) -> ("Data.Queue"=w1899:refnum<queue>, "cRef.Data.References.Tangent On/Off"=w1897:refnum<vi>)
        n742 = property class="Bool (strict)"(reference=w1897) -> ("Value"=w1896:bool)  [unwired: 1 in, 2 out]
        n743 = call "AE DataProcessControl.vi"("Action"=Enum_Process_Data."Set Cursor Mode", "error in (no error)"=w1903, "Cursor Mode In"=w1896) -> ("error out"=w1902:errorcluster)  [unwired: 6 in, 2 out]
        n744 = Enqueue Element(queue=w1899, element=cluster{"Msg":string, "Data":variant} {"Msg"="Reset", "Data"=variant}, error in (no error)=w1902) -> (error out=w1901:errorcluster)  [unwired: 1 in, 2 out]
      }
      frame "ExportGraphs" {
        w1908 = "\r"
        n745 = Unbundle By Name(w1922) -> ("User Parameters.CPR Number"=w1909:string, "User Parameters.Name"=w1910:string, "User Parameters.Operator"=w1921:string, "User Parameters.Measuring Type"=w1907:string)
        n746 = String To Path(string=w1917) -> (path=w1919:path)
        n747 = Path to Array of Strings(0:w1919) -> (2:w1912:string[])  [unwired: 1 out]
        n748 = Reverse 1D Array(array=w1912) -> (reversed array=w1915:string[])
        n749 = while {
          tunnel: w1915 -> [w1934] mode=indexing
          tunnel: "[0-9]{4}-[0-9]{2}-[0-9]{2}" ("regular expression") -> [w1932]
          tunnel: [w1930] -> w1916
          i -> [w1930]
          stop <- w1931 stop-if-true
          n750 = xnode "Match Regular Expression"("input string"=w1934, "regular expression"=w1932) -> ("offset past match"=w1933:i32)  [unwired: 4 in, 4 out]
          n751 = Greater Or Equal To 0?(x=w1933) -> (x >= 0?=w1931:bool)
        }
        n752 = Concatenate Strings(w1909, w1908, w1910, w1908, w1921) -> (w1920:string)
        n753 = Delete From Array(array=w1912, length=w1916) -> (array with subset deleted=w1911:string[])  [unwired: 1 in, 1 out]
        n754 = Array of Strings to Path(0:w1911) -> (2:w1914:path)  [unwired: 1 in]
        n755 = Path To String(path=w1914) -> (string=w1913:string)
        n756 = call "exportGraphsToPDF.vi"("PatientID"=w1909, "error in (no error)"=w1923, "Type"=w1907, "Text"=w1920, "Folder"=w1913) -> ("error out"=w1906:errorcluster)  [unwired: 6 in]
        n757 = case shown="Error" w1906 {
          selector: w1906 -> [w1924 w1928]
          tunnel: [w1924 errorcluster {"status"=FALSE, "code"=0, "source"=""} ("error IO")] -> w1905
          frame No Error {
          }
          frame Error {
            n758 = Unbundle By Name(w1928) -> ("source"=w1927:string)
            n759 = Concatenate Strings("An error occured when trying to export the graph:  " ("message"), w1927) -> (w1925:string)
            n760 = One Button Dialog(message=w1925) -> ()  [unwired: 1 in, 1 out]
          }
        }
      }
      frame "ChangeSegment" {
        n761 = Unbundle By Name(w2047) -> ("cRef.Configuration.References.ListboxMeasurementArea"=w2046:refnum<vi>)
        n762 = call "ChangeSegment.vi"("error in (no error)"=w2053, "Message Value"=w2048, "cRef.Configuration.References.ListboxMeasurementArea"=w2046) -> ("error out"=w2051:errorcluster, "Moved?"=w2052:bool, "target out"=w2049:path)  [unwired: 6 in]
        n763 = case shown="True" w2052 {
          tunnel: w2051 -> [w2054 w2074]
          tunnel: [w2054 w2058] -> w2050
          tunnel: w2049 -> [_ w2070]
          tunnel: w2048 -> [_ w2067]
          tunnel: w2047 -> [_ w2064]
          frame False {
          }
          frame True {
            n764 = Unbundle By Name(w2064) -> ("User Parameters.CPR Number"=w2063:string, "cRef.Data.References.Menu"=w2056:refnum<vi>, "cRef.Journal.References.Menu"=w2055:refnum<vi>)
            n765 = invoke class="Tree (strict)" method="Edit Tree Items.Delete"(reference=w2056, error in=w2074, "tag"=w2067, "Delete Children"=TRUE ("Delete Children?")) -> (reference out=w2068:refnum<vi>, error out=w2071:errorcluster)  [unwired: 1 in, 3 out]
            n766 = global read "DataPathGlobalVariable.vi" "DataPath"() -> (w2061:path)
            n767 = call "Encrypt.vi"("Input"=w2063) -> ("Output"=w2062:string)  [unwired: 10 in]
            n768 = call "TreeMenuUpdatePath.vi"("error in"=w2071, "Level"=2, "ProcessDataTreeMenu"=w2068, "stripped path"=w2070) -> ("error out"=w2066:errorcluster, "stripped path out"=w2065:path)  [unwired: 1 in]
            n769 = Build Path(base path=w2061, name or relative path=w2062) -> (appended path=w2060:path)
            n770 = Path To String(path=w2065) -> (string=w2072:string)
            n771 = property class="Tree (strict)"(reference=w2068, error in=w2066, "Value"=w2072) -> (error out=w2057:errorcluster)  [unwired: 1 out]
            n772 = call "Init_Open_Close.vi"("error in"=w2057, "Level"=1, "path to start the search"=w2060, "Tree In"=w2055) -> ("error out"=w2058:errorcluster)  [unwired: 5 in, 2 out]
          }
        }
      }
      frame "DeleteTreeItem" {
        n773 = Two Button Dialog(message="Are you sure you want to delete this data permanently?", 2:"Yes" ("T button name (\"OK\")")) -> (T button?=w2079:bool)  [unwired: 1 in]
        n774 = case shown="True" w2079 {
          tunnel: w2080 -> [_ w2093]
          tunnel: w2078 -> [w2082 w2087]
          tunnel: [w2082 w2092] -> w2081
          tunnel: w2080 -> [_ w2086]
          tunnel: w2075 -> [_ w2085]
          frame False {
          }
          frame True {
            n775 = Unbundle By Name(w2085) -> ("cRef.Data.References.Menu"=w2084:refnum<vi>, "cRef.Journal.References.Menu"=w2083:refnum<vi>)
            n776 = String To Path(string=w2086) -> (path=w2089:path)
            n777 = Delete(path (use dialog)=w2089, entire hierarchy (F)=TRUE, confirm (F)=FALSE, error in=w2087) -> (error out=w2088:errorcluster)  [unwired: 1 in, 2 out]
            n778 = Build Array(w2084, w2083) -> (w2094:refnum<vi>[])
            n779 = for {
              tunnel: w2094 -> [w2097] mode=indexing
              tunnel: w2093 -> [w2100]
              tunnel: w2088 -> [w2098]
              tunnel: [w2095] -> w2092
              n780 = invoke class="Tree (strict)" method="Edit Tree Items.Delete"(reference=w2097, error in=w2098, "tag"=w2100, "Delete Children"=TRUE ("Delete Children?")) -> (error out=w2096:errorcluster)  [unwired: 1 in, 4 out]
              n781 = call <userlib>:"Clear All Errors__ogtk.vi"("Error In"=w2096) -> ("Error Out"=w2095:errorcluster)  [unwired: 3 in]
            }
          }
        }
      }
      frame "/***Journal***/" {
      }
      frame "FillDataTable" {
        n782 = Unbundle By Name(w2111) -> ("cRef.Journal.References.Data"=w2103:refnum<vi>, "Database.ActiveItemTag"=w2109:string)
        n783 = Empty String/Path?(string/path=w2108) -> (empty?=w2107:bool)
        n784 = Select(t=w2109, s=w2107, f=w2108) -> (s? t:f=w2110:string)
        n785 = String To Path(string=w2110) -> (path=w2105:path)
        n786 = call-poly <userlib>:"File Exists__ogtk.vi"("file path"=w2105) -> ("exists"=w2106:bool)  [unwired: 6 in, 1 out]
        n787 = case shown="True" w2106 {
          tunnel: [w2114 w2118] -> w2112
          tunnel: w2104 -> [w2114 w2117]
          tunnel: w2105 -> [_ w2116]
          tunnel: w2103 -> [_ w2115]
          frame False {
          }
          frame True {
            n788 = case shown="No Error" w2117 {
              selector: w2117 -> [w2120 w2123]
              tunnel: [w2122 w2124] -> w2118
              tunnel: w2116 -> [w2121 _]
              tunnel: w2115 -> [w2119 _]
              frame No Error {
                n789 = call "ListboxItems (SubVI).vi"("error in (no error)"=w2120, "MCListbox Refnum"=w2119, "path"=w2121) -> ("error out"=w2122:errorcluster)  [unwired: 2 in]
              }
              frame Error {
                n790 = call-poly <userlib>:"MGI Suppress Error Code.vi"("Error Code"=1430, "Error In"=w2123) -> ("Error Out"=w2124:errorcluster)  [unwired: 4 in, 1 out]
              }
            }
          }
        }
        n791 = Bundle By Name(cluster=w2111, "Database.ActiveItemTag"=w2110) -> (w2113:T3)
      }
      frame "GenerateReport" {
        n792 = Unbundle By Name(w2134) -> ("Database.ActiveItemTag"=w2127:string, "cRef.Journal.References.ReportSelection"=w2129:refnum<vi>)
        n793 = case shown="False" FALSE {
          tunnel: [T19."leave excel open after last close" ("closing behavior (leave open)") T19."close excel after last close" ("closing behavior (leave open)")] -> w2135
          frame False {
          }
          frame True {
          }
        }
        n794 = property class="Ring (strict)"(reference=w2129) -> ("Value"=w2128:u16)  [unwired: 1 in, 2 out]
        n795 = Empty String/Path?(string/path=w2127) -> (empty?=w2126:bool)
        n796 = case shown="False" w2126 {
          tunnel: w2136 -> [w2142 w2144]
          tunnel: w2135 -> [w2141 _]
          tunnel: [w2140 path "" ("ReportPath")] -> w2132
          tunnel: [w2139 w2144] -> w2131
          tunnel: w2128 -> [w2138 _]
          tunnel: w2127 -> [w2137 _]
          frame False {
            n797 = call "GetDataForExcel.vi"("error in (no error)"=w2142, "ID"=w2137, "ReportSelection"=w2138, "closing behavior (leave open)"=w2141) -> ("error out"=w2139:errorcluster, "ReportPath"=w2140:path)  [unwired: 5 in, 1 out]
          }
          frame True {
          }
        }
        n798 = Bundle By Name(cluster=w2134, "Database.JournalPath"=w2132) -> (w2133:T3)
      }
      frame "DeleteSingleMeasurement" {
        n799 = Unflatten From String(type=cluster{i32, i32} {0, 0}, binary string=w2167, error in (no error)=w2152) -> (value=w2165:cluster{i32, i32}, error out=w2154:errorcluster)  [unwired: 2 in, 1 out]
        n800 = Unbundle By Name(w2164) -> ("Database.ActiveItemTag"=w2150:string, "cRef.Journal.References.Data"=w2147:refnum<vi>)
        n801 = Unbundle(w2165) -> (w2163:i32, w2156:i32)
        n802 = String To Path(string=w2150) -> (path=w2148:path)
        n803 = List Folder(path=w2148, error in=w2154) -> (folder names=w2162:string[], error out=w2153:errorcluster)  [unwired: 2 in, 2 out]
        n804 = Index Array(array=w2162, index=w2163) -> (element=w2161:string)
        n805 = Build Path(base path=w2148, name or relative path=w2161) -> (appended path=w2160:path)
        n806 = Build Path(base path=w2160, name or relative path="processdata.dm2000") -> (appended path=w2158:path)
        n807 = call <vilib>:"Check if File or Folder Exists.vi"("error in (no error)"=w2153, "path"=w2158) -> ("error out"=w2151:errorcluster, "file or folder exists?"=w2157:bool, "dup path"=w2155:path)  [unwired: 7 in]
        n808 = case shown="True" w2157 {
          tunnel: w2156 -> [_ w2177]
          tunnel: w2155 -> [_ w2175]
          tunnel: w2151 -> [w2168 w2173]
          tunnel: [w2168 w2172] -> w2149
          tunnel: w2148 -> [_ w2171]
          tunnel: w2147 -> [_ w2169]
          frame False {
          }
          frame True {
            n809 = call-poly <vilib>:"Read From Spreadsheet File.vi"("delimiter (\\t)"=";" ("delimiter (\\t)"), "file path (dialog if empty)"=w2175) -> ("first row"=w2174:dbl[])  [unwired: 5 in, 4 out]
            n810 = case shown="1" w2177 {
              tunnel: w2175 -> [_ w2186 w2194]
              tunnel: w2174 -> [_ w2185 w2193]
              tunnel: w2171 -> [w2178 w2179 w2187]
              tunnel: [w2178 w2179 w2187] -> w2170
              frame 0, Default {
              }
              frame 1 {
                n811 = Replace Array Subset(array=w2185, new element=0.0 ("new element/subarray"), index=0) -> (w2182:dbl[])
                n812 = call-poly <vilib>:"Write To Spreadsheet File.vi"("delimiter (\\t)"=";" ("delimiter (\\t)"), "append to file? (new file:F)"=FALSE, "1D data"=w2182, "file path (dialog if empty)"=w2186) -> ()  [unwired: 4 in, 1 out]
              }
              frame 2 {
                n813 = Replace Array Subset(array=w2193, new element=0.0 ("new element/subarray"), index=1) -> (w2190:dbl[])
                n814 = call-poly <vilib>:"Write To Spreadsheet File.vi"("delimiter (\\t)"=";" ("delimiter (\\t)"), "append to file? (new file:F)"=FALSE, "1D data"=w2190, "file path (dialog if empty)"=w2194) -> ()  [unwired: 4 in, 1 out]
              }
            }
            n815 = call "ListboxItems (SubVI).vi"("error in (no error)"=w2173, "MCListbox Refnum"=w2169, "path"=w2170) -> ("error out"=w2172:errorcluster)  [unwired: 2 in]
          }
        }
      }
      frame "/****Save Data****/" {
      }
      frame "SaveArmPressure" {
        w2201 = 0 ("index (row)")
        w2207 = 0 ("index (row)")
        n816 = Unbundle By Name(w2224) -> ("User Parameters.CPR Number"=w2219:string, "System Parameters.Date"=w2222:string, "User Parameters.RightArm"=w2212:string[][], "User Parameters.LeftArm"=w2211:string[][], "User Parameters.Puls"=w2197:dbl)
        n817 = call "Encrypt.vi"("Input"=w2219) -> ("Output"=w2218:string)  [unwired: 10 in]
        n818 = global read "DataPathGlobalVariable.vi" "DataPath"() -> (w2220:path)
        n819 = Initialize Array(0, 2 ("dimension size"), 4) -> (w2203:i32[][])
        n820 = Decimal String To Number(string=w2212) -> (number=w2210:i32[][])  [unwired: 2 in, 1 out]
        n821 = Decimal String To Number(string=w2211) -> (number=w2209:i32[][])  [unwired: 2 in, 1 out]
        n822 = Transpose 2D Array(2D array=w2210) -> (transposed array=w2204:i32[][])
        n823 = Build Path(base path=w2220, name or relative path=w2218) -> (appended path=w2223:path)
        n824 = Transpose 2D Array(2D array=w2209) -> (transposed array=w2202:i32[][])
        n825 = Build Path(base path=w2223, name or relative path=w2222) -> (appended path=w2221:path)
        n826 = Replace Array Subset(array=w2203, new element=w2204, index (row)=w2207, index (col)=w2207) -> (w2200:i32[][])
        n827 = Replace Array Subset(array=w2203, new element=w2202, index (row)=w2201, index (col)=w2201) -> (w2199:i32[][])
        n828 = call <userlib>:"Create Dir if Non-Existant__ogtk.vi"("error in (no error)"=w2217, "Directory Path"=w2221) -> ("error out"=w2213:errorcluster, "dup Directory Path"=w2215:path)  [unwired: 7 in, 1 out]
        n829 = Build Array (concatenate)(w2200, w2199) -> (w2198:i32[][])
        n830 = Not A Number/Path/Refnum?(number/path/refnum=w2215) -> (NaN/Path/Refnum?=w2214:bool)
        n831 = case shown="No Error" w2213 {
          selector: w2213 -> [w2227 w2246]
          tunnel: w2215 -> [w2230 _]
          tunnel: [w2229 w2246] -> w2216
          tunnel: w2214 -> [w2228 _]
          tunnel: w2198 -> [w2226 _]
          tunnel: w2197 -> [w2225 _]
          frame No Error {
            n832 = case shown="False" w2228 {
              tunnel: [w2236 w2245] -> w2229
              tunnel: w2230 -> [w2237 _]
              tunnel: w2227 -> [w2236 w2244]
              tunnel: w2226 -> [w2235 _]
              tunnel: w2225 -> [w2233 _]
              frame False {
                n833 = Build Path(base path=w2237, name or relative path="armpressure.dm2000") -> (appended path=w2231:path)
                n834 = Build Array(w2233) -> (w2232:dbl[])
                n835 = Build Array (concatenate)(w2235, w2232) -> (w2234:dbl[][])
                n836 = call-poly <vilib>:"Write To Spreadsheet File.vi"("delimiter (\\t)"=";" ("delimiter (\\t)"), "append to file? (new file:F)"=FALSE, "2D data"=w2234, "file path (dialog if empty)"=w2231) -> ()  [unwired: 4 in, 1 out]
              }
              frame True {
                w2242 = 7 items=["No error", "Argument error", "Memory is full", "Out of zone", "End of file", "File already open", "Generic file I/O error", "File not found", "File permission error", "Disk is full", "Duplicate path", "Too many files open", "System feature not enabled", "Resource file not found", "Cannot add resource", "Resource not found", "Image not found", "Image memory error", "Pen does not exist", "Config type invalid", "Config token not found", "Config parse error", "Config memory error", "Bad external code format", "Bad external code offset", "External code not present", "Null window", "Destroy window error", "Null menu", "Print aborted", "Bad print record", "Print driver error", "Windows error during printing", "Memory error during printing", "Print dialog error", "Generic print error", "Invalid device refnum", "Device not found", "Device parameter error", "Device unit error", "Cannot open device", "Device call aborted", "Generic error", "Cancelled by user", "Object ID too low", "Object ID too high", "Object not in heap", "Unknown heap", "Unknown object (invalid DefProc)", "Unknown object (DefProc not in table)", "Message out of range", "Invalid (null) method", "Unknown message", "Manager call not supported", "Bad address", "Network operation in progress", "Network operation timed out", "Connection is busy", "Network attribute not supported", "Network error", "Address in use", "System out of memory", "Connection aborted", "Connection refused", "Not connected", "Already connected", "Connection closed", "Initialization error (interapplication manager)", "Bad occurrence", "Wait on unbound occurrence handler", "Occurrence queue overflow", "Datalog type conflict", "Unused", "Unrecognized type (interapplication manager)", "Memory corrupt", "Failed to make temporary DLL", "Old CIN version", "Drag socket not found", "Failed to load drop-object", "Failed to register OLE object", "Failed to release OLE object", "Format specifier type mismatch", "Unknown format specifier", "Too few format specifiers", "Too many format specifiers", "Scan failed", "Newer CIN version", "Error converting to variant", "Runtime menu error", "Password tampered", "Variant attribute not found", "Incompatible variant data type", "Event data is not available", "Event Store is not present", "Occurrence is not found", "Event Queue is not created", "Event info is not available", "Refnum passed is NULL", "Error retrieving Class GUID", "Error retrieving CoClass GUID", "Error retrieving TypeLib GUID.", "Bad built application magic bytes.", "Specific driver is different from the specific driver associated with the Logical Name.", "There is no session opened to the class driver.", "Max Error", "MAX - Error with config objects", "MAX - Error loading configuration", "MAX - Group not supported"]
                n837 = call <userlib>:"Build Error Cluster__ogtk.vi"("String to Prepend to source (\"\")"="Armpressure file could not be located or created" ("String to Prepend to source (\"\")"), "code"=w2242) -> ("error out"=w2243:errorcluster)
                n838 = Merge Errors(w2244, w2243) -> (w2245:errorcluster)
              }
            }
          }
          frame Error {
          }
        }
      }
      frame "SaveArmPressure_new" {
        n839 = Unbundle By Name(w2254) -> ("User Parameters.RightArm"=w2253:string[][], "User Parameters.Puls"=w2247:dbl)
        n840 = Decimal String To Number(string=w2253) -> (number=w2252:i32[][])  [unwired: 2 in, 1 out]
        n841 = Transpose 2D Array(2D array=w2252) -> (transposed array=w2248:i32[][])
        n842 = for {
          tunnel: w2251 -> [w2263]
          tunnel: [w2262] -> w2250
          tunnel: T20 {"sys"=0.0, "dia"=0.0, "puls"=0.0, "date"="", "time"="", "code"="", "serial"="", "temp"=0.0, "activity"=""} ("data") -> [w2261]
          tunnel: w2248 -> [w2260] mode=indexing
          tunnel: w2247 -> [w2257]
          n843 = Index Array(array=w2260) -> (element #1=w2259:i32, element #2=w2258:i32)  [unwired: 2 in]
          n844 = Bundle By Name(cluster=w2261, "sys"=w2259, "dia"=w2258, "puls"=w2257) -> (w2256:T20)
          n845 = call "AddArmpressureAndSave.vi"("error in"=w2263, "Side(Left/Right)"="", "data"=w2256) -> ("error out"=w2262:errorcluster)  [unwired: 8 in]
        }
      }
      frame "SavePalpationData" {
        n846 = Unbundle By Name(w2279) -> ("User Parameters.CPR Number"=w2275:string, "System Parameters.Date"=w2277:string, "User Parameters.Temp One"=w2267:dbl, "User Parameters.Temp Two"=w2266:dbl, "User Parameters.PalpationRight"=w2265:string, "User Parameters.PalpationLeft"=w2264:string)
        n847 = global read "DataPathGlobalVariable.vi" "DataPath"() -> (w2276:path)
        n848 = call "Encrypt.vi"("Input"=w2275) -> ("Output"=w2274:string)  [unwired: 10 in]
        n849 = Build Array(w2265, w2264) -> (w2270:string[])
        n850 = Build Array(w2267, w2266) -> (w2268:dbl[])
        n851 = Build Path(base path=w2276, name or relative path=w2274) -> (appended path=w2278:path)
        n852 = Number To Decimal String(number=w2268) -> (decimal integer string=w2269:string[])  [unwired: 1 in]
        n853 = Build Path(base path=w2278, name or relative path=w2277) -> (appended path=w2271:path)
        n854 = case shown="No Error" w2272 {
          selector: w2272 -> [w2289 w2291]
          tunnel: w2271 -> [w2290 _]
          tunnel: [w2289 w2291] -> w2273
          tunnel: w2269 -> [w2280 _]
          tunnel: w2270 -> [w2281 _]
          frame No Error {
            n855 = Build Path(base path=w2290, name or relative path="armpressure.dm2000") -> (appended path=w2286:path)
            n856 = call-poly <vilib>:"Read From Spreadsheet File.vi"("delimiter (\\t)"=";" ("delimiter (\\t)"), "file path (dialog if empty)"=w2286) -> ("all rows"=w2285:string[][])  [unwired: 5 in, 4 out]
            n857 = Build Array (concatenate)(w2285, w2280, w2281) -> (w2284:string[][])
            n858 = call-poly <vilib>:"Write To Spreadsheet File.vi"("delimiter (\\t)"=";" ("delimiter (\\t)"), "append to file? (new file:F)"=FALSE, "2D data"=w2284, "file path (dialog if empty)"=w2286) -> ()  [unwired: 4 in, 1 out]
          }
          frame Error {
          }
        }
      }
      frame "SavePatientData" {
        n859 = Unbundle By Name(w2311) -> ("User Parameters.CPR Number"=w2293:string, "User Parameters.Name"=w2309:string, "User Parameters.Operator"=w2308:string, "User Parameters.Doctor"=w2307:string, "User Parameters.Comment"=w2306:string, "cRef.Profile.References.HospitalName"=w2303:refnum<vi>, "cRef.Profile.References.HospitalDepartment"=w2302:refnum<vi>, "cRef.Profile.References.HospitalAddress"=w2301:refnum<vi>)
        n860 = call "Encrypt.vi"("Input"=w2293) -> ("Output"=w2292:string)  [unwired: 10 in]
        n861 = Bundle By Name(cluster=T22 {"id"="", "name"="", "operator"="", "doctor"="", "comment"=""} ("profile"), "id"=w2292, "name"=w2309, "operator"=w2308, "doctor"=w2307, "comment"=w2306) -> (w2305:T22)
        n862 = call "SavePatientDateInfo_Profile.vi"("error in"=w2296, "profile"=w2305) -> ("error out"=w2295:errorcluster)  [unwired: 9 in]
        n863 = property class="Str"(reference=w2303) -> ("Value"=w2300:string)  [unwired: 1 in, 2 out]
        n864 = property class="Str"(reference=w2302) -> ("Value"=w2299:string)  [unwired: 1 in, 2 out]
        n865 = property class="Str"(reference=w2301) -> ("Value"=w2298:string)  [unwired: 1 in, 2 out]
        n866 = Bundle By Name(cluster=T21 {"name"="", "department"="", "address"=""} ("hospital"), "name"=w2300, "department"=w2299, "address"=w2298) -> (w2297:T21)
        n867 = call "SavePatientDateInfo_Hospital.vi"("error in"=w2295, "hospital"=w2297) -> ("error out"=w2294:errorcluster)  [unwired: 9 in]
      }
      frame "_SavePatientData" {
        n868 = Unbundle By Name(w2333) -> ("User Parameters.CPR Number"=w2315:string, "User Parameters.Name"=w2332:string, "User Parameters.Operator"=w2331:string, "User Parameters.Doctor"=w2330:string, "User Parameters.Comment"=w2329:string, "cRef.Profile.References.HospitalName"=w2312:refnum<vi>, "cRef.Profile.References.HospitalDepartment"=w2313:refnum<vi>, "cRef.Profile.References.HospitalAddress"=w2314:refnum<vi>)
        n869 = global read "DataPathGlobalVariable.vi" "DataPath"() -> (w2328:path)
        n870 = call "Encrypt.vi"("Input"=w2315) -> ("Output"=w2316:string)  [unwired: 10 in]
        n871 = property class="Str"(reference=w2312) -> ("Value"=w2324:string)  [unwired: 1 in, 2 out]
        n872 = property class="Str"(reference=w2313) -> ("Value"=w2323:string)  [unwired: 1 in, 2 out]
        n873 = property class="Str"(reference=w2314) -> ("Value"=w2325:string)  [unwired: 1 in, 2 out]
        n874 = Build Path(base path=w2328, name or relative path=w2316) -> (appended path=w2326:path)
        n875 = Build Array(w2324, w2323) -> (w2322:string[])
        n876 = call <userlib>:"Multi-line String to Array__ogtk.vi"("string"=w2325) -> ("lines"=w2321:string[])
        n877 = Empty String/Path?(string/path=w2315) -> (empty?=w2320:bool)
        n878 = Build Array (concatenate)(w2322, w2321) -> (w2319:string[])
        n879 = Build Array(w2316, w2332, w2331, w2330, w2329) -> (w2327:string[])
        n880 = case shown="False" w2320 {
          tunnel: w2327 -> [w2342 _]
          tunnel: w2326 -> [w2340 _]
          tunnel: w2319 -> [w2335 _]
          tunnel: w2318 -> [w2334 w2343]
          tunnel: [w2334 w2343] -> w2317
          frame False {
            n881 = Build Array(w2342, w2335) -> (w2341:string[][])
            n882 = Build Path(base path=w2340, name or relative path=T18 "index.dm2000" ("FileName")) -> (appended path=w2337:path)
            n883 = call-poly <vilib>:"Write To Spreadsheet File.vi"("delimiter (\\t)"=";" ("delimiter (\\t)"), "append to file? (new file:F)"=FALSE, "2D data"=w2341, "file path (dialog if empty)"=w2337) -> ()  [unwired: 4 in, 1 out]
          }
          frame True {
          }
        }
      }
      frame "SavePatientDataOnDate" {
        n884 = call "AMC Send Local Message.vi"("Message Name"="SavePatientData", "Message Queue in"=w2345) -> ()  [unwired: 8 in, 2 out]
      }
      frame "GetProcessData" {
        n885 = call "AE Variables.vi"("error in (no error)"=w2354, "Action"=Enum_Variables."Get Red Cursors") -> ("Dbl Array"=w2349:dbl[][], "error out"=w2353:errorcluster)  [unwired: 10 in, 6 out]
        n886 = call "AE Variables.vi"("error in (no error)"=w2353, "Action"=Enum_Variables."Get Blue Cursors") -> ("Dbl Array"=w2348:dbl[][], "error out"=w2352:errorcluster)  [unwired: 10 in, 6 out]
        n887 = call "AE Variables.vi"("error in (no error)"=w2352, "Action"=Enum_Variables."Get Red Pressure") -> ("NumericOut"=w2355:dbl, "error out"=w2357:errorcluster)  [unwired: 10 in, 6 out]
        n888 = call "AE Variables.vi"("error in (no error)"=w2357, "Action"=Enum_Variables."Get Blue Pressure") -> ("NumericOut"=w2356:dbl, "error out"=w2362:errorcluster)  [unwired: 10 in, 6 out]
        n889 = Bundle By Name(cluster=w2361, "Database.Blue Pressure"=w2356, "Database.Red Pressure"=w2355, "Database.BluePositionArray"=w2348, "Database.RedPositionArray"=w2349) -> (w2360:T3)
      }
      frame "SaveProcessData" {
        n890 = Unbundle By Name(w2378) -> ("Database.PatientdataPath"=w2374:path, "Database.Blue Pressure"=w2377:dbl, "Database.Red Pressure"=w2376:dbl, "Database.BluePositionArray"=w2367:dbl[][], "Database.RedPositionArray"=w2371:dbl[][])
        n891 = Matrix Size(0:w2367) -> (1:w2370:i32, 2:w2369:i32)
        n892 = Add(x=w2370, y=w2369) -> (x+y=w2364:i32)
        n893 = Less?(x=w2364, y=6 ("x")) -> (x < y?=w2368:bool)
        n894 = Select(t=dbl[][] [[0.0, 0.0], [0.0, 0.0], [0.0, 0.0], [0.0, 0.0]], s=w2368, f=w2367) -> (s? t:f=w2366:dbl[][])
        n895 = Build Array(w2377, w2376) -> (w2373:dbl[])
        n896 = Build Array (concatenate)(w2373, w2366, w2371) -> (w2372:dbl[][])
        n897 = call-poly <userlib>:"Valid Path__ogtk.vi"("path"=w2374) -> ("valid"=w2375:bool)
        n898 = case shown="True" w2375 {
          tunnel: w2372 -> [_ w2380]
          tunnel: w2374 -> [_ w2382]
          frame False {
          }
          frame True {
            n899 = Build Path(base path=w2382, name or relative path=T18 "processdata.dm2000" ("FileName")) -> (appended path=w2383:path)
            n900 = call-poly <vilib>:"Write To Spreadsheet File.vi"("delimiter (\\t)"=";" ("delimiter (\\t)"), "format (%.3f)"="%s" ("format (%s)"), "append to file? (new file:F)"=FALSE, "2D data"=w2380, "file path (dialog if empty)"=w2383) -> ()  [unwired: 3 in, 1 out]
          }
        }
      }
      frame "DeleteMeasurement" {
        n901 = Unbundle By Name(w2401) -> ("cRef.Data.References.Menu"=w2388:refnum<vi>, "cRef.Data.References.Menu"=w2387:refnum<vi>, "Database.ActiveItemTag"=w2397:string, "cRef.Journal.References.Data"=w2391:refnum<vi>)
        n902 = property class="MCListbox (strict)"(reference=w2391, error in=w2398) -> (reference out=w2399:refnum<vi>, error out=w2393:errorcluster, "ItemNames"=w2402:string[][], "Value"=w2390:i32)
        n903 = String To Path(string=w2397) -> (path=w2400:path)
        n904 = Index Array(array=w2402, index (row)=w2390, index (col)=0 ("disabled index (col)")) -> (element=w2389:string)
        n905 = Build Path(base path=w2400, name or relative path=w2389) -> (appended path=w2395:path)
        n906 = call <vilib>:"Check if File or Folder Exists.vi"("error in (no error)"=w2393, "path"=w2395) -> ("error out"=w2392:errorcluster, "file or folder exists?"=w2394:bool)  [unwired: 7 in, 1 out]
        n907 = case shown="True" w2394 {
          tunnel: w2395 -> [_ w2418]
          tunnel: w2399 -> [_ w2415]
          tunnel: w2397 -> [_ w2407]
          tunnel: [w2404 w2412] -> w2396
          tunnel: w2392 -> [w2404 w2409]
          tunnel: w2388 -> [_ w2406]
          tunnel: w2387 -> [_ w2405]
          frame False {
          }
          frame True {
            n908 = Delete(path (use dialog)=w2418, entire hierarchy (F)=TRUE, confirm (F)=TRUE, error in=w2409) -> (deleted path=w2411:path, cancelled=w2410:bool, error out=w2414:errorcluster)  [unwired: 1 in]
            n909 = String To Path(string=w2407) -> (path=w2408:path)
            n910 = call "ListboxItems (SubVI).vi"("error in (no error)"=w2414, "MCListbox Refnum"=w2415, "path"=w2408) -> ("error out"=w2413:errorcluster)  [unwired: 2 in]
            n911 = case shown="False" w2410 {
              tunnel: w2413 -> [w2423 w2433]
              tunnel: [w2422 w2432] -> w2412
              tunnel: w2411 -> [w2424 _]
              tunnel: w2406 -> [w2420 _]
              tunnel: w2405 -> [w2419 _]
              frame False {
                n912 = Build Array(w2420, w2419) -> (w2421:refnum<vi>[])
                n913 = Path To String(path=w2424) -> (string=w2425:string)
                n914 = for {
                  tunnel: w2421 -> [w2427] mode=indexing
                  tunnel: TRUE ("Delete Children?") -> [w2431]
                  tunnel: w2425 -> [w2430]
                  tunnel: w2423 -> [w2429]
                  tunnel: [w2428] -> w2422
                  n915 = invoke class="Tree (strict)" method="Edit Tree Items.Delete"(reference=w2427, error in=w2429, "tag"=w2430, "Delete Children"=w2431) -> (error out=w2428:errorcluster)  [unwired: 1 in, 4 out]
                }
              }
              frame True {
                n916 = call <vilib>:"Clear Errors.vi"("error in (no error)"=w2433) -> ("error out"=w2432:errorcluster)  [unwired: 6 in]
              }
            }
          }
        }
      }
      frame "/*********Shutdown********/" {
      }
      frame "Error" {
        n917 = call <vilib>:"General Error Handler CORE.vi"("type of dialog (OK msg:1)"=DialogTypeEnum."auto error handling dialog", "error in (no error)"=w2443) -> ("stop event propagated"=w2440:bool, "error out"=w2436:errorcluster)  [unwired: 12 out]
        n918 = case "User Chose to Stop and Not Continue\nFALSE = Continue: CLEAR ERRORS" shown="True" w2440 {
          tunnel: [w2444 w2448] -> w2442
          tunnel: w2436 -> [w2445 w2453]
          tunnel: w2441 -> [_ w2452]
          tunnel: w2438 -> [w2446 w2455]
          tunnel: [w2446 w2454] -> w2437
          frame False {
            n919 = call <vilib>:"Clear Errors.vi"("error in (no error)"=w2445) -> ("error out"=w2444:errorcluster)  [unwired: 6 out]
          }
          frame True {
            n920 = call <vilib>:"Clear Errors.vi"("error in (no error)"=w2453) -> ("error out"=w2451:errorcluster)  [unwired: 6 out]
            n921 = Bundle By Name(cluster=w2455, "Terminate Error"=w2453) -> (w2454:T3)
            n922 = call "AMC Flush Message Queue.vi"("error in (no error)"=w2451, "Message Queue in"=w2452) -> ("error out"=w2450:errorcluster, "Message Queue out"=w2449:T6)  [unwired: 7 in]
            n923 = call "AMC Send Local Messages.vi"("error in (no error)"=w2450, "Message Names"=string[] ["Close SubVI", "Exit"], "Message Queue in"=w2449) -> ("error out"=w2448:errorcluster)  [unwired: 7 in, 1 out]
          }
        }
      }
      frame "Exit" {
        w2456 = refnum<class> refnum  # event data
        # "Don't wire 'Error In'\nMust Execute Regardless"
        n924 = Unbundle By Name(w2462) -> ("Exit Event"=w2461:T4, "Terminate Error"=w2458:errorcluster)
        n925 = Generate User Event(user event=w2461, event data cluster=w2456) -> (error out=w2460:errorcluster)  [unwired: 2 in, 1 out]
        n926 = Merge Errors(w2460, w2458, w2457) -> (w2459:errorcluster)
      }
      frame "Close SubVI" {
      }
      frame Default {
        w2468 = 1 items=["No error", "Argument error", "Memory is full", "Out of zone", "End of file", "File already open", "Generic file I/O error", "File not found", "File permission error", "Disk is full", "Duplicate path", "Too many files open", "System feature not enabled", "Resource file not found", "Cannot add resource", "Resource not found", "Image not found", "Image memory error", "Pen does not exist", "Config type invalid", "Config token not found", "Config parse error", "Config memory error", "Bad external code format", "Bad external code offset", "External code not present", "Null window", "Destroy window error", "Null menu", "Print aborted", "Bad print record", "Print driver error", "Windows error during printing", "Memory error during printing", "Print dialog error", "Generic print error", "Invalid device refnum", "Device not found", "Device parameter error", "Device unit error", "Cannot open device", "Device call aborted", "Generic error", "Cancelled by user", "Object ID too low", "Object ID too high", "Object not in heap", "Unknown heap", "Unknown object (invalid DefProc)", "Unknown object (DefProc not in table)", "Message out of range", "Invalid (null) method", "Unknown message", "Manager call not supported", "Bad address", "Network operation in progress", "Network operation timed out", "Connection is busy", "Network attribute not supported", "Network error", "Address in use", "System out of memory", "Connection aborted", "Connection refused", "Not connected", "Already connected", "Connection closed", "Initialization error (interapplication manager)", "Bad occurrence", "Wait on unbound occurrence handler", "Occurrence queue overflow", "Datalog type conflict", "Unused", "Unrecognized type (interapplication manager)", "Memory corrupt", "Failed to make temporary DLL", "Old CIN version", "Drag socket not found", "Failed to load drop-object", "Failed to register OLE object", "Failed to release OLE object", "Format specifier type mismatch", "Unknown format specifier", "Too few format specifiers", "Too many format specifiers", "Scan failed", "Newer CIN version", "Error converting to variant", "Runtime menu error", "Password tampered", "Variant attribute not found", "Incompatible variant data type", "Event data is not available", "Event Store is not present", "Occurrence is not found", "Event Queue is not created", "Event info is not available", "Refnum passed is NULL", "Error retrieving Class GUID", "Error retrieving CoClass GUID", "Error retrieving TypeLib GUID.", "Bad built application magic bytes.", "Specific driver is different from the specific driver associated with the Logical Name.", "There is no session opened to the class driver.", "Max Error", "MAX - Error with config objects", "MAX - Error loading configuration", "MAX - Group not supported"]
        w2469 = TRUE  # status
        n927 = Format Into String(format string="DEVELOPER ERROR:\nImproper State Requested\n================\nState {%s} does not exist within this architecture\n\nCheck for spelling and case errors" ("source"), w2466) -> (resulting string=w2467:string)  [unwired: 2 in, 1 out]
        n928 = Bundle By Name(cluster=w2471, "status"=w2469, "code"=w2468, "source"=w2467) -> (w2470:errorcluster)
      }
    }
    n929 = Get Date/Time In Seconds() -> (seconds since 1Jan1904=w357:timestamp)
    n930 = Get Date/Time String(seconds (now)=w357, want seconds? (F)=TRUE) -> (time string=w355:string)  [unwired: 1 in, 1 out]
    n931 = Concatenate Strings(w355, w356) -> (w354:string)
  }
  n932 = control-ref of="This VI"() -> (w2:refnum<vi>)
  n933 = call "Save Log.vi"("Array"=w1, "VI in"=w2) -> ()  [unwired: 10 in]
  n934 = while "App Close" {
    shift-right: [w2479] -> _
    shift-left: enum16{"Close Display", "Clear References"}."Close Display" -> [w2478]
    tunnel: w15 -> [w2476]
    tunnel: w17 -> [w2477]
    tunnel: [w2474] -> w11
    shift-right: [w2473] -> w10
    shift-left: w16 -> [w2475]
    i -> [w2480]
    stop <- w2481 stop-if-true
    n935 = case shown="\"Clear References\"" w2478 {
      tunnel: [w2482 w2489] -> w2474
      tunnel: [w2484 w2488] -> w2473
      tunnel: [w2483 _] -> _
      tunnel: w2477 -> [w2482 w2489]
      tunnel: w2476 -> [w2483 w2490]
      tunnel: w2475 -> [w2484 w2488]
      frame "Close Display" {
        n936 = disable-structure shown="RUN_TIME_ENGINE==True" {
          frame condition #0 (active) {
          }
          frame condition #1 {
            n937 = control-ref of="This VI"() -> (w2485:refnum<vi>)
            n938 = invoke class="VI" method="FP.Open"(reference=w2485, "Activate"=TRUE ("Activate?"), "State"=T2."Standard") -> ()  [unwired: 2 in, 5 out]
          }
        }
      }
      frame "Clear References" {
        n939 = Unbundle By Name(w2488) -> ("Exit Event"=w2491:T4)
        n940 = call "Close SubVI.vi"("SHIFTER DATA"=w2488) -> ()  [unwired: 11 in]
        n941 = Unregister For Events(event registration refnum=w2490) -> ()  [unwired: 1 in, 1 out]
        n942 = Destroy User Event(user event=w2491) -> ()  [unwired: 1 in, 1 out]
      }
    }
    n943 = call "Enum Loop Complete.vi"("Current State Enum"=w2478, "Itteration"=w2480) -> ("Loop Complete?"=w2481:bool)  [unwired: 13 out]
    n944 = Increment(x=w2478) -> (x+1=w2479:enum16{"Close Display", "Clear References"})
  }
  n945 = disable-structure shown="RUN_TIME_ENGINE==True" {
    disable-tunnel: [w2492 w2493] -> w9
    disable-tunnel: w11 -> [w2492 w2493]
    frame condition #0 (active) {
    }
    frame condition #1 {
      n946 = Quit LabVIEW() -> ()  [unwired: 1 in]
    }
  }
  n947 = Unbundle By Name(w10) -> ("Terminate Error"=w8:errorcluster)
  n948 = Merge Errors(w8, w9) -> (w4:errorcluster)
  n949 = call <vilib>:"Clear Errors.vi"("error in (no error)"=w4) -> ()  [unwired: 6 in, 1 out]
